vi "2D scan Tclk.vi"(0 "ActiveX Container":refnum<k7>(container), 1 "Det Info":T11={"Brightness A"=40.0, "Contrast A"=26.0, "Detector B name"="ESB @ 1.0 kV", "Brightness B"=40.0, "Contrast B"=40.0, "Detector C name"="PMT @ 6.0", "Detector D name"="Detector D"}, 2 "HW Config":T12={"SEM X coil"="SEM-X", "SEM Y coil"="SEM-Y", "Detectors"="Detectors", "Det min (V)"=-10.0, "Det max (V)"=10.0, "Eanable COM"=TRUE, "COM port"="COM1", "Detector FIB-NI auto switch"="FIB/port0/line0", "Machine Type"=0, "Machine ID"="", "SEM Max FOV (um)"=350.0} {"Machine Type" items=["Feiss", "NVision"]}, 3 "Scan Para":T10={"X resolution"=4096, "Y resolution"=2048, "X center (um)"=0.0, "Y center (um)"=0.0, "X size (V)"=20.0, "X size auto"=TRUE, "X stig"=0.0, "Y stig"=0.0, "X aln"=0.0, "Y aln"=0.0, "Scan rate (Hz)"=10000000, "Oversampling"=10, "Oversampling auto"=TRUE, "Frame line rampdown ratio"=0.1, "Pixel size (nm)"=5.0, "WD"=4.0} {"WD" format="%#_7g"; "Frame line rampdown ratio" min=-1 max=1 step=0.05 format="%.2g"; "Scan rate (Hz)" max=4000000 format="%.2e"}, 4 "Focus Index Options":T2={"Keep aspect ratio"=FALSE, "X Grids"=1, "Y Grids"=1, "Primary X index"=1, "Primary Y index"=1}, 5 "File Info":T8={"File path"=path "E:/Images", "Notes"="", "Save recipe"=FALSE, "Load recipe"=FALSE, "Sample ID"=""}, 6 "Options":T9={"GetInfo"=TRUE, "Set Det A para"=TRUE, "Set WD"=FALSE, "Set Mag"=TRUE, "Set stig"=FALSE, "Set aln"=FALSE, "Display"=TRUE, "Save"=TRUE, "8-bit"=TRUE, "Detector A"=TRUE, "Detector B"=TRUE, "Detector C"=FALSE, "Detector D"=FALSE, "Inverse A"=FALSE, "Inverse B"=FALSE, "Inverse C"=FALSE, "Inverse D"=FALSE, "Inverse PNG"=FALSE, "Freeze"=TRUE, "PNG only"=FALSE, "Upload"=FALSE, "Delete after upload"=FALSE}, 7 "WatchDog Mode":u16(ring)=2 items=["Do Nothing", "Send Idle Only", "Watch FIB & SEM", "Watch FIB Only", "Watch SEM Only"], 9 "Additional Info":cluster{"Restart flag":u8, "Stage move flag":u8}, 10 "Frame":u8=1 min=1 step=1, 11 "Tile index":u8[](array[numeric])=[0, 0], 13 "Milling para":T1={"X resolution"=4096, "Y resolution"=125001, "X offset (um)"=0.0, "Y offset (um)"=0.0, "X center (um)"=0.0, "Y center (um)"=0.0, "X size (um)"=250.0, "Y size (um)"=250.0, "UL-Ang"=90.0, "UR-Ang"=90.0, "Line milling time (s)"=5.0, "Z-step (nm)"=2.0, "Lines auto pause"=1, "Auto pause"=FALSE, "Mill from Bottom"=FALSE, "FIB FOV (um)"=500.0, "Auto Profile"=FALSE, "Mill start from Last"=FALSE, "FIB PID on"=FALSE, "FIB PID reset"=TRUE, "FIB PID measured"=0, "FIB PID target"=0.0, "FIB PID target slope"=0.0, "FIB PID P"=0.001, "FIB PID I"=0.01, "FIB PID D"=0.0, "Emission (uA)"=1.36, "Suppressor (V)"=50.0, "Auto reheat"=FALSE} caption="Milling Parameters" {"Suppressor (V)" step=0.1 format="%.1g"; "Emission (uA)" step=0.1 format="%.2g"; "FIB PID measured" items=["Spec.", "B.D. 1", "B.D. 2", "Mill", "Spec. +"]; "FIB PID target slope" min=-1 max=1 step=0.1; "UR-Ang" format="%.2f"; "UL-Ang" format="%.2f"; "Y offset (um)" step=0.02 format="%.3g"; "X offset (um)" step=1 format="%.3g"; "FIB FOV (um)" format="%.3g"; "Line milling time (s)" format="%.1f"; "Y center (um)" format="%#.3g"; "X center (um)" format="%#.3g"}) -> (12 "Image Focus Index Array":T3, 14 "Info & Status":T7={"AO SampClk.MaxRate"=100000000.0, "AI SampClk.MaxRate"=100000000.0, "AO rate"=10000000.0, "Scan speed"=1, "Detector number"=2, "X min (V)"=-10.0, "X max (V)"=10.0, "X min index"=0, "X max index"=4095, "AO multiline"=128, "Decimating factor"=8, "AvailSampPerChan"=6177088, "AO scan line"=2048, "Total pixels recorded"=8388608, "Total lines scanned"=2048, "Scan time (m)"=0.0, "Scan time (s)"=0.9240575999999999, "Remaining time (m)"=0, "Remaining time (s)"=0, "Specimen I (nA)"=0.0, "Frame"=1, "X tile"=0, "Y tile"=0} {"Frame" min=1 step=1; "Y tile" min=1; "X tile" min=1; "Specimen I (nA)" format="%#.2g"; "AvailSampPerChan" scale=0.0..32000000.0; "Scan time (s)" format="%.3f"; "Total pixels recorded" scale=0.0..250000.0; "Scan speed" scale=1.0..15.0; "AO rate" format="%#_3e"}, 15 "SEM parameters":T5={"Detector A"="Det A", "Detector B"="ESB @ 1.0 kV", "Brightness A"=40.0, "Contrast A"=26.0, "Brightness B"=40.0, "Contrast B"=40.0, "Magnification"=5582.6, "Pixel size"=5.0, "Working distance"=4.0, "EHT"=0.0, "Aperture"=0, "High current mode"=0, "Probe current"=0.0, "Scan rotation"=0.0, "Chamber vac"=0.0, "Gun vac"=0.0, "Beam shift X"=0.0, "Beam shift Y"=0.0, "Stig X"=0.0, "Stig Y"=0.0, "Alignment X"=0.0, "Alignment Y"=0.0, "Stage X"=0.0, "Stage Y"=0.0, "Stage Z"=0.0, "Stage T"=0.0, "Stage R"=0.0, "Stage M"=0.0}, 17 "8-bit over scale":bool[](array[boolean]), 18 "FIB parameters":T6, 19 "Image Focus Index":T4)   [LabVIEW 2018]
uses:
  <vilib>/Utility/error.llb/DialogType.ctl
  <vilib>/DAQmx/write.llb/DAQmx Write (Digital Bool 1Line 1Point).vi
  <vilib>/Analysis/2dsp.llb/Decimate (single shot, DBL).vi
  <vilib>/DAQmx/create/channels.llb/DAQmx Create Channel (DO-Digital Output).vi
  <vilib>/DAQmx/miscellaneous.llb/DAQmx Fill In Error Info.vi
  <instrlib>/niScope/Acquire/niScope Get Scaling Coefficients.vi
  <instrlib>/niScope/Acquire/Fetch/niScope Multi Fetch Binary 16.vi
  <vilib>/measure/madcrms.llb/Basic Averaged DC-RMS for 1 Chan.vi
  <instrlib>/niFgen/niFgen.llb/niFgen Write Waveform.vi
  <vilib>/regexp/Match Regular Expression.xnode
  <vilib>/Analysis/NI_AALPro.lvlib
  <vilib>/measure/NI_MAPro.lvlib
panel:
  out "First pixel Y":i32
  out "First pixel X":i32
  out "Stage move flag":u8
  out "Restart flag":u8
  out "AI multiline":u16
  out "Total pixels":u32
  in  "Force tclk init":bool
  out "DetB-Scaling":sgl
  out "DetA-Scaling":sgl
  out "DetB-Rate":sgl
  out "DetA-Rate":sgl
  out "8-bit coefficents":sgl[][](array[numeric])
  out "DetB-k":sgl
  out "DetB-Io":sgl
  out "DetA-k":sgl
  out "DetA-Io":sgl
  out "8-bit":bool=TRUE
  out "Screen pixel factor":dbl=0.25
  out "Mag":dbl=5582.6
  out "Runsheet header array":string[](array[string])=["Date", "Time", "Notes", "Detector A", "Detector B", "Detector C", "Detector D", "Detectors", "X resolution", "Y resolution", "Rate (Hz)", "Brightness A (%)", "Contrast A (%)", "Brightness B (%)", "Contrast B (%)", "Magnification", "Pixel size (nm)", "Working Distance (mm)", "EHT (kV)", "Aperture #", "High Current Mode", "Probe Current (A)", "Beam Shift X", "Beam Shift Y", "Stigmation X", "Stigmation Y", "Alignment X", "Alignment Y", "FIB spacing (nm)", "A Img Focus Index", "B Img Focus Index", "C Img Focus Index", "D Img Focus Index", "Temp (F)", "FIB Faraday Cup (nA)", "Specimen I (nA)", "Milling Beam Dump (nA)", "Milling Y voltage (V)", "SEM Specimen I (nA)", "Image Delta X (pix)", "Image Delta Y (pix)", "Image Delta Z"]
  out "Set aln":bool
  out "X aln":sgl
  out "Y aln":sgl
  out "FI scaling":u8=1
  in  "SEM Spec. I (nA)":sgl format="%#.2g"
  out "SW date":string
  out "Image bits":u8=16
  out "error out":errorcluster
  out "Delete after upload":bool
  in  "FI Detector":u16(ring) caption="Detector" items=["A", "B", "C", "D"]
  out "keep aspect ratio":bool=TRUE
  out "Primary Y index":u8 caption="Primary Y"
  out "Primary X index":u8 caption="Primary X"
  out "Y Grids":u8=1
  out "X Grids":u8=1
  out "Timestamp":timestamp=timestamp(3479292891.7167473 s since 1904-01-01)
  out "Upload flags path":path
  out "Upload":bool=TRUE
  out "Sample ID":string
  out "Machine ID":string
  out "Eanable COM":bool
  out "PNG only":bool=TRUE
  out "Eval B":i16[][](graph)
  out "Eval A":i16[][](graph)
  out "Freeze":bool=TRUE
  out "Detector FIB-NI auto switch":tag="FIB/port0/line0"
  out "GetInfo":bool=TRUE
  out "Set stig":bool
  out "Y stig":sgl
  out "X stig":sgl
  in  "Total time":dbl=0.9240575999999999
  in  "stop":bool=TRUE
  out "Det max (V)":dbl=10.0
  out "Det min (V)":dbl=-10.0
  in  "AvailSampPerChan":u32(slide)=6177088 scale=0.0..1000000.0
  in  "AO scan line":u32=2048
  in  "AO multiline":u32=128
  in  "Decimating factor":u16=8
  in  "Remaining time (m)":u16
  in  "Remaining time (s)":u8
  in  "Scan time (s)":dbl=0.9240575999999999 format="%.3f"
  in  "Scan time (m)":dbl
  in  "Total lines scanned":i32=2048
  in  "Total pixels recorded":i32(slide)=8388608 scale=-1.0..1048576.0
  in  "X max (V)":dbl=10.0
  in  "X min (V)":dbl=-10.0
  in  "X min index":i32
  in  "X max index":i32=4095
  in  "Scan speed":u8(slide)=1 scale=1.0..15.0
  in  "AO rate":dbl=10000000.0 caption="Scanning rate" format="%#_3e"
  in  "Detector number":u8=2
  in  "AI SampClk.MaxRate":dbl=100000000.0
  in  "AO SampClk.MaxRate":dbl=100000000.0
  out "Det A Img":i16[][](graph)
  out "Det B Img":i16[][](graph)
  out "Notes":string
  out "File path":path=path "E:/Images"
  out "Inverse PNG":bool
  out "Inverse D":bool
  out "Inverse C":bool
  out "Inverse B":bool
  out "Inverse A":bool
  out "Detector D":bool
  out "Detector C":bool
  out "Detector B":bool=TRUE
  out "Detector A":bool=TRUE
  out "Save":bool=TRUE
  out "Display":bool=TRUE
  out "Set Mag":bool=TRUE
  out "Set WD":bool
  out "Set Det A para":bool=TRUE
  out "WD":sgl=4.0
  out "Pixel size (nm)":sgl=5.0
  out "Frame line rampdown ratio":sgl=0.1
  out "Oversampling":u32=10
  out "Scan rate (Hz)":u32=10000000
  out "Y resolution":u32=2048
  out "X resolution":u32=4096
  out "Detector D name":string="Detector D"
  out "Detector C name":string="PMT @ 6.0"
  out "Contrast B":dbl=40.0
  out "Brightness B":dbl=40.0
  out "Detector B name":string="ESB @ 1.0 kV"
  out "Contrast A":dbl=26.0
  out "Brightness A":dbl=40.0
  out "COM port":refnum<visa-resource-name>="COM1"
  out "File name":path=path "E:/Images/Y2014/M04/D02/_14-04-02_091451_0-0.dat"
  # "Hardware Configuration"
  # "Detectors Information"
  # "Scanning Parameters"
  # "Direction"
  # "Start\nfrom"
  # "<"
  # "Hz"
  # "Scanning time"
  # "m"
  # "s"
  # "Remaining time"
  # "m"
  # "s"
  # "Det"
  # "Detector A"
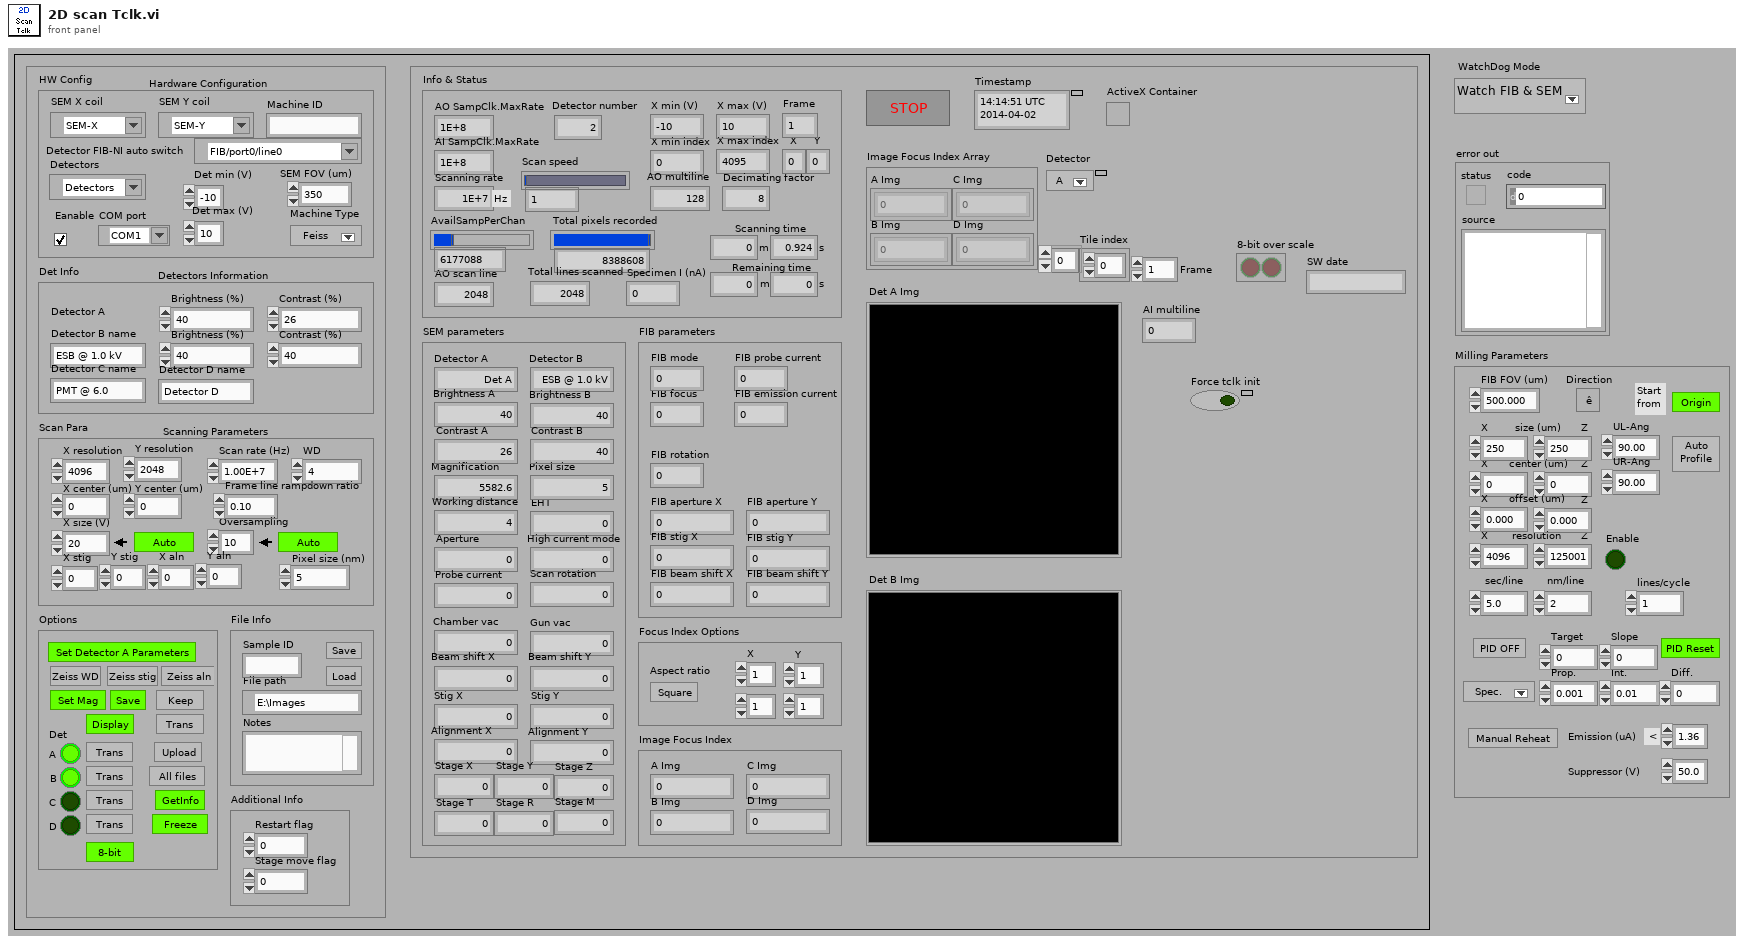
[diagram p1: front panel]
types:
  T1 = cluster{"X resolution":u32, "Y resolution":u32, "X offset (um)":sgl, "Y offset (um)":sgl, "X center (um)":sgl, "Y center (um)":sgl, "X size (um)":sgl, "Y size (um)":sgl, "UL-Ang":sgl, "UR-Ang":sgl, "Line milling time (s)":sgl, "Z-step (nm)":dbl, "Lines auto pause":u16, "Auto pause":bool, "Mill from Bottom":bool, "FIB FOV (um)":sgl, "Auto Profile":bool, "Mill start from Last":bool, "FIB PID on":bool, "FIB PID reset":bool, "FIB PID measured":u8, "FIB PID target":sgl, "FIB PID target slope":sgl, "FIB PID P":sgl, "FIB PID I":sgl, "FIB PID D":sgl, "Emission (uA)":dbl, "Suppressor (V)":sgl, "Auto reheat":bool}
  T2 = cluster{"Keep aspect ratio":bool, "X Grids":u8, "Y Grids":u8, "Primary X index":u8, "Primary Y index":u8}
  T3 = cluster{"A Img Focus Index array":sgl[][], "B Img Focus Index array":sgl[][], "C Img Focus Index array":sgl[][], "D Img Focus Index array":sgl[][]}
  T4 = cluster{"A Img Focus Index":sgl, "B Img Focus Index":sgl, "C Img Focus Index":sgl, "D Img Focus Index":sgl}
  T5 = cluster{"Detector A":string, "Detector B":string, "Brightness A":sgl, "Contrast A":sgl, "Brightness B":sgl, "Contrast B":sgl, "Magnification":sgl, "Pixel size":sgl, "Working distance":sgl, "EHT":sgl, "Aperture":u8, "High current mode":u8, "Probe current":sgl, "Scan rotation":sgl, "Chamber vac":sgl, "Gun vac":sgl, "Beam shift X":sgl, "Beam shift Y":sgl, "Stig X":sgl, "Stig Y":sgl, "Alignment X":sgl, "Alignment Y":sgl, "Stage X":sgl, "Stage Y":sgl, "Stage Z":sgl, "Stage T":sgl, "Stage R":sgl, "Stage M":sgl}
  T6 = cluster{"FIB mode":u8, "FIB focus":sgl, "FIB probe current":sgl, "FIB emission current":sgl, "FIB rotation":sgl, "FIB aperture X":sgl, "FIB aperture Y":sgl, "FIB stig X":sgl, "FIB stig Y":sgl, "FIB beam shift X":sgl, "FIB beam shift Y":sgl}
  T7 = cluster{"AO SampClk.MaxRate":dbl, "AI SampClk.MaxRate":dbl, "AO rate":dbl, "Scan speed":u8, "Detector number":u8, "X min (V)":dbl, "X max (V)":dbl, "X min index":i32, "X max index":i32, "AO multiline":u32, "Decimating factor":u16, "AvailSampPerChan":u32, "AO scan line":u32, "Total pixels recorded":i32, "Total lines scanned":i32, "Scan time (m)":dbl, "Scan time (s)":dbl, "Remaining time (m)":u16, "Remaining time (s)":u8, "Specimen I (nA)":sgl, "Frame":u8, "X tile":u8, "Y tile":u8}
  T8 = cluster{"File path":path, "Notes":string, "Save recipe":bool, "Load recipe":bool, "Sample ID":string}
  T9 = cluster{"GetInfo":bool, "Set Det A para":bool, "Set WD":bool, "Set Mag":bool, "Set stig":bool, "Set aln":bool, "Display":bool, "Save":bool, "8-bit":bool, "Detector A":bool, "Detector B":bool, "Detector C":bool, "Detector D":bool, "Inverse A":bool, "Inverse B":bool, "Inverse C":bool, "Inverse D":bool, "Inverse PNG":bool, "Freeze":bool, "PNG only":bool, "Upload":bool, "Delete after upload":bool}
  T10 = cluster{"X resolution":u32, "Y resolution":u32, "X center (um)":sgl, "Y center (um)":sgl, "X size (V)":dbl, "X size auto":bool, "X stig":sgl, "Y stig":sgl, "X aln":sgl, "Y aln":sgl, "Scan rate (Hz)":u32, "Oversampling":u32, "Oversampling auto":bool, "Frame line rampdown ratio":sgl, "Pixel size (nm)":sgl, "WD":sgl}
  T11 = cluster{"Brightness A":dbl, "Contrast A":dbl, "Detector B name":string, "Brightness B":dbl, "Contrast B":dbl, "Detector C name":string, "Detector D name":string}
  T12 = cluster{"SEM X coil":refnum<k15>, "SEM Y coil":refnum<k15>, "Detectors":refnum<k15>, "Det min (V)":dbl, "Det max (V)":dbl, "Eanable COM":bool, "COM port":refnum<visa-resource-name>, "Detector FIB-NI auto switch":tag, "Machine Type":u8, "Machine ID":string, "SEM Max FOV (um)":sgl}
  T13 = cluster{"AO SampClk.MaxRate":dbl, "AI SampClk.MaxRate":dbl, "AO rate":dbl, "Scan speed":u8, "Detector number":u8, "X min (V)":dbl, "X max (V)":dbl, "X min index":i32, "X max index":i32, "AO multiline":u32, "Decimating factor":u16, "AvailSampPerChan":u32, "AO scan line":u32, "Total pixels recorded":i32, "Total lines scanned":i32, "Scan time (m)":dbl, "Scan time (s)":dbl, "Remaining time (m)":u16, "Remaining time (s)":u8, "SEM Spec. I (nA)":sgl, "Frame":u8, u8, u8}
  T14 = enum16{"SEM", "FIB", "Milling", "SEM + FIB", "Mill + SEM", "SEM Drift Correction", "FIB Drift Correction", "No Beam", "External", "External + SEM"}
  T15 = enum16{"Initialize Reference", "Get Reference", "Close Reference"}
  T16 = enum16{"open", "replace", "create", "open or create", "replace or create", "replace or create with confirmation"}
  T17 = typedef "DialogType.ctl" = u16
  T18 = cluster{"FIB mode":u8, "FIB focus":sgl, "FIB probe current":u8, "FIB emission current":sgl, "FIB rotation":sgl, "FIB aperture X":sgl, "FIB aperture Y":sgl, "FIB stig X":sgl, "FIB stig Y":sgl, "FIB beam shift X":sgl, "FIB beam shift Y":sgl}
  T19 = cluster{"Latest 8-bit coefficients[0]":sgl, "Latest 8-bit coefficients[1]":sgl, "Latest 8-bit coefficients[2]":sgl, "Latest 8-bit coefficients[3]":sgl, "Latest 8-bit coefficients[4]":sgl, "Latest 8-bit coefficients[5]":sgl, "Latest 8-bit coefficients[6]":sgl, "Latest 8-bit coefficients[7]":sgl}
  T20 = cluster{"sessions out":refnum<k20>[], "SEM-X handle out":refnum<k15>, "SEM-Y handle out":refnum<k15>, "SEM-Y waveform handle out":i32, "Detectors handle out":refnum<k15>, "channels":string, "error out":errorcluster, "Others":cluster{"AO SampClk.MaxRate":dbl, "AI SampClk.MaxRate":dbl, "AO rate":dbl, "Scan speed":u8, "Detector number":u8, "X min (V)":dbl, "X max (V)":dbl, "X min index":i32, "X max index":i32, "Y min (V)":dbl, "Y max (V)":dbl, "AO multiline":u32, "Decimating factor":u16, "Total time":dbl, "Scan time (m)":dbl, "Scan time (s)":dbl, "X resolution":u32, "Y resolution":u32, "X resolution with rampdown":i32, "Oversampling":u32, "Y scan pts per line":i32, "Y scan pts per AO multiline":i32, "Small scan":bool, "Y single line pattern":dbl[], "Detectors min record length":u32, "Waveform blocks":u32, "Repeat count":u32, "Waveform size":u32, "AI multiline":u16}}
  T21 = cluster{"offset":dbl, "gain":dbl, "reserved 1":dbl, "reserved 2":dbl}[]
  T22 = cluster{"offset":sgl, "gain":sgl, "reserved 1":sgl, "reserved 2":sgl}[]
  T23 = cluster{"Detector A":bool, "Detector B":bool, "Detector C":bool, "Detector D":bool}
  T24 = cluster{"Detector C name":string, "Detector D name":string}
  T25 = cluster{"X resolution":u32, "Y resolution":u32, "Oversampling":u32, "Scan speed":u8, "AO rate":dbl, "Frame line rampdown ratio":sgl, "X min (V)":dbl, "X max (V)":dbl, "Det min (V)":dbl, "Det max (V)":dbl}
  T26 = cluster{"X resolution":u32, "Y resolution":u32, "X index":u32[], "Y index":u32[], "X length":u32, "Y length":u32}
  T27 = cluster{"A Img Focus Index array":dbl[][], "B Img Focus Index array":dbl[][], "C Img Focus Index array":dbl[][], "D Img Focus Index array":dbl[][]}
  T28 = cluster{"A Img Focus Index":dbl, "B Img Focus Index":dbl, "C Img Focus Index":dbl, "D Img Focus Index":dbl}
  T29 = cluster{"Single":sgl, "Single":sgl, "Single":sgl, "Single":sgl, "Single":sgl, "Single":sgl, "SEM Spec. I (nA)":sgl, "Single":sgl, "D Img Focus Index":dbl, "UInt32":u32}
  T30 = cluster{dbl, "8-bit":bool, "8-bit coefficents":sgl[][], "Restart flag":u8, "Stage move flag":u8, "First pixel X":i32, "First pixel Y":i32, cluster{"Detector A":bool, "Detector B":bool, "Detector C":bool, "Detector D":bool}, cluster{"X resolution":u32, "Y resolution":u32, "Oversampling":u32, "Scan speed":u8, "AO rate":dbl, "Frame line rampdown ratio":sgl, "X min (V)":dbl, "X max (V)":dbl, "Det min (V)":dbl, "Det max (V)":dbl}, "Decimating factor":u16, "Sample ID":string, "Notes":string, cluster{"Detector C name":string, "Detector D name":string}, "SEM parameters":cluster{"Detector A":string, "Detector B":string, "Brightness A":sgl, "Contrast A":sgl, "Brightness B":sgl, "Contrast B":sgl, "Magnification":sgl, "Pixel size":sgl, "Working distance":sgl, "EHT":sgl, "Aperture":u8, "High current mode":u8, "Probe current":sgl, "Scan rotation":sgl, "Chamber vac":sgl, "Gun vac":sgl, "Beam shift X":sgl, "Beam shift Y":sgl, "Stig X":sgl, "Stig Y":sgl, "Alignment X":sgl, "Alignment Y":sgl, "Stage X":sgl, "Stage Y":sgl, "Stage Z":sgl, "Stage T":sgl, "Stage R":sgl, "Stage M":sgl}, "FIB parameters":cluster{"FIB mode":u8, "FIB focus":sgl, "FIB probe current":sgl, "FIB emission current":sgl, "FIB rotation":sgl, "FIB aperture X":sgl, "FIB aperture Y":sgl, "FIB stig X":sgl, "FIB stig Y":sgl, "FIB beam shift X":sgl, "FIB beam shift Y":sgl}, "Milling para":cluster{"X resolution":u32, "Y resolution":u32, "X offset (um)":sgl, "Y offset (um)":sgl, "X center (um)":sgl, "Y center (um)":sgl, "X size (um)":sgl, "Y size (um)":sgl, "UL-Ang":sgl, "UR-Ang":sgl, "Line milling time (s)":sgl, "Z-step (nm)":dbl, "Lines auto pause":u16, "Auto pause":bool, "Mill from Bottom":bool, "FIB FOV (um)":sgl, "Auto Profile":bool, "Mill start from Last":bool, "FIB PID on":bool, "FIB PID reset":bool, "FIB PID measured":u8, "FIB PID target":sgl, "FIB PID target slope":sgl, "FIB PID P":sgl, "FIB PID I":sgl, "FIB PID D":sgl, "Emission (uA)":dbl, "Suppressor (V)":sgl, "Auto reheat":bool}, "Machine ID":string, cluster{"Single":sgl, "Single":sgl, "Single":sgl, "Single":sgl, "Single":sgl, "Single":sgl, "SEM Spec. I (nA)":sgl, "Single":sgl, "D Img Focus Index":dbl, "UInt32":u32}}
  T31 = typedef "imagedata.ctl" = cluster{"image type":i32, "image depth":i32, "image":u8[], "mask":u8[], "colors":u32[], "Rectangle":cluster{"left":i16, "top":i16, "right":i16, "bottom":i16}}
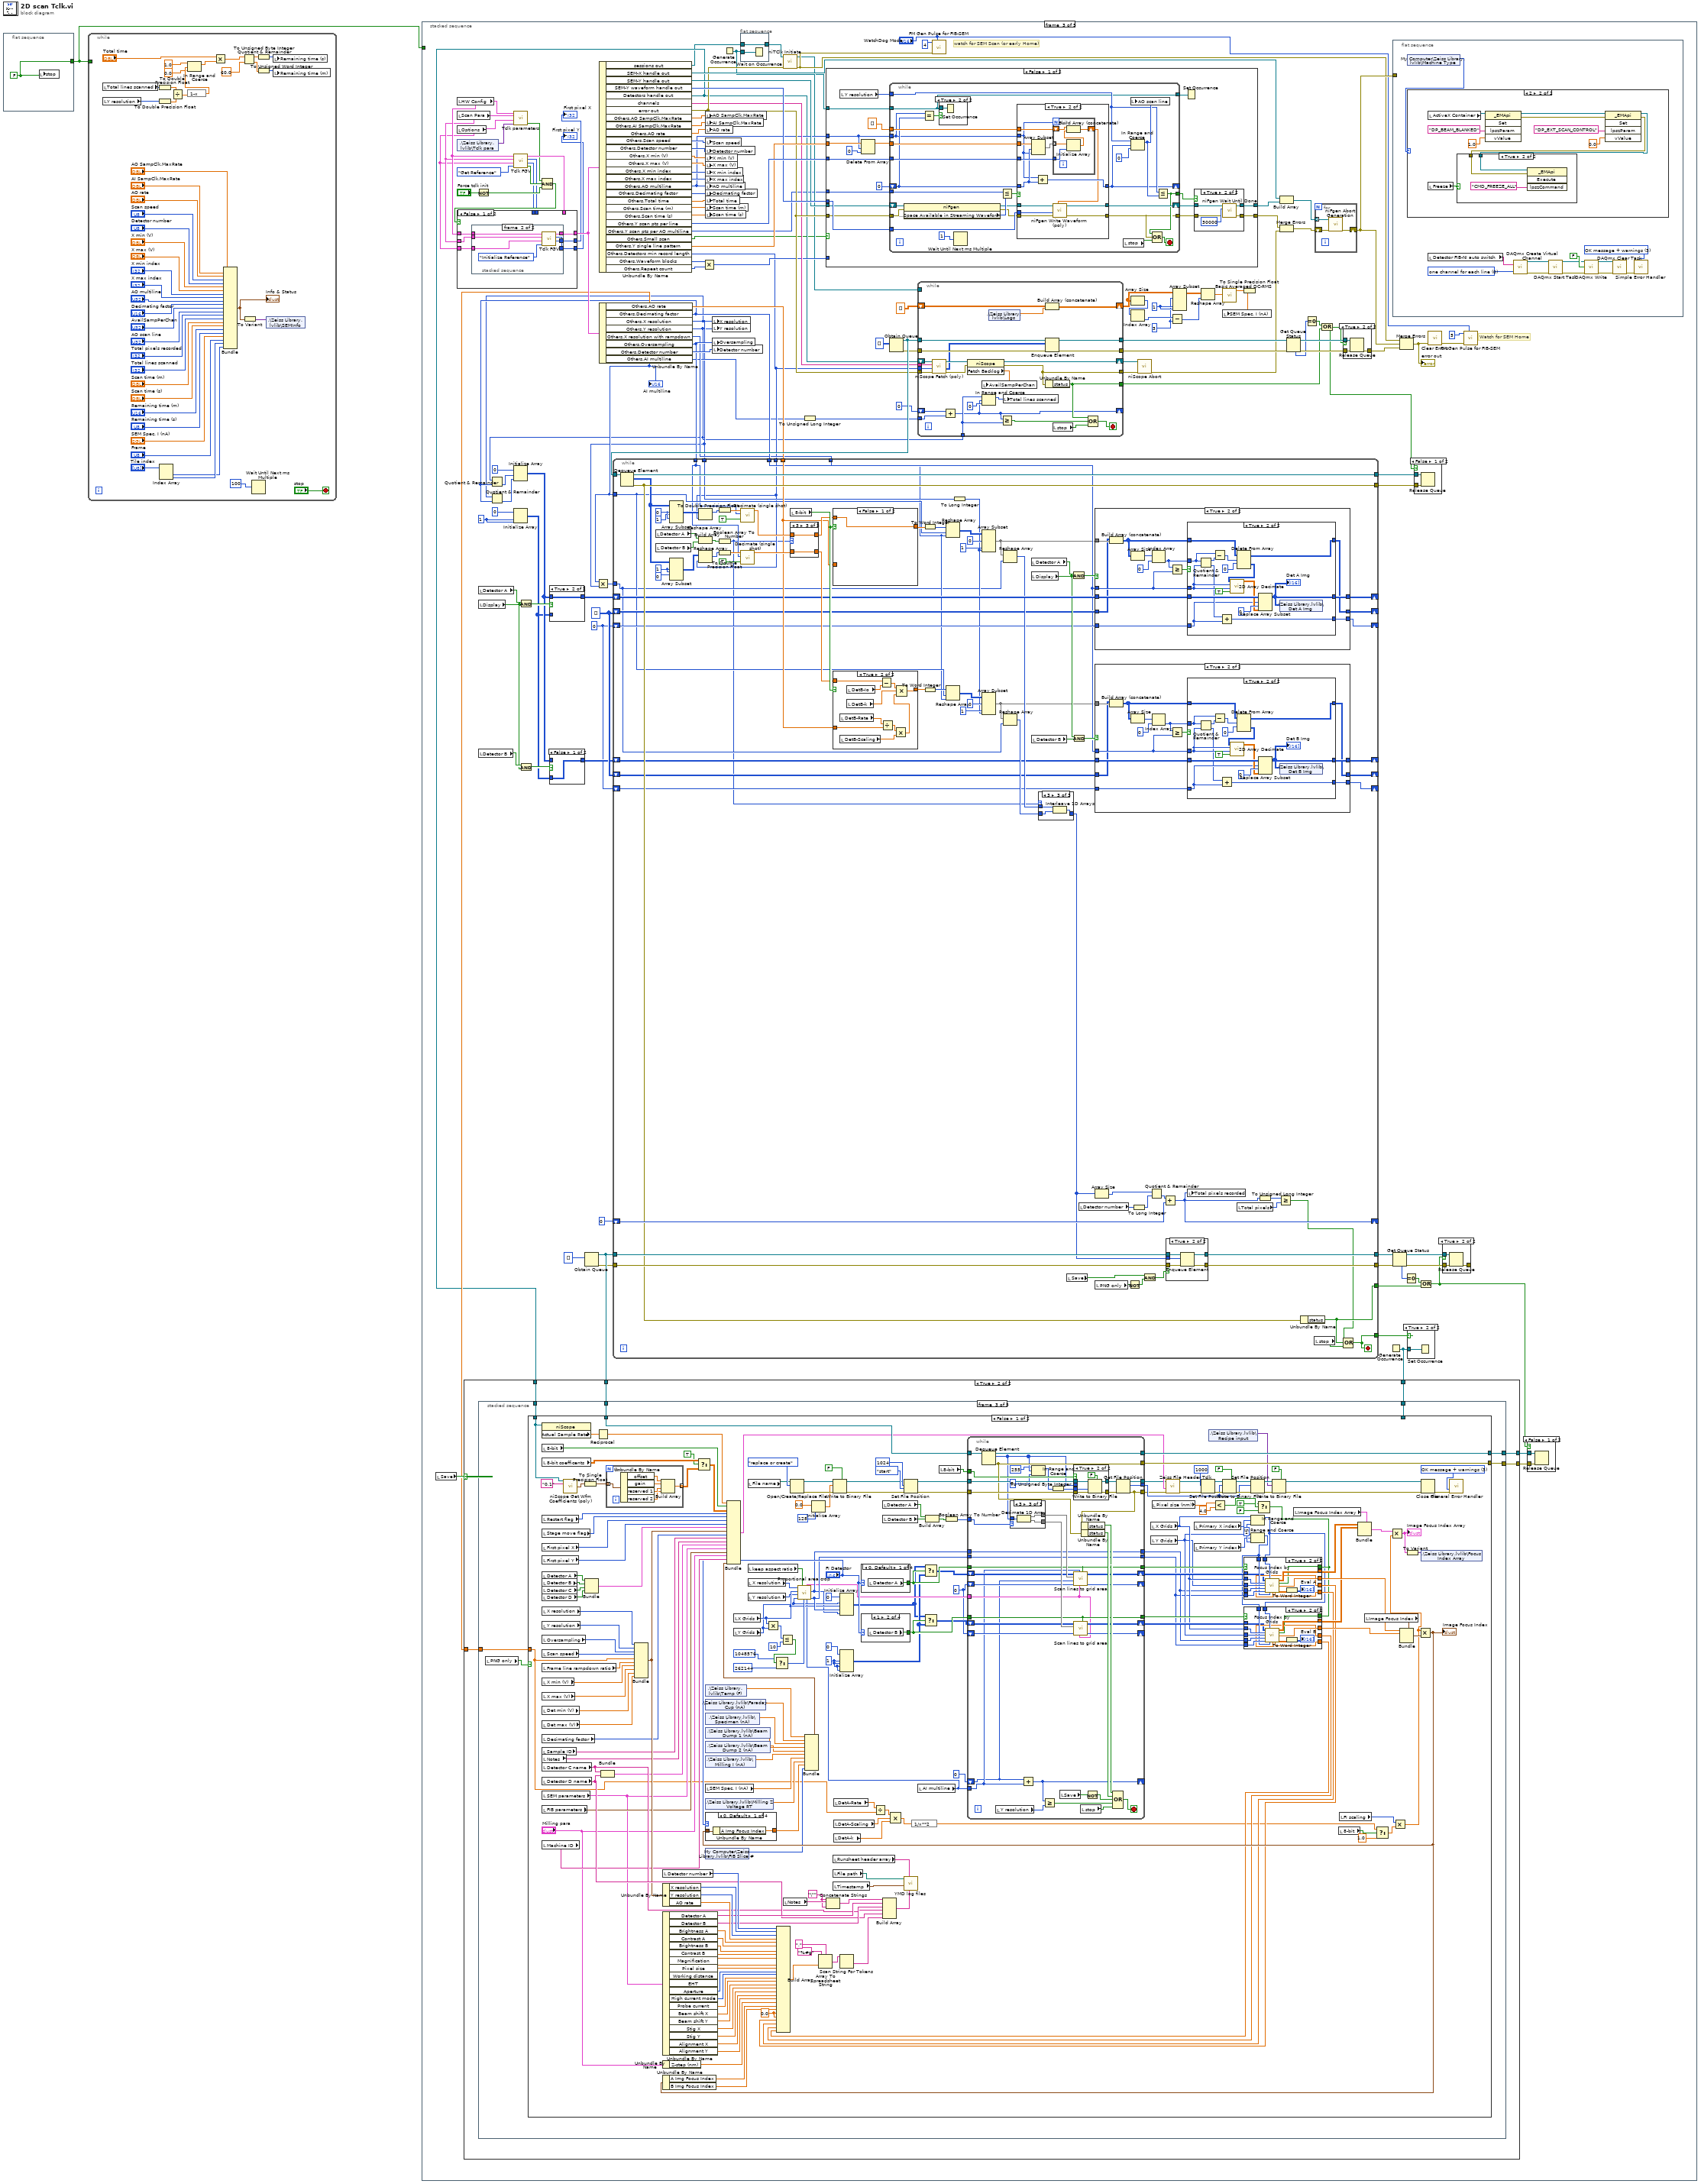
[diagram p0: block diagram]
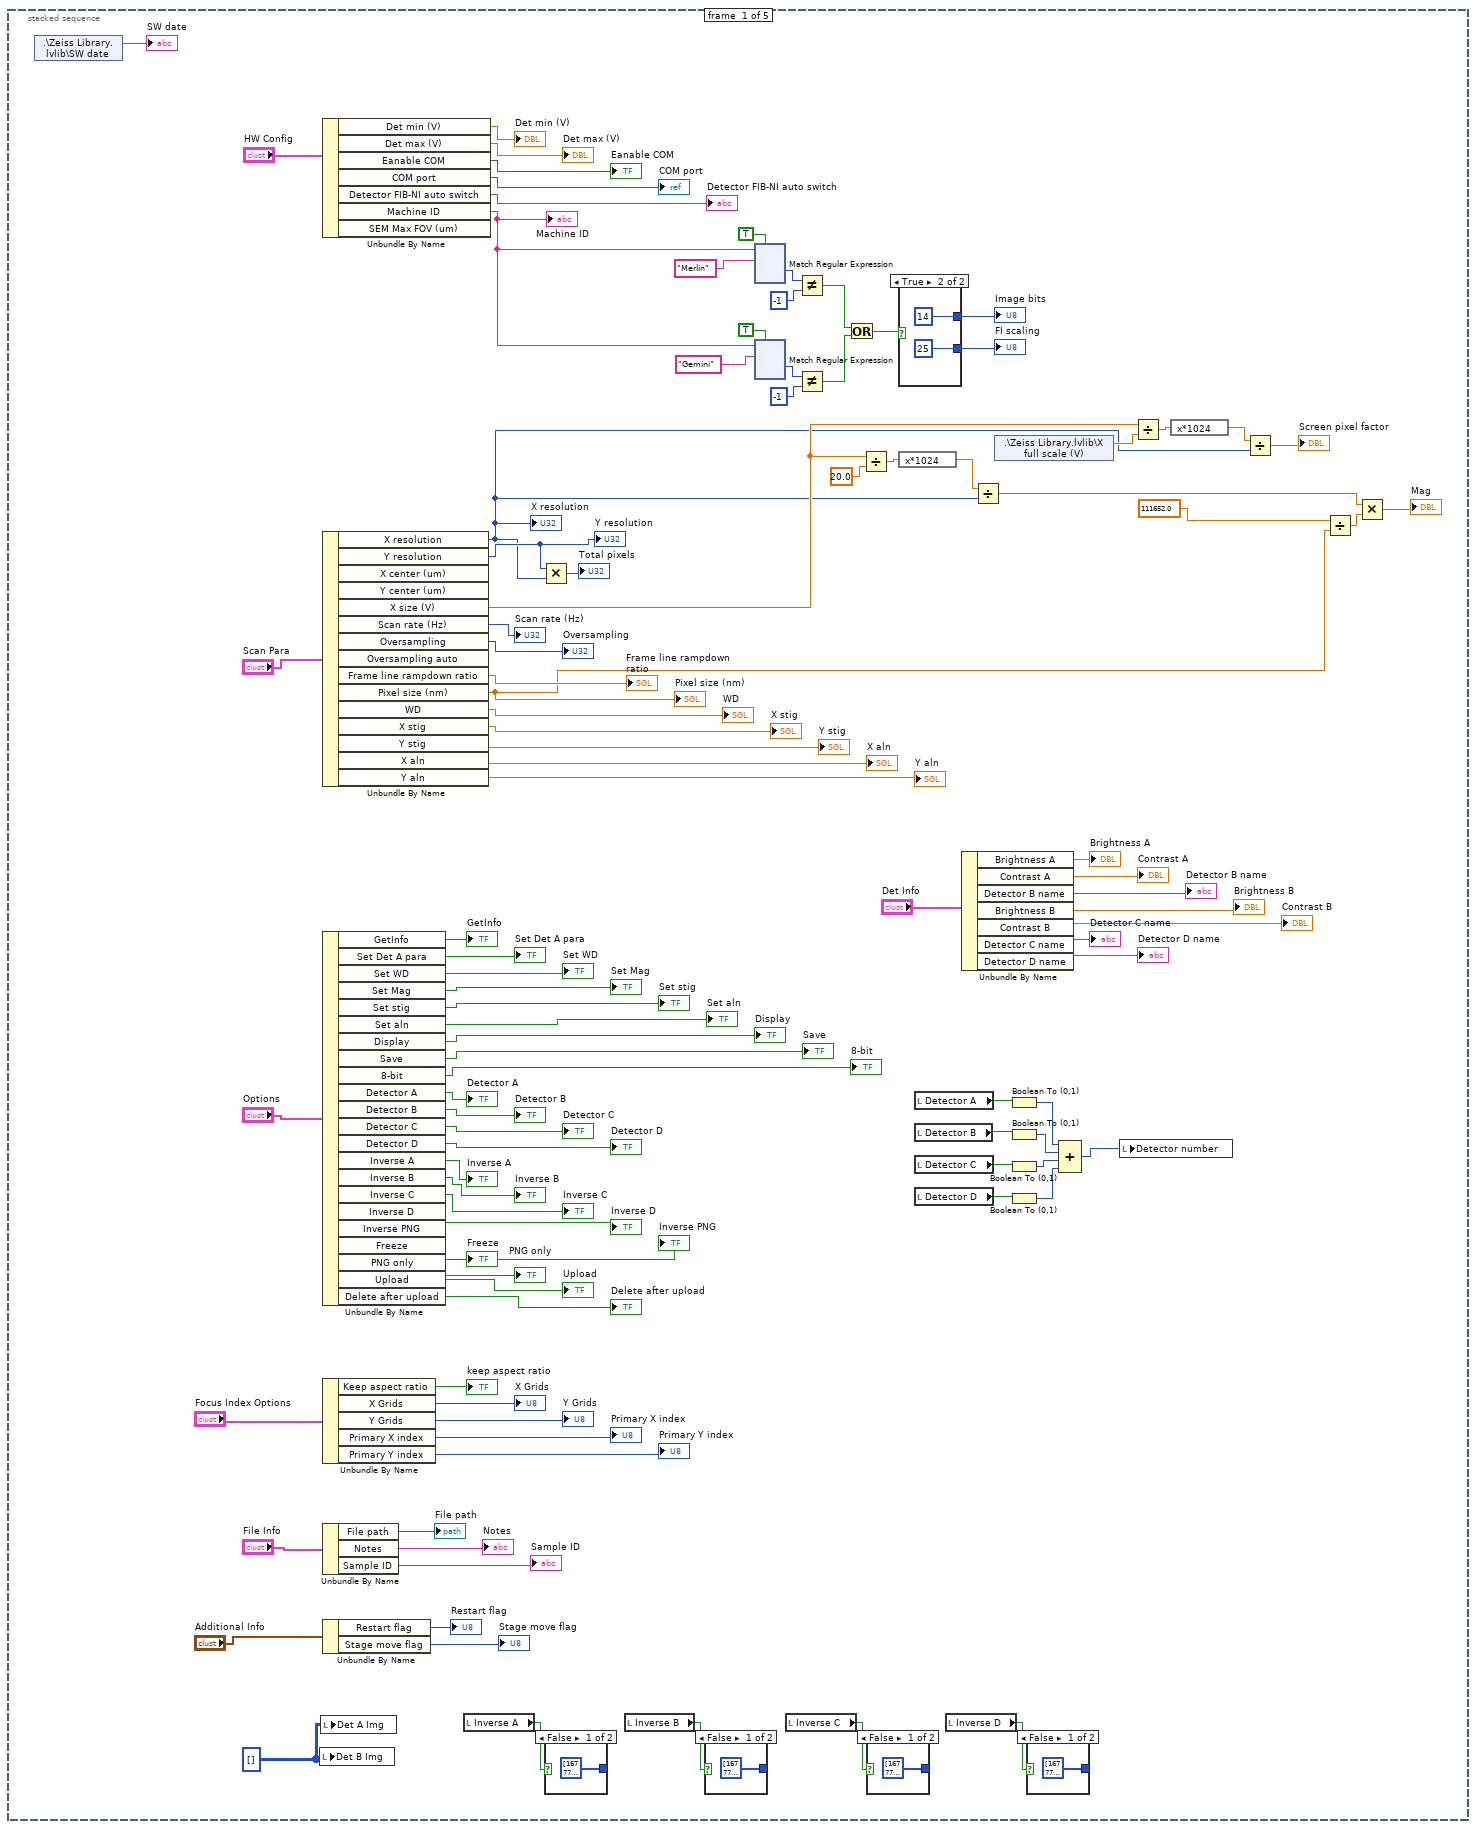
[diagram p2: hidden frame]
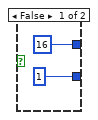
[diagram p3: hidden frame]
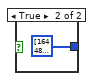
[diagram p4: hidden frame]
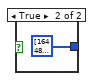
[diagram p5: hidden frame]
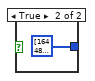
[diagram p6: hidden frame]
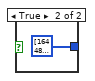
[diagram p7: hidden frame]
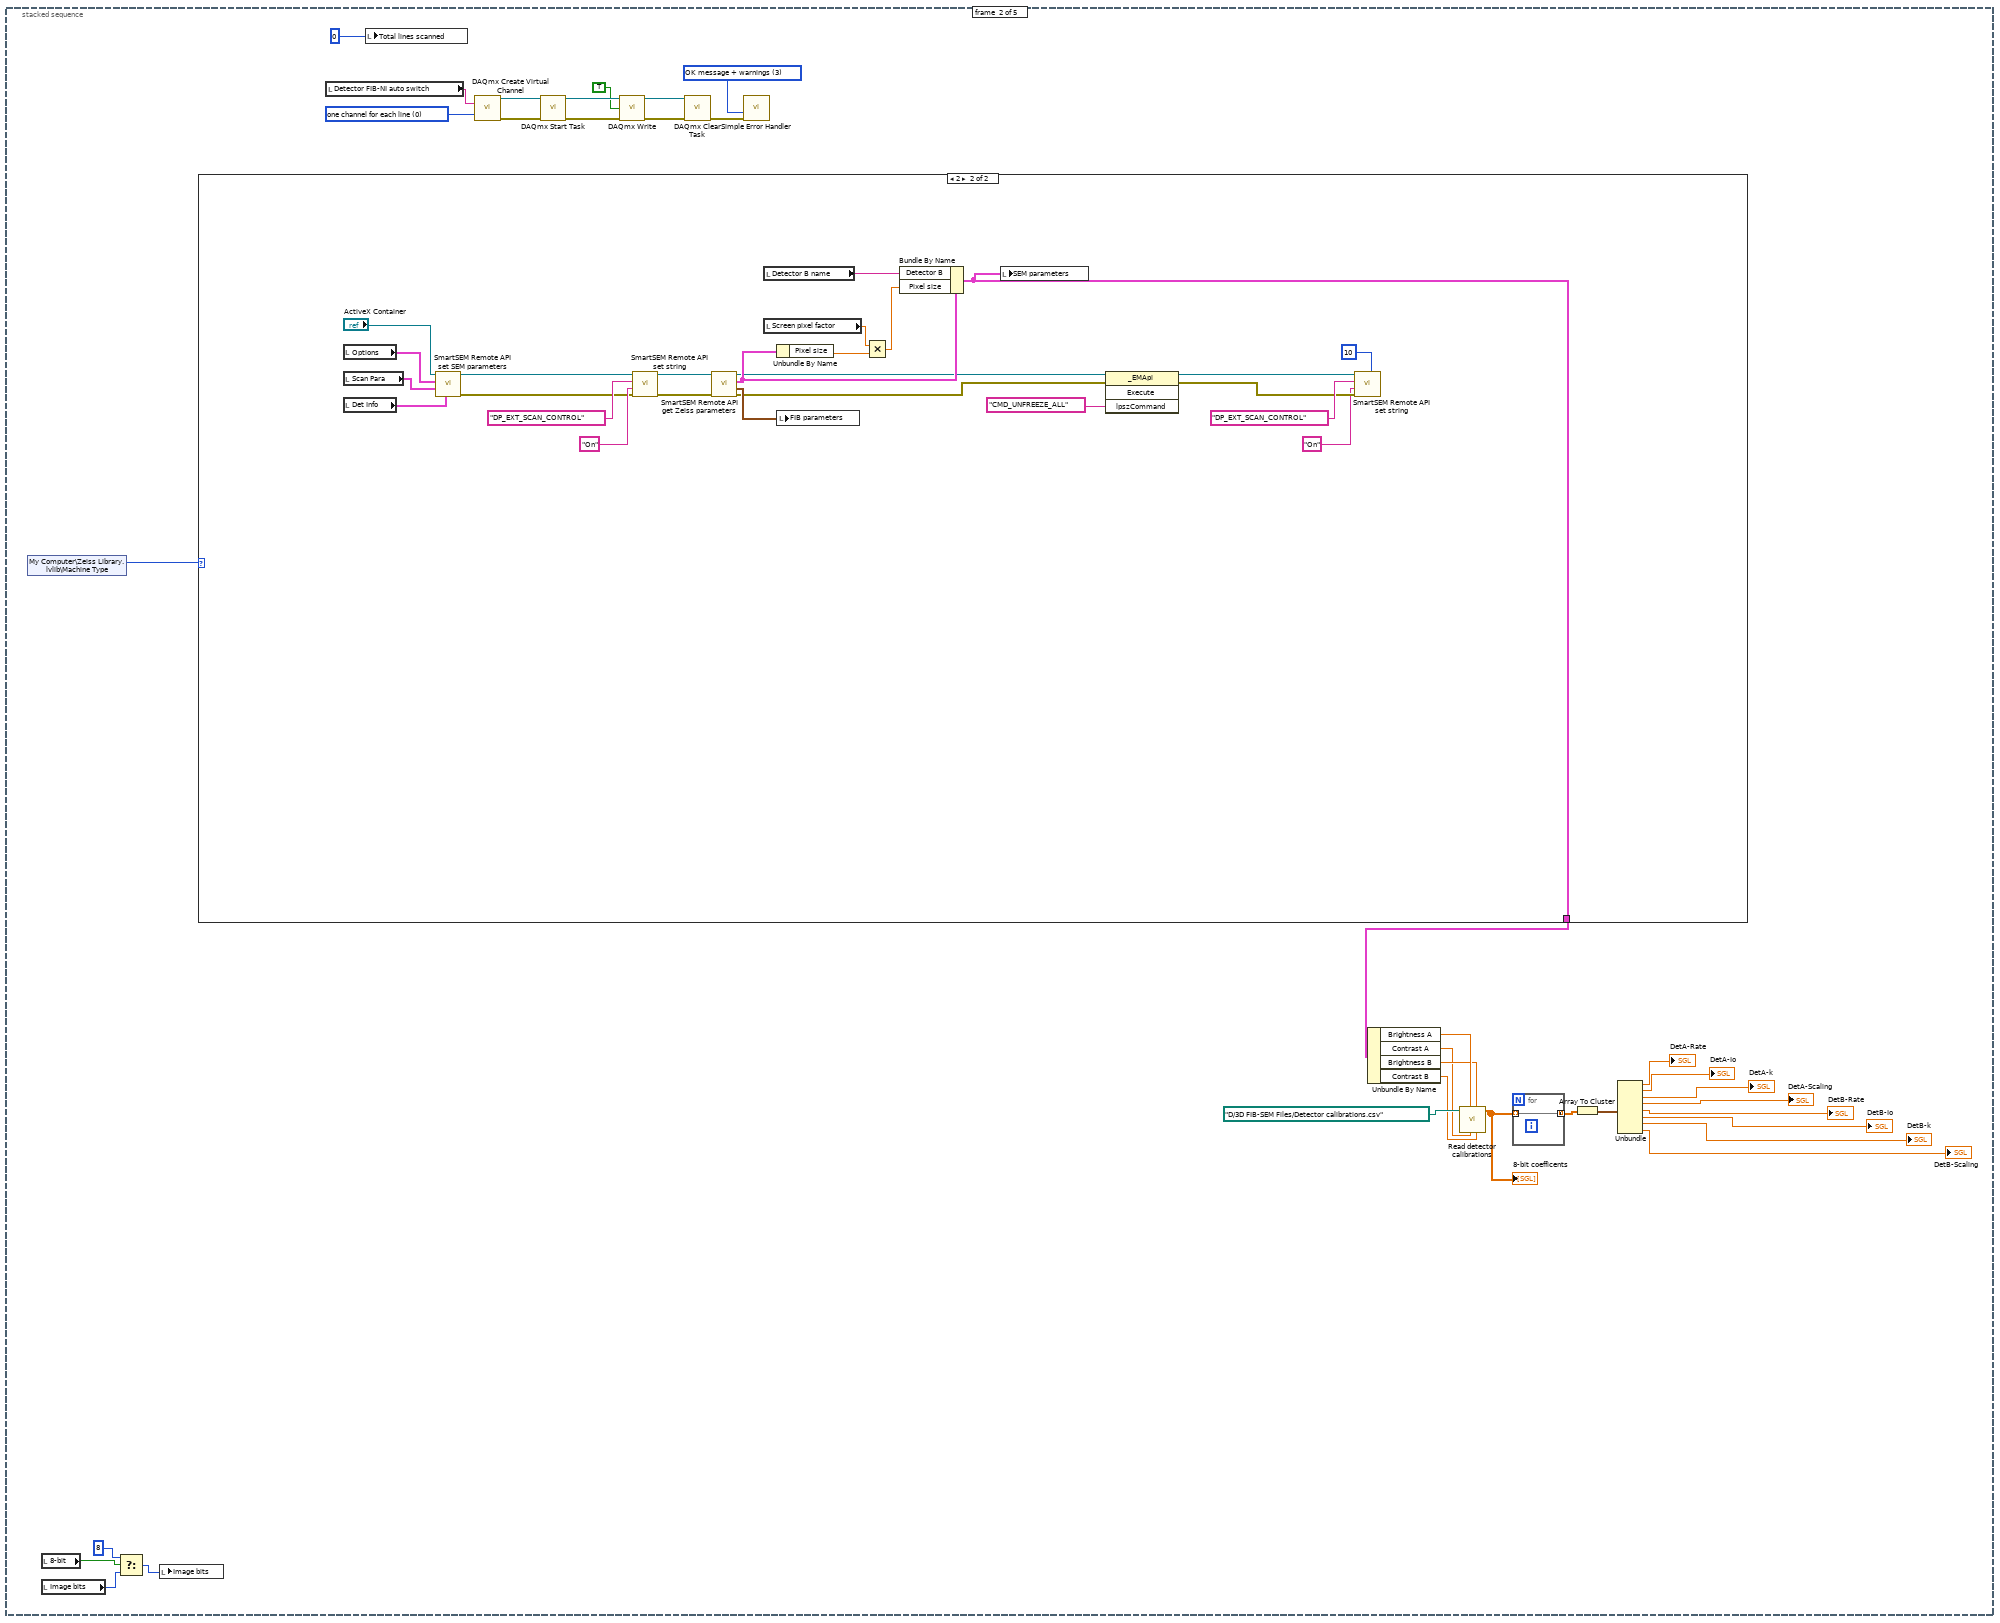
[diagram p8: hidden frame]
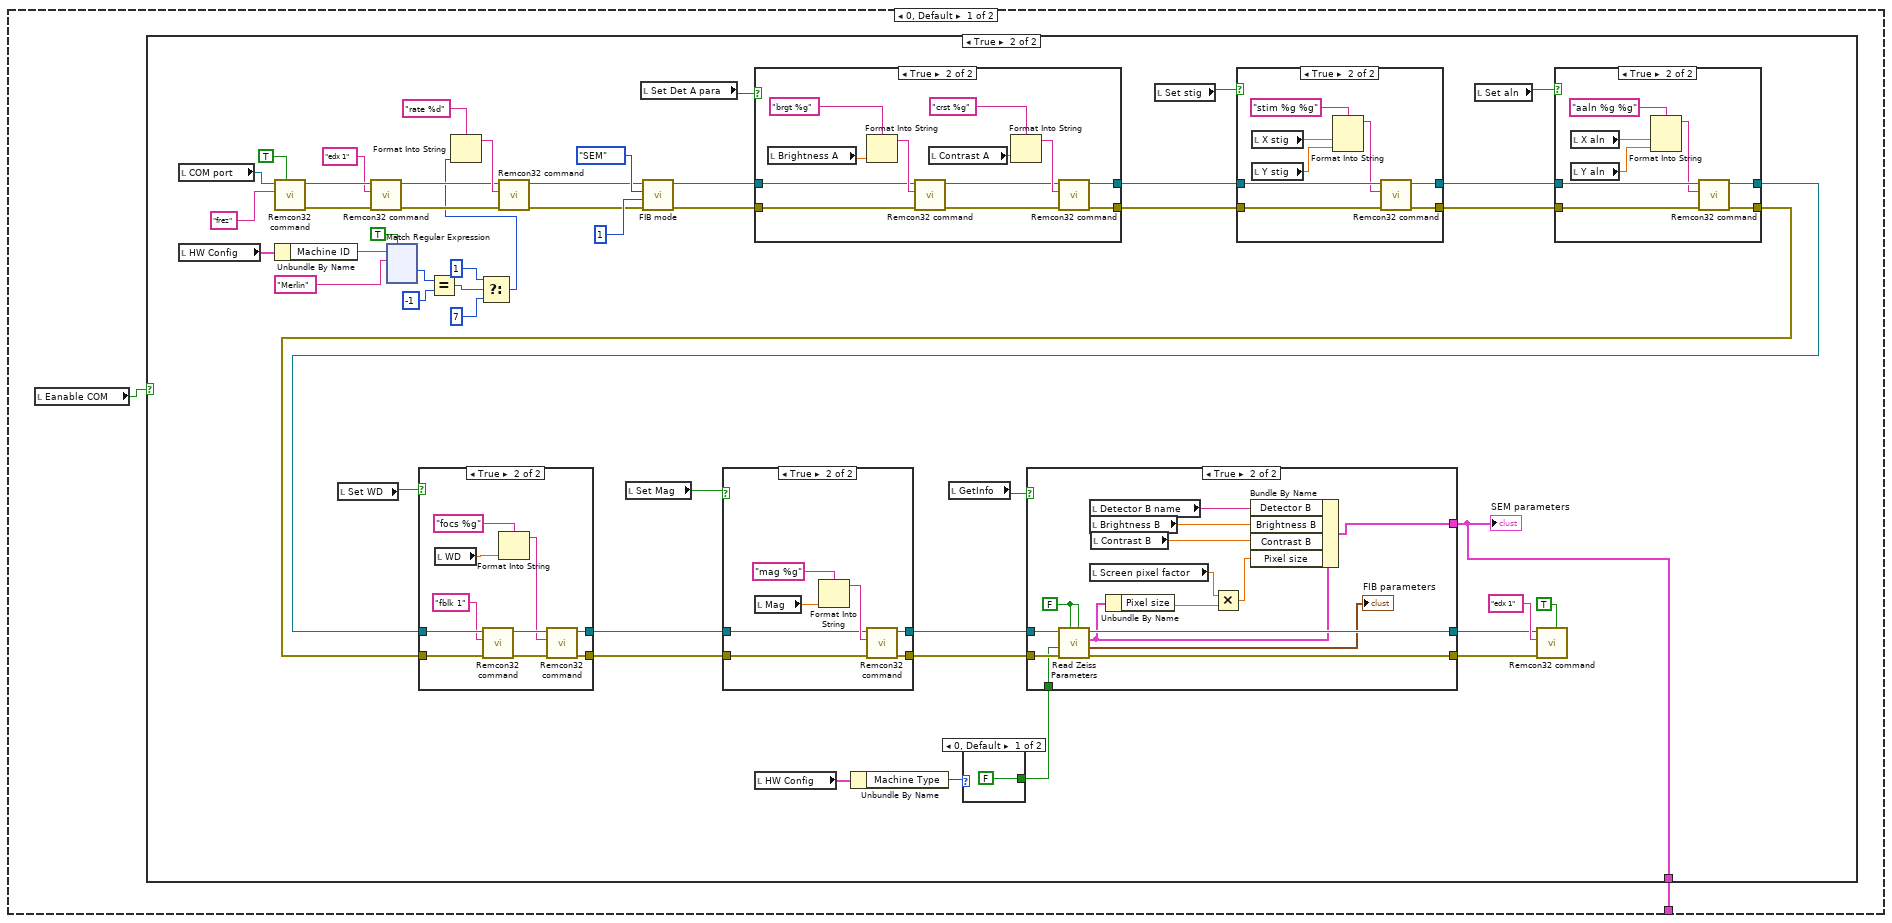
[diagram p9: hidden frame]
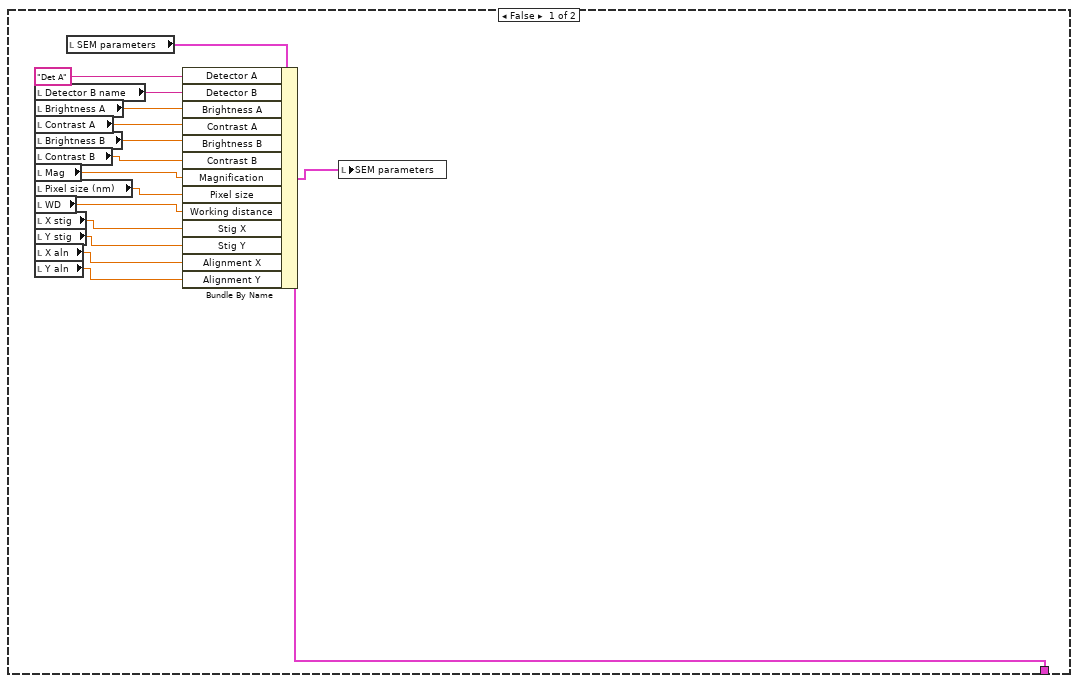
[diagram p10: hidden frame]
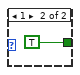
[diagram p12: hidden frame]
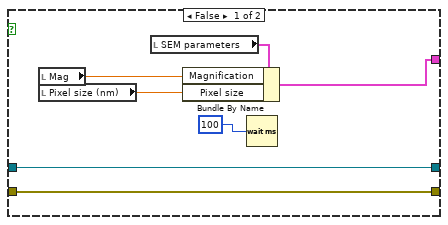
[diagram p13: hidden frame]
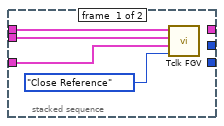
[diagram p19: hidden frame]
diagram:
  n1 = flat-sequence {
    tunnel: [w2] -> w1
    frame #0 {
      w2 = FALSE ("stop")
      n2 = local write "stop"(w2) -> ()
    }
  }
  n3 = while {
    tunnel: w1 -> [_]
    stop <- "stop" stop-if-true
    n4 = local read "Total lines scanned"() -> (w27:i32)
    n5 = local read "Y resolution"() -> (w16:u32)
    n6 = To Double Precision Float(number=w27) -> (double precision float=w20:dbl)
    n7 = To Double Precision Float(number=w16) -> (double precision float=w21:dbl)
    n8 = Index Array(array="Tile index") -> (element #1=w6:u8, element #2=w7:u8)  [unwired: 2 in]
    n9 = Divide(x=w20, y=w21) -> (x/y=w26:dbl)
    n10 = expression code="1-x"(w26) -> (w13:dbl)
    n11 = In Range and Coerce(upper limit=1.0, x=w13, lower limit=0.0) -> (coerced(x)=w10:dbl)  [unwired: 1 out]
    n12 = Multiply(x="Total time", y=w10) -> (x*y=w22:dbl)
    n13 = Bundle("AO SampClk.MaxRate"="AO SampClk.MaxRate", "AI SampClk.MaxRate"="AI SampClk.MaxRate", "AO rate"="AO rate", "Scan speed"="Scan speed", "Detector number"="Detector number", "X min (V)"="X min (V)", "X max (V)"="X max (V)", "X min index"="X min index", "X max index"="X max index", "AO multiline"="AO multiline", "Decimating factor"="Decimating factor", "AvailSampPerChan"="AvailSampPerChan", "AO scan line"="AO scan line", "Total pixels recorded"="Total pixels recorded", "Total lines scanned"="Total lines scanned", "Scan time (m)"="Scan time (m)", "Scan time (s)"="Scan time (s)", "Remaining time (m)"="Remaining time (m)", "Remaining time (s)"="Remaining time (s)", "SEM Spec. I (nA)"="SEM Spec. I (nA)", "Frame"="Frame", w7, w6) -> (w14:T13)  [unwired: 1 out]
    "Info & Status" <- w14
    n14 = Quotient & Remainder(x=w22, y=60.0) -> (x-y*floor(x/y)=w25:dbl, floor(x/y)=w24:dbl)
    n15 = To Variant(anything=w14) -> (Variant=w15:variant)
    n16 = Wait Until Next ms Multiple(millisecond multiple=u32 100) -> ()  [unwired: 1 out]
    n17 = To Unsigned Byte Integer(number=w25) -> (unsigned 8bit integer=w18:u8)
    n18 = To Unsigned Word Integer(number=w24) -> (unsigned 16bit integer=w19:u16)
    n19 = shared-variable ".\\Zeiss Library.lvlib\\SEMInfo"(w15) -> ()  [unwired: 2 out]
    n20 = local write "Remaining time (s)"(w18) -> ()
    n21 = local write "Remaining time (m)"(w19) -> ()
  }
  n22 = stacked-sequence {
    tunnel: w1 -> [_ _ _ _ _]
    frame #0 {
      w137 = i16[][] [] ("SEM")
      n23 = shared-variable ".\\Zeiss Library.lvlib\\SW date"() -> (→"SW date":string)  [unwired: 1 in, 1 out]
      n24 = local write "Det B Img"(w137) -> ()
      n25 = local write "Det A Img"(w137) -> ()
      n26 = Unbundle By Name("HW Config") -> ("Det min (V)"=→"Det min (V)":dbl, "Det max (V)"=→"Det max (V)":dbl, "Eanable COM"=→"Eanable COM":bool, "COM port"=→"COM port":refnum<visa-resource-name>, "Detector FIB-NI auto switch"=→"Detector FIB-NI auto switch":tag, "Machine ID"=w65:string)  [unwired: 1 out]
      "Machine ID" <- w65
      n27 = Unbundle By Name("Scan Para") -> ("X resolution"=w51:u32, "Y resolution"=w52:u32, "X size (V)"=w56:dbl, "Scan rate (Hz)"=→"Scan rate (Hz)":u32, "Oversampling"=→"Oversampling":u32, "Frame line rampdown ratio"=→"Frame line rampdown ratio":sgl, "Pixel size (nm)"=w76:sgl, "WD"=→"WD":sgl, "X stig"=→"X stig":sgl, "Y stig"=→"Y stig":sgl, "X aln"=→"X aln":sgl, "Y aln"=→"Y aln":sgl)  [unwired: 3 out]
      "X resolution" <- w51
      "Y resolution" <- w52
      "Pixel size (nm)" <- w76
      n28 = Unbundle By Name("Options") -> ("GetInfo"=→"GetInfo":bool, "Set Det A para"=→"Set Det A para":bool, "Set WD"=→"Set WD":bool, "Set Mag"=→"Set Mag":bool, "Set stig"=→"Set stig":bool, "Set aln"=→"Set aln":bool, "Display"=→"Display":bool, "Save"=→"Save":bool, "8-bit"=→"8-bit":bool, "Detector A"=→"Detector A":bool, "Detector B"=→"Detector B":bool, "Detector C"=→"Detector C":bool, "Detector D"=→"Detector D":bool, "Inverse A"=→"Inverse A":bool, "Inverse B"=→"Inverse B":bool, "Inverse C"=→"Inverse C":bool, "Inverse D"=→"Inverse D":bool, "Inverse PNG"=→"Inverse PNG":bool, "Freeze"=→"Freeze":bool, "PNG only"=→"PNG only":bool, "Upload"=→"Upload":bool, "Delete after upload"=→"Delete after upload":bool)
      n29 = Unbundle By Name("Focus Index Options") -> ("Keep aspect ratio"=→"keep aspect ratio":bool, "X Grids"=→"X Grids":u8, "Y Grids"=→"Y Grids":u8, "Primary X index"=→"Primary X index":u8, "Primary Y index"=→"Primary Y index":u8)
      n30 = Unbundle By Name("File Info") -> ("File path"=→"File path":path, "Notes"=→"Notes":string, "Sample ID"=→"Sample ID":string)
      n31 = Unbundle By Name("Additional Info") -> ("Restart flag"=→"Restart flag":u8, "Stage move flag"=→"Stage move flag":u8)
      n32 = local read "Inverse A"() -> (w147:bool)
      n33 = Multiply(x=w52, y=w51) -> (x*y=→"Total pixels":u32)
      n34 = case shown="False" w147 {
        tunnel: [u32[] [16777222, 65793, 131586, 197379, 263172, 328965, 394758, 460551, 526344, 592137, 657930, 723723, 789516, 855309, 921102, 986895, 1052688, 1118481, 1184274, 1250067, 1315860, 1381653, 1447446, 1513239, 1579032, 1644825, 1710618, 1776411, 1842204, 1907997, 1973790, 2039583, 2105376, 2171169, 2236962, 2302755, 2368548, 2434341, 2500134, 2565927, 2631720, 2697513, 2763306, 2829099, 2894892, 2960685, 3026478, 3092271, 3158064, 3223857, 3289650, 3355443, 3421236, 3487029, 3552822, 3618615, 3684408, 3750201, 3815994, 3881787, 3947580, 4013373, 4079166, 4144959, 4210752, 4276545, 4342338, 4408131, 4473924, 4539717, 4605510, 4671303, 4737096, 4802889, 4868682, 4934475, 5000268, 5066061, 5131854, 5197647, 5263440, 5329233, 5395026, 5460819, 5526612, 5592405, 5658198, 5723991, 5789784, 5855577, 5921370, 5987163, 6052956, 6118749, 6184542, 6250335, 6316128, 6381921, 6447714, 6513507, 6579300, 6645093, 6710886, 6776679, 6842472, 6908265, 6974058, 7039851, 7105644, 7171437, 7237230, 7303023, 7368816, 7434609, 7500402, 7566195, 7631988, 7697781, 7763574, 7829367, 7895160, 7960953, 8026746, 8092539, 8158332, 8224125, 8289918, 8355711, 8421504, 8487297, 8553090, 8618883, 8684676, 8750469, 8816262, 8882055, 8947848, 9013641, 9079434, 9145227, 9211020, 9276813, 9342606, 9408399, 9474192, 9539985, 9605778, 9671571, 9737364, 9803157, 9868950, 9934743, 10000536, 10066329, 10132122, 10197915, 10263708, 10329501, 10395294, 10461087, 10526880, 10592673, 10658466, 10724259, 10790052, 10855845, 10921638, 10987431, 11053224, 11119017, 11184810, 11250603, 11316396, 11382189, 11447982, 11513775, 11579568, 11645361, 11711154, 11776947, 11842740, 11908533, 11974326, 12040119, 12105912, 12171705, 12237498, 12303291, 12369084, 12434877, 12500670, 12566463, 12632256, 12698049, 12763842, 12829635, 12895428, 12961221, 13027014, 13092807, 13158600, 13224393, 13290186, 13355979, 13421772, 13487565, 13553358, 13619151, 13684944, 13750737, 13816530, 13882323, 13948116, 14013909, 14079702, 14145495, 14211288, 14277081, 14342874, 14408667, 14474460, 14540253, 14606046, 14671839, 14737632, 14803425, 14869218, 14935011, 15000804, 15066597, 15132390, 15198183, 15263976, 15329769, 15395562, 15461355, 15527148, 15592941, 15658734, 15724527, 15790320, 15856113, 15921906, 15987699, 16053492, 16119285, 16185078, 16250871, 16316664, 16382457, 16448250, 16514043, 16579836, 16645629, 16711422, 16448250] ("256 gray scale") u32[] [16448250, 16711422, 16645629, 16579836, 16514043, 16448250, 16382457, 16316664, 16250871, 16185078, 16119285, 16053492, 15987699, 15921906, 15856113, 15790320, 15724527, 15658734, 15592941, 15527148, 15461355, 15395562, 15329769, 15263976, 15198183, 15132390, 15066597, 15000804, 14935011, 14869218, 14803425, 14737632, 14671839, 14606046, 14540253, 14474460, 14408667, 14342874, 14277081, 14211288, 14145495, 14079702, 14013909, 13948116, 13882323, 13816530, 13750737, 13684944, 13619151, 13553358, 13487565, 13421772, 13355979, 13290186, 13224393, 13158600, 13092807, 13027014, 12961221, 12895428, 12829635, 12763842, 12698049, 12632256, 12566463, 12500670, 12434877, 12369084, 12303291, 12237498, 12171705, 12105912, 12040119, 11974326, 11908533, 11842740, 11776947, 11711154, 11645361, 11579568, 11513775, 11447982, 11382189, 11316396, 11250603, 11184810, 11119017, 11053224, 10987431, 10921638, 10855845, 10790052, 10724259, 10658466, 10592673, 10526880, 10461087, 10395294, 10329501, 10263708, 10197915, 10132122, 10066329, 10000536, 9934743, 9868950, 9803157, 9737364, 9671571, 9605778, 9539985, 9474192, 9408399, 9342606, 9276813, 9211020, 9145227, 9079434, 9013641, 8947848, 8882055, 8816262, 8750469, 8684676, 8618883, 8553090, 8487297, 8421504, 8355711, 8289918, 8224125, 8158332, 8092539, 8026746, 7960953, 7895160, 7829367, 7763574, 7697781, 7631988, 7566195, 7500402, 7434609, 7368816, 7303023, 7237230, 7171437, 7105644, 7039851, 6974058, 6908265, 6842472, 6776679, 6710886, 6645093, 6579300, 6513507, 6447714, 6381921, 6316128, 6250335, 6184542, 6118749, 6052956, 5987163, 5921370, 5855577, 5789784, 5723991, 5658198, 5592405, 5526612, 5460819, 5395026, 5329233, 5263440, 5197647, 5131854, 5066061, 5000268, 4934475, 4868682, 4802889, 4737096, 4671303, 4605510, 4539717, 4473924, 4408131, 4342338, 4276545, 4210752, 4144959, 4079166, 4013373, 3947580, 3881787, 3815994, 3750201, 3684408, 3618615, 3552822, 3487029, 3421236, 3355443, 3289650, 3223857, 3158064, 3092271, 3026478, 2960685, 2894892, 2829099, 2763306, 2697513, 2631720, 2565927, 2500134, 2434341, 2368548, 2302755, 2236962, 2171169, 2105376, 2039583, 1973790, 1907997, 1842204, 1776411, 1710618, 1644825, 1579032, 1513239, 1447446, 1381653, 1315860, 1250067, 1184274, 1118481, 1052688, 986895, 921102, 855309, 789516, 723723, 657930, 592137, 526344, 460551, 394758, 328965, 263172, 197379, 131586, 65793, 16777222] ("256 gray scale inverse")] -> _
        frame False {
        }
        frame True {
        }
      }
      n35 = local read "Inverse B"() -> (w148:bool)
      n36 = case shown="False" w148 {
        tunnel: [u32[] [16777222, 65793, 131586, 197379, 263172, 328965, 394758, 460551, 526344, 592137, 657930, 723723, 789516, 855309, 921102, 986895, 1052688, 1118481, 1184274, 1250067, 1315860, 1381653, 1447446, 1513239, 1579032, 1644825, 1710618, 1776411, 1842204, 1907997, 1973790, 2039583, 2105376, 2171169, 2236962, 2302755, 2368548, 2434341, 2500134, 2565927, 2631720, 2697513, 2763306, 2829099, 2894892, 2960685, 3026478, 3092271, 3158064, 3223857, 3289650, 3355443, 3421236, 3487029, 3552822, 3618615, 3684408, 3750201, 3815994, 3881787, 3947580, 4013373, 4079166, 4144959, 4210752, 4276545, 4342338, 4408131, 4473924, 4539717, 4605510, 4671303, 4737096, 4802889, 4868682, 4934475, 5000268, 5066061, 5131854, 5197647, 5263440, 5329233, 5395026, 5460819, 5526612, 5592405, 5658198, 5723991, 5789784, 5855577, 5921370, 5987163, 6052956, 6118749, 6184542, 6250335, 6316128, 6381921, 6447714, 6513507, 6579300, 6645093, 6710886, 6776679, 6842472, 6908265, 6974058, 7039851, 7105644, 7171437, 7237230, 7303023, 7368816, 7434609, 7500402, 7566195, 7631988, 7697781, 7763574, 7829367, 7895160, 7960953, 8026746, 8092539, 8158332, 8224125, 8289918, 8355711, 8421504, 8487297, 8553090, 8618883, 8684676, 8750469, 8816262, 8882055, 8947848, 9013641, 9079434, 9145227, 9211020, 9276813, 9342606, 9408399, 9474192, 9539985, 9605778, 9671571, 9737364, 9803157, 9868950, 9934743, 10000536, 10066329, 10132122, 10197915, 10263708, 10329501, 10395294, 10461087, 10526880, 10592673, 10658466, 10724259, 10790052, 10855845, 10921638, 10987431, 11053224, 11119017, 11184810, 11250603, 11316396, 11382189, 11447982, 11513775, 11579568, 11645361, 11711154, 11776947, 11842740, 11908533, 11974326, 12040119, 12105912, 12171705, 12237498, 12303291, 12369084, 12434877, 12500670, 12566463, 12632256, 12698049, 12763842, 12829635, 12895428, 12961221, 13027014, 13092807, 13158600, 13224393, 13290186, 13355979, 13421772, 13487565, 13553358, 13619151, 13684944, 13750737, 13816530, 13882323, 13948116, 14013909, 14079702, 14145495, 14211288, 14277081, 14342874, 14408667, 14474460, 14540253, 14606046, 14671839, 14737632, 14803425, 14869218, 14935011, 15000804, 15066597, 15132390, 15198183, 15263976, 15329769, 15395562, 15461355, 15527148, 15592941, 15658734, 15724527, 15790320, 15856113, 15921906, 15987699, 16053492, 16119285, 16185078, 16250871, 16316664, 16382457, 16448250, 16514043, 16579836, 16645629, 16711422, 16448250] ("256 gray scale") u32[] [16448250, 16711422, 16645629, 16579836, 16514043, 16448250, 16382457, 16316664, 16250871, 16185078, 16119285, 16053492, 15987699, 15921906, 15856113, 15790320, 15724527, 15658734, 15592941, 15527148, 15461355, 15395562, 15329769, 15263976, 15198183, 15132390, 15066597, 15000804, 14935011, 14869218, 14803425, 14737632, 14671839, 14606046, 14540253, 14474460, 14408667, 14342874, 14277081, 14211288, 14145495, 14079702, 14013909, 13948116, 13882323, 13816530, 13750737, 13684944, 13619151, 13553358, 13487565, 13421772, 13355979, 13290186, 13224393, 13158600, 13092807, 13027014, 12961221, 12895428, 12829635, 12763842, 12698049, 12632256, 12566463, 12500670, 12434877, 12369084, 12303291, 12237498, 12171705, 12105912, 12040119, 11974326, 11908533, 11842740, 11776947, 11711154, 11645361, 11579568, 11513775, 11447982, 11382189, 11316396, 11250603, 11184810, 11119017, 11053224, 10987431, 10921638, 10855845, 10790052, 10724259, 10658466, 10592673, 10526880, 10461087, 10395294, 10329501, 10263708, 10197915, 10132122, 10066329, 10000536, 9934743, 9868950, 9803157, 9737364, 9671571, 9605778, 9539985, 9474192, 9408399, 9342606, 9276813, 9211020, 9145227, 9079434, 9013641, 8947848, 8882055, 8816262, 8750469, 8684676, 8618883, 8553090, 8487297, 8421504, 8355711, 8289918, 8224125, 8158332, 8092539, 8026746, 7960953, 7895160, 7829367, 7763574, 7697781, 7631988, 7566195, 7500402, 7434609, 7368816, 7303023, 7237230, 7171437, 7105644, 7039851, 6974058, 6908265, 6842472, 6776679, 6710886, 6645093, 6579300, 6513507, 6447714, 6381921, 6316128, 6250335, 6184542, 6118749, 6052956, 5987163, 5921370, 5855577, 5789784, 5723991, 5658198, 5592405, 5526612, 5460819, 5395026, 5329233, 5263440, 5197647, 5131854, 5066061, 5000268, 4934475, 4868682, 4802889, 4737096, 4671303, 4605510, 4539717, 4473924, 4408131, 4342338, 4276545, 4210752, 4144959, 4079166, 4013373, 3947580, 3881787, 3815994, 3750201, 3684408, 3618615, 3552822, 3487029, 3421236, 3355443, 3289650, 3223857, 3158064, 3092271, 3026478, 2960685, 2894892, 2829099, 2763306, 2697513, 2631720, 2565927, 2500134, 2434341, 2368548, 2302755, 2236962, 2171169, 2105376, 2039583, 1973790, 1907997, 1842204, 1776411, 1710618, 1644825, 1579032, 1513239, 1447446, 1381653, 1315860, 1250067, 1184274, 1118481, 1052688, 986895, 921102, 855309, 789516, 723723, 657930, 592137, 526344, 460551, 394758, 328965, 263172, 197379, 131586, 65793, 16777222] ("256 gray scale inverse")] -> _
        frame False {
        }
        frame True {
        }
      }
      n37 = xnode "Match Regular Expression"("input string"=w65, "regular expression"="Merlin", "ignore case? (F)"=TRUE) -> ("offset past match"=w85:i32)  [unwired: 3 in, 4 out]
      n38 = xnode "Match Regular Expression"("input string"=w65, "regular expression"="Gemini", "ignore case? (F)"=TRUE) -> ("offset past match"=w71:i32)  [unwired: 3 in, 4 out]
      n39 = local read "Inverse C"() -> (w149:bool)
      n40 = Not Equal?(x=w85, y=-1) -> (x != y?=w66:bool)
      n41 = Not Equal?(x=w71, y=-1) -> (x != y?=w68:bool)
      n42 = Or(x=w66, y=w68) -> (x .or. y?=w67:bool)
      n43 = Divide(x=w56, y=20.0) -> (x/y=w79:dbl)
      n44 = case shown="False" w149 {
        tunnel: [u32[] [16777222, 65793, 131586, 197379, 263172, 328965, 394758, 460551, 526344, 592137, 657930, 723723, 789516, 855309, 921102, 986895, 1052688, 1118481, 1184274, 1250067, 1315860, 1381653, 1447446, 1513239, 1579032, 1644825, 1710618, 1776411, 1842204, 1907997, 1973790, 2039583, 2105376, 2171169, 2236962, 2302755, 2368548, 2434341, 2500134, 2565927, 2631720, 2697513, 2763306, 2829099, 2894892, 2960685, 3026478, 3092271, 3158064, 3223857, 3289650, 3355443, 3421236, 3487029, 3552822, 3618615, 3684408, 3750201, 3815994, 3881787, 3947580, 4013373, 4079166, 4144959, 4210752, 4276545, 4342338, 4408131, 4473924, 4539717, 4605510, 4671303, 4737096, 4802889, 4868682, 4934475, 5000268, 5066061, 5131854, 5197647, 5263440, 5329233, 5395026, 5460819, 5526612, 5592405, 5658198, 5723991, 5789784, 5855577, 5921370, 5987163, 6052956, 6118749, 6184542, 6250335, 6316128, 6381921, 6447714, 6513507, 6579300, 6645093, 6710886, 6776679, 6842472, 6908265, 6974058, 7039851, 7105644, 7171437, 7237230, 7303023, 7368816, 7434609, 7500402, 7566195, 7631988, 7697781, 7763574, 7829367, 7895160, 7960953, 8026746, 8092539, 8158332, 8224125, 8289918, 8355711, 8421504, 8487297, 8553090, 8618883, 8684676, 8750469, 8816262, 8882055, 8947848, 9013641, 9079434, 9145227, 9211020, 9276813, 9342606, 9408399, 9474192, 9539985, 9605778, 9671571, 9737364, 9803157, 9868950, 9934743, 10000536, 10066329, 10132122, 10197915, 10263708, 10329501, 10395294, 10461087, 10526880, 10592673, 10658466, 10724259, 10790052, 10855845, 10921638, 10987431, 11053224, 11119017, 11184810, 11250603, 11316396, 11382189, 11447982, 11513775, 11579568, 11645361, 11711154, 11776947, 11842740, 11908533, 11974326, 12040119, 12105912, 12171705, 12237498, 12303291, 12369084, 12434877, 12500670, 12566463, 12632256, 12698049, 12763842, 12829635, 12895428, 12961221, 13027014, 13092807, 13158600, 13224393, 13290186, 13355979, 13421772, 13487565, 13553358, 13619151, 13684944, 13750737, 13816530, 13882323, 13948116, 14013909, 14079702, 14145495, 14211288, 14277081, 14342874, 14408667, 14474460, 14540253, 14606046, 14671839, 14737632, 14803425, 14869218, 14935011, 15000804, 15066597, 15132390, 15198183, 15263976, 15329769, 15395562, 15461355, 15527148, 15592941, 15658734, 15724527, 15790320, 15856113, 15921906, 15987699, 16053492, 16119285, 16185078, 16250871, 16316664, 16382457, 16448250, 16514043, 16579836, 16645629, 16711422, 16448250] ("256 gray scale") u32[] [16448250, 16711422, 16645629, 16579836, 16514043, 16448250, 16382457, 16316664, 16250871, 16185078, 16119285, 16053492, 15987699, 15921906, 15856113, 15790320, 15724527, 15658734, 15592941, 15527148, 15461355, 15395562, 15329769, 15263976, 15198183, 15132390, 15066597, 15000804, 14935011, 14869218, 14803425, 14737632, 14671839, 14606046, 14540253, 14474460, 14408667, 14342874, 14277081, 14211288, 14145495, 14079702, 14013909, 13948116, 13882323, 13816530, 13750737, 13684944, 13619151, 13553358, 13487565, 13421772, 13355979, 13290186, 13224393, 13158600, 13092807, 13027014, 12961221, 12895428, 12829635, 12763842, 12698049, 12632256, 12566463, 12500670, 12434877, 12369084, 12303291, 12237498, 12171705, 12105912, 12040119, 11974326, 11908533, 11842740, 11776947, 11711154, 11645361, 11579568, 11513775, 11447982, 11382189, 11316396, 11250603, 11184810, 11119017, 11053224, 10987431, 10921638, 10855845, 10790052, 10724259, 10658466, 10592673, 10526880, 10461087, 10395294, 10329501, 10263708, 10197915, 10132122, 10066329, 10000536, 9934743, 9868950, 9803157, 9737364, 9671571, 9605778, 9539985, 9474192, 9408399, 9342606, 9276813, 9211020, 9145227, 9079434, 9013641, 8947848, 8882055, 8816262, 8750469, 8684676, 8618883, 8553090, 8487297, 8421504, 8355711, 8289918, 8224125, 8158332, 8092539, 8026746, 7960953, 7895160, 7829367, 7763574, 7697781, 7631988, 7566195, 7500402, 7434609, 7368816, 7303023, 7237230, 7171437, 7105644, 7039851, 6974058, 6908265, 6842472, 6776679, 6710886, 6645093, 6579300, 6513507, 6447714, 6381921, 6316128, 6250335, 6184542, 6118749, 6052956, 5987163, 5921370, 5855577, 5789784, 5723991, 5658198, 5592405, 5526612, 5460819, 5395026, 5329233, 5263440, 5197647, 5131854, 5066061, 5000268, 4934475, 4868682, 4802889, 4737096, 4671303, 4605510, 4539717, 4473924, 4408131, 4342338, 4276545, 4210752, 4144959, 4079166, 4013373, 3947580, 3881787, 3815994, 3750201, 3684408, 3618615, 3552822, 3487029, 3421236, 3355443, 3289650, 3223857, 3158064, 3092271, 3026478, 2960685, 2894892, 2829099, 2763306, 2697513, 2631720, 2565927, 2500134, 2434341, 2368548, 2302755, 2236962, 2171169, 2105376, 2039583, 1973790, 1907997, 1842204, 1776411, 1710618, 1644825, 1579032, 1513239, 1447446, 1381653, 1315860, 1250067, 1184274, 1118481, 1052688, 986895, 921102, 855309, 789516, 723723, 657930, 592137, 526344, 460551, 394758, 328965, 263172, 197379, 131586, 65793, 16777222] ("256 gray scale inverse")] -> _
        frame False {
        }
        frame True {
        }
      }
      n45 = case shown="True" w67 {
        tunnel: [u8 16 ("t") u8 14 ("t")] -> w83
        tunnel: [u8 1 ("t") u8 25 ("t")] -> w82
        frame False {
        }
        frame True {
        }
      }
      "Image bits" <- w83
      "FI scaling" <- w82
      n46 = expression code="x*1024"(w79) -> (w74:dbl)
      n47 = local read "Detector A"() -> (w141:bool)
      n48 = local read "Detector B"() -> (w140:bool)
      n49 = local read "Detector C"() -> (w142:bool)
      n50 = local read "Detector D"() -> (w143:bool)
      n51 = local read "Inverse D"() -> (w150:bool)
      n52 = Unbundle By Name("Det Info") -> ("Brightness A"=→"Brightness A":dbl, "Contrast A"=→"Contrast A":dbl, "Detector B name"=→"Detector B name":string, "Brightness B"=→"Brightness B":dbl, "Contrast B"=→"Contrast B":dbl, "Detector C name"=→"Detector C name":string, "Detector D name"=→"Detector D name":string)
      n53 = Divide(x=w74, y=w51) -> (x/y=w73:dbl)
      n54 = shared-variable ".\\Zeiss Library.lvlib\\X full scale (V)"() -> (w55:sgl)  [unwired: 1 in, 1 out]
      n55 = Boolean To (0,1)(Boolean=w141) -> (0, 1=w138:i16)
      n56 = Boolean To (0,1)(Boolean=w140) -> (0, 1=w139:i16)
      n57 = Boolean To (0,1)(Boolean=w142) -> (0, 1=w144:i16)
      n58 = Boolean To (0,1)(Boolean=w143) -> (0, 1=w145:i16)
      n59 = case shown="False" w150 {
        tunnel: [u32[] [16777222, 65793, 131586, 197379, 263172, 328965, 394758, 460551, 526344, 592137, 657930, 723723, 789516, 855309, 921102, 986895, 1052688, 1118481, 1184274, 1250067, 1315860, 1381653, 1447446, 1513239, 1579032, 1644825, 1710618, 1776411, 1842204, 1907997, 1973790, 2039583, 2105376, 2171169, 2236962, 2302755, 2368548, 2434341, 2500134, 2565927, 2631720, 2697513, 2763306, 2829099, 2894892, 2960685, 3026478, 3092271, 3158064, 3223857, 3289650, 3355443, 3421236, 3487029, 3552822, 3618615, 3684408, 3750201, 3815994, 3881787, 3947580, 4013373, 4079166, 4144959, 4210752, 4276545, 4342338, 4408131, 4473924, 4539717, 4605510, 4671303, 4737096, 4802889, 4868682, 4934475, 5000268, 5066061, 5131854, 5197647, 5263440, 5329233, 5395026, 5460819, 5526612, 5592405, 5658198, 5723991, 5789784, 5855577, 5921370, 5987163, 6052956, 6118749, 6184542, 6250335, 6316128, 6381921, 6447714, 6513507, 6579300, 6645093, 6710886, 6776679, 6842472, 6908265, 6974058, 7039851, 7105644, 7171437, 7237230, 7303023, 7368816, 7434609, 7500402, 7566195, 7631988, 7697781, 7763574, 7829367, 7895160, 7960953, 8026746, 8092539, 8158332, 8224125, 8289918, 8355711, 8421504, 8487297, 8553090, 8618883, 8684676, 8750469, 8816262, 8882055, 8947848, 9013641, 9079434, 9145227, 9211020, 9276813, 9342606, 9408399, 9474192, 9539985, 9605778, 9671571, 9737364, 9803157, 9868950, 9934743, 10000536, 10066329, 10132122, 10197915, 10263708, 10329501, 10395294, 10461087, 10526880, 10592673, 10658466, 10724259, 10790052, 10855845, 10921638, 10987431, 11053224, 11119017, 11184810, 11250603, 11316396, 11382189, 11447982, 11513775, 11579568, 11645361, 11711154, 11776947, 11842740, 11908533, 11974326, 12040119, 12105912, 12171705, 12237498, 12303291, 12369084, 12434877, 12500670, 12566463, 12632256, 12698049, 12763842, 12829635, 12895428, 12961221, 13027014, 13092807, 13158600, 13224393, 13290186, 13355979, 13421772, 13487565, 13553358, 13619151, 13684944, 13750737, 13816530, 13882323, 13948116, 14013909, 14079702, 14145495, 14211288, 14277081, 14342874, 14408667, 14474460, 14540253, 14606046, 14671839, 14737632, 14803425, 14869218, 14935011, 15000804, 15066597, 15132390, 15198183, 15263976, 15329769, 15395562, 15461355, 15527148, 15592941, 15658734, 15724527, 15790320, 15856113, 15921906, 15987699, 16053492, 16119285, 16185078, 16250871, 16316664, 16382457, 16448250, 16514043, 16579836, 16645629, 16711422, 16448250] ("256 gray scale") u32[] [16448250, 16711422, 16645629, 16579836, 16514043, 16448250, 16382457, 16316664, 16250871, 16185078, 16119285, 16053492, 15987699, 15921906, 15856113, 15790320, 15724527, 15658734, 15592941, 15527148, 15461355, 15395562, 15329769, 15263976, 15198183, 15132390, 15066597, 15000804, 14935011, 14869218, 14803425, 14737632, 14671839, 14606046, 14540253, 14474460, 14408667, 14342874, 14277081, 14211288, 14145495, 14079702, 14013909, 13948116, 13882323, 13816530, 13750737, 13684944, 13619151, 13553358, 13487565, 13421772, 13355979, 13290186, 13224393, 13158600, 13092807, 13027014, 12961221, 12895428, 12829635, 12763842, 12698049, 12632256, 12566463, 12500670, 12434877, 12369084, 12303291, 12237498, 12171705, 12105912, 12040119, 11974326, 11908533, 11842740, 11776947, 11711154, 11645361, 11579568, 11513775, 11447982, 11382189, 11316396, 11250603, 11184810, 11119017, 11053224, 10987431, 10921638, 10855845, 10790052, 10724259, 10658466, 10592673, 10526880, 10461087, 10395294, 10329501, 10263708, 10197915, 10132122, 10066329, 10000536, 9934743, 9868950, 9803157, 9737364, 9671571, 9605778, 9539985, 9474192, 9408399, 9342606, 9276813, 9211020, 9145227, 9079434, 9013641, 8947848, 8882055, 8816262, 8750469, 8684676, 8618883, 8553090, 8487297, 8421504, 8355711, 8289918, 8224125, 8158332, 8092539, 8026746, 7960953, 7895160, 7829367, 7763574, 7697781, 7631988, 7566195, 7500402, 7434609, 7368816, 7303023, 7237230, 7171437, 7105644, 7039851, 6974058, 6908265, 6842472, 6776679, 6710886, 6645093, 6579300, 6513507, 6447714, 6381921, 6316128, 6250335, 6184542, 6118749, 6052956, 5987163, 5921370, 5855577, 5789784, 5723991, 5658198, 5592405, 5526612, 5460819, 5395026, 5329233, 5263440, 5197647, 5131854, 5066061, 5000268, 4934475, 4868682, 4802889, 4737096, 4671303, 4605510, 4539717, 4473924, 4408131, 4342338, 4276545, 4210752, 4144959, 4079166, 4013373, 3947580, 3881787, 3815994, 3750201, 3684408, 3618615, 3552822, 3487029, 3421236, 3355443, 3289650, 3223857, 3158064, 3092271, 3026478, 2960685, 2894892, 2829099, 2763306, 2697513, 2631720, 2565927, 2500134, 2434341, 2368548, 2302755, 2236962, 2171169, 2105376, 2039583, 1973790, 1907997, 1842204, 1776411, 1710618, 1644825, 1579032, 1513239, 1447446, 1381653, 1315860, 1250067, 1184274, 1118481, 1052688, 986895, 921102, 855309, 789516, 723723, 657930, 592137, 526344, 460551, 394758, 328965, 263172, 197379, 131586, 65793, 16777222] ("256 gray scale inverse")] -> _
        frame False {
        }
        frame True {
        }
      }
      n60 = Compound Arithmetic op=ADD(w138, w139, w144, w145) -> (w146:i16)
      n61 = local write "Detector number"(w146) -> ()
      n62 = Divide(x=w56, y=w55) -> (x/y=w57:dbl)
      n63 = expression code="x*1024"(w57) -> (w54:dbl)
      n64 = Divide(x=w54, y=w51) -> (x/y=→"Screen pixel factor":dbl)
      n65 = Divide(x=111652.0, y=w76) -> (x/y=w77:dbl)
      n66 = Multiply(x=w73, y=w77) -> (x*y=→"Mag":dbl)
    }
    frame #1 {
      w411 = T17 3 items=["no dialog", "OK message", "continue or stop message", "OK message + warnings", "continue/stop + warnings"] ("type of dialog (OK msg:1)")
      w415 = 0 items=["one channel for each line", "one channel for all lines"] ("line grouping")
      n67 = shared-variable "My Computer\\Zeiss Library.lvlib\\Machine Type"() -> (w385:u8)  [unwired: 1 in, 1 out]
      n68 = local read "8-bit"() -> (w388:bool)
      n69 = local read "Image bits"() -> (w389:u8)
      n70 = Select(t=u8 8, s=w388, f=w389) -> (s? t:f=w386:u8)
      n71 = local write "Image bits"(w386) -> ()
      n72 = case shown="2" w385 {
        tunnel: [w419 w688] -> w403
        frame 0, Default {
          n73 = local read "Eanable COM"() -> (w420:bool)
          n74 = case shown="True" w420 {
            tunnel: [w421 w452] -> w419
            frame False {
              n75 = local read "Detector B name"() -> (w434:string)
              n76 = local read "Brightness A"() -> (w432:dbl)
              n77 = local read "Contrast A"() -> (w431:dbl)
              n78 = local read "Brightness B"() -> (w430:dbl)
              n79 = local read "Contrast B"() -> (w429:dbl)
              n80 = local read "Mag"() -> (w426:dbl)
              n81 = local read "Pixel size (nm)"() -> (w428:sgl)
              n82 = local read "WD"() -> (w427:sgl)
              n83 = local read "X stig"() -> (w425:sgl)
              n84 = local read "Y stig"() -> (w424:sgl)
              n85 = local read "X aln"() -> (w423:sgl)
              n86 = local read "Y aln"() -> (w422:sgl)
              n87 = local read "SEM parameters"() -> (w435:T5)
              n88 = Bundle By Name(cluster=w435, "Detector A"="Det A", "Detector B"=w434, "Brightness A"=w432, "Contrast A"=w431, "Brightness B"=w430, "Contrast B"=w429, "Magnification"=w426, "Pixel size"=w428, "Working distance"=w427, "Stig X"=w425, "Stig Y"=w424, "Alignment X"=w423, "Alignment Y"=w422) -> (w421:T5)
              n89 = local write "SEM parameters"(w421) -> ()
            }
            frame True {
              n90 = local read "COM port"() -> (w479:refnum<visa-resource-name>)
              n91 = local read "HW Config"() -> (w445:T12)
              n92 = call "Remcon32 command.vi"("Initialization"=TRUE, "SEM command"="frez" ("write buffer"), "COM port in"=w479) -> ("error out"=w459:errorcluster, "COM port out"=w460:refnum<visa-resource-name>)  [unwired: 2 in, 5 out]
              n93 = Unbundle By Name(w445) -> ("Machine ID"=w441:string)
              n94 = local read "Set WD"() -> (w469:bool)
              n95 = call "Remcon32 command.vi"("error in"=w459, "SEM command"="edx 1" ("write buffer"), "COM port in"=w460) -> ("error out"=w447:errorcluster, "COM port out"=w449:refnum<visa-resource-name>)  [unwired: 2 in, 5 out]
              n96 = xnode "Match Regular Expression"("input string"=w441, "regular expression"="Merlin", "ignore case? (F)"=TRUE) -> ("offset past match"=w443:i32)  [unwired: 3 in, 4 out]
              n97 = Equal?(x=w443, y=-1) -> (x = y?=w439:bool)
              n98 = Select(t=u8 1, s=w439, f=u8 7 ("t")) -> (s? t:f=w436:u8)
              n99 = Format Into String(format string="rate %d", w436) -> (resulting string=w451:string)  [unwired: 2 in, 1 out]
              n100 = call "Remcon32 command.vi"("error in"=w447, "SEM command"=w451, "COM port in"=w449) -> ("error out"=w446:errorcluster, "COM port out"=w448:refnum<visa-resource-name>)  [unwired: 2 in, 5 out]
              n101 = local read "Set Mag"() -> (w468:bool)
              n102 = local read "Set Det A para"() -> (w470:bool)
              n103 = call "FIB mode.vi"("error in"=w446, "Iterations"=u32 1, "FIB mode"=T14."SEM", "COM port in"=w448) -> ("error out"=w471:errorcluster, "COM port out"=w472:refnum<visa-resource-name>)  [unwired: 2 in, 4 out]
              n104 = case shown="True" w470 {
                tunnel: w472 -> [w642 w646]
                tunnel: w471 -> [w641 w645]
                tunnel: [w642 w654] -> w466
                tunnel: [w641 w653] -> w465
                frame False {
                }
                frame True {
                  n105 = local read "Brightness A"() -> (w643:dbl)
                  n106 = Format Into String(format string="brgt %g", w643) -> (resulting string=w649:string)  [unwired: 2 in, 1 out]
                  n107 = call "Remcon32 command.vi"("error in"=w645, "SEM command"=w649, "COM port in"=w646) -> ("error out"=w647:errorcluster, "COM port out"=w648:refnum<visa-resource-name>)  [unwired: 2 in, 5 out]
                  n108 = local read "Contrast A"() -> (w644:dbl)
                  n109 = Format Into String(format string="crst %g", w644) -> (resulting string=w651:string)  [unwired: 2 in, 1 out]
                  n110 = call "Remcon32 command.vi"("error in"=w647, "SEM command"=w651, "COM port in"=w648) -> ("error out"=w653:errorcluster, "COM port out"=w654:refnum<visa-resource-name>)  [unwired: 2 in, 5 out]
                }
              }
              n111 = local read "HW Config"() -> (w463:T12)
              n112 = Unbundle By Name(w463) -> ("Machine Type"=w462:u8)
              n113 = local read "GetInfo"() -> (w464:bool)
              n114 = case shown="0, Default" w462 {
                tunnel: [FALSE ("Initialization") TRUE ("Initialization")] -> w461
                frame 0, Default {
                }
                frame 1 {
                }
              }
              n115 = local read "Set stig"() -> (w467:bool)
              n116 = case shown="True" w467 {
                tunnel: [w632 w640] -> w455
                tunnel: [w631 w639] -> w456
                tunnel: w466 -> [w632 w638]
                tunnel: w465 -> [w631 w637]
                frame False {
                }
                frame True {
                  n117 = local read "X stig"() -> (w634:sgl)
                  n118 = local read "Y stig"() -> (w636:sgl)
                  n119 = Format Into String(format string="stim %g %g", w634, w636) -> (resulting string=w633:string)  [unwired: 2 in, 1 out]
                  n120 = call "Remcon32 command.vi"("error in"=w637, "SEM command"=w633, "COM port in"=w638) -> ("error out"=w639:errorcluster, "COM port out"=w640:refnum<visa-resource-name>)  [unwired: 2 in, 5 out]
                }
              }
              n121 = local read "Set aln"() -> (w457:bool)
              n122 = case shown="True" w457 {
                tunnel: [w598 w606] -> w454
                tunnel: [w597 w605] -> w453
                tunnel: w455 -> [w598 w604]
                tunnel: w456 -> [w597 w603]
                frame False {
                }
                frame True {
                  n123 = local read "X aln"() -> (w600:sgl)
                  n124 = local read "Y aln"() -> (w602:sgl)
                  n125 = Format Into String(format string="aaln %g %g", w600, w602) -> (resulting string=w599:string)  [unwired: 2 in, 1 out]
                  n126 = call "Remcon32 command.vi"("error in"=w603, "SEM command"=w599, "COM port in"=w604) -> ("error out"=w605:errorcluster, "COM port out"=w606:refnum<visa-resource-name>)  [unwired: 2 in, 5 out]
                }
              }
              n127 = case shown="True" w469 {
                tunnel: w454 -> [w665 w675]
                tunnel: w453 -> [w664 w674]
                tunnel: [w665 w672] -> w476
                tunnel: [w664 w670] -> w474
                frame False {
                }
                frame True {
                  n128 = local read "WD"() -> (w668:sgl)
                  n129 = call "Remcon32 command.vi"("error in"=w674, "SEM command"="fblk 1", "COM port in"=w675) -> ("error out"=w671:errorcluster, "COM port out"=w673:refnum<visa-resource-name>)  [unwired: 2 in, 5 out]
                  n130 = Format Into String(format string="focs %g", w668) -> (resulting string=w666:string)  [unwired: 2 in, 1 out]
                  n131 = call "Remcon32 command.vi"("error in"=w671, "SEM command"=w666, "COM port in"=w673) -> ("error out"=w670:errorcluster, "COM port out"=w672:refnum<visa-resource-name>)  [unwired: 2 in, 5 out]
                }
              }
              n132 = case shown="True" w468 {
                tunnel: w476 -> [w656 w659]
                tunnel: [w656 w661] -> w475
                tunnel: w474 -> [w655 w658]
                tunnel: [w655 w660] -> w473
                frame False {
                }
                frame True {
                  n133 = local read "Mag"() -> (w657:dbl)
                  n134 = Format Into String(format string="mag %g", w657) -> (resulting string=w662:string)  [unwired: 2 in, 1 out]
                  n135 = call "Remcon32 command.vi"("error in"=w658, "SEM command"=w662, "COM port in"=w659) -> ("error out"=w660:errorcluster, "COM port out"=w661:refnum<visa-resource-name>)  [unwired: 2 in, 5 out]
                }
              }
              n136 = case shown="True" w464 {
                tunnel: [w615 w630] -> w481
                tunnel: [w614 w629] -> w480
                tunnel: w475 -> [w615 w628]
                tunnel: w473 -> [w614 w627]
                tunnel: w461 -> [_ w619]
                tunnel: [w609 w616] -> w452
                frame False {
                  n137 = local read "Mag"() -> (w610:dbl)
                  n138 = local read "Pixel size (nm)"() -> (w611:sgl)
                  n139 = local read "SEM parameters"() -> (w613:T5)
                  n140 = Bundle By Name(cluster=w613, "Magnification"=w610, "Pixel size"=w611) -> (w609:T5)
                  n141 = Wait (ms)(milliseconds to wait=u32 100) -> ()  [unwired: 1 out]
                }
                frame True {
                  w620 = FALSE ("Initialization")
                  n142 = call "Read Zeiss Parameters.vi"("Close session"=w620, "Initialization"=w620, "error in (no error)"=w627, "FIB"=w619, "COM port in"=w628) -> ("error out"=w629:errorcluster, "FIB parameters"=→"FIB parameters":T18, "SEM parameters"=w622:T5, "COM port out"=w630:refnum<visa-resource-name>)  [unwired: 3 out]
                  n143 = local read "Detector B name"() -> (w624:string)
                  n144 = local read "Brightness B"() -> (w625:dbl)
                  n145 = local read "Screen pixel factor"() -> (w618:dbl)
                  n146 = local read "Contrast B"() -> (w626:dbl)
                  n147 = Unbundle By Name(w622) -> ("Pixel size"=w621:sgl)
                  n148 = Multiply(x=w618, y=w621) -> (x*y=w617:dbl)
                  n149 = Bundle By Name(cluster=w622, "Detector B"=w624, "Brightness B"=w625, "Contrast B"=w626, "Pixel size"=w617) -> (w616:T5)
                }
              }
              "SEM parameters" <- w452
              n150 = call "Remcon32 command.vi"("Close session"=TRUE, "error in"=w480, "SEM command"="edx 1" ("write buffer"), "COM port in"=w481) -> ()  [unwired: 1 in, 7 out]
            }
          }
        }
        frame 2 {
          n151 = local read "Options"() -> (w699:T9)
          n152 = local read "Scan Para"() -> (w700:T10)
          n153 = local read "Det Info"() -> (w698:T11)
          n154 = call "SmartSEM Remote API set SEM parameters.vi"("Det Info"=w698, "Scan Para"=w700, "SEM Options"=w699, "ActiveX Container"="ActiveX Container") -> ("error out"=w679:errorcluster, "reference out"=w680:refnum<k7>)  [unwired: 6 in]
          n155 = call "SmartSEM Remote API set string.vi"("error in"=w679, "vValue"="On", "lpszParam"="DP_EXT_SCAN_CONTROL" ("lpszCommand"), "ActiveX Container"=w680) -> ("error out"=w677:errorcluster, "reference out"=w678:refnum<k7>)  [unwired: 6 in]
          n156 = call "SmartSEM Remote API get Zeiss parameters.vi"("error in"=w677, "ActiveX Container"=w678) -> ("error out"=w690:errorcluster, "FIB parameters"=w697:T6, "SEM parameters"=w692:T5, "reference out"=w689:refnum<k7>)  [unwired: 6 in]
          n157 = local read "Detector B name"() -> (w696:string)
          n158 = local read "Screen pixel factor"() -> (w694:dbl)
          n159 = Unbundle By Name(w692) -> ("Pixel size"=w695:sgl)
          n160 = local write "FIB parameters"(w697) -> ()
          n161 = Multiply(x=w694, y=w695) -> (x*y=w693:dbl)
          n162 = Bundle By Name(cluster=w692, "Detector B"=w696, "Pixel size"=w693) -> (w688:T5)
          n163 = local write "SEM parameters"(w688) -> ()
          n164 = invoke class="_EMApi" method="Execute"(reference=w689, error in=w690, "lpszCommand"="CMD_UNFREEZE_ALL") -> (reference out=w687:refnum<k7>, error out=w685:errorcluster)  [unwired: 1 in, 2 out]
          n165 = call "SmartSEM Remote API set string.vi"("Wait (ms)"=u32 10 ("wait (ms)"), "error in"=w685, "vValue"="On", "lpszParam"="DP_EXT_SCAN_CONTROL" ("lpszCommand"), "ActiveX Container"=w687) -> ()  [unwired: 5 in, 2 out]
        }
      }
      n166 = local read "Detector FIB-NI auto switch"() -> (w407:tag)
      n167 = local write "Total lines scanned"(0 ("Read line")) -> ()
      n168 = call-poly <vilib>:"DAQmx Create Virtual Channel.vi"("lines"=w407, "line grouping"=w415) -> ("task out"=w417:refnum<k21>, "error out"=w416:errorcluster)  [unwired: 3 in, 9 out]
      n169 = call <vilib>:"DAQmx Start Task.vi"("task/channels in"=w417, "error in"=w416) -> ("task out"=w414:refnum<k21>, "error out"=w413:errorcluster)  [unwired: 12 out]
      n170 = call-poly <vilib>:"DAQmx Write.vi"("task/channels in"=w414, "data"=TRUE, "error in"=w413) -> ("task out"=w409:refnum<k21>, "error out"=w408:errorcluster)  [unwired: 1 in, 10 out]
      n171 = call <vilib>:"DAQmx Clear Task.vi"("task in"=w409, "error in"=w408) -> ("error out"=w410:errorcluster)  [unwired: 13 out]
      n172 = call <vilib>:"Simple Error Handler.vi"("type of dialog (OK msg:1)"=w411, "error in (no error)"=w410) -> ()  [unwired: 8 out]
      n173 = Unbundle By Name(w403) -> ("Brightness A"=w402:sgl, "Contrast A"=w400:sgl, "Brightness B"=w401:sgl, "Contrast B"=w399:sgl)
      n174 = call "Read detector calibrations.vi"("Contrast B"=w399, "Brightness B"=w401, "Contrast A"=w400, "Brightness A"=w402, "Path"=path "D:/3D FIB-SEM Files/Detector calibrations.csv" ("file path (dialog if empty)")) -> ("Latest 8-bit coefficients"=w390:sgl[][])  [unwired: 6 in]
      "8-bit coefficents" <- w390
      n175 = for {
        tunnel: w390 -> [w701] mode=indexing
        tunnel: [w701] -> w406 mode=concatenating
      }
      n176 = Array To Cluster(array=w406) -> (cluster=w405:T19)
      n177 = Unbundle(w405) -> ("Latest 8-bit coefficients[0]"=→"DetA-Rate":sgl, "Latest 8-bit coefficients[1]"=→"DetA-Io":sgl, "Latest 8-bit coefficients[2]"=→"DetA-k":sgl, "Latest 8-bit coefficients[3]"=→"DetA-Scaling":sgl, "Latest 8-bit coefficients[4]"=→"DetB-Rate":sgl, "Latest 8-bit coefficients[5]"=→"DetB-Io":sgl, "Latest 8-bit coefficients[6]"=→"DetB-k":sgl, "Latest 8-bit coefficients[7]"=→"DetB-Scaling":sgl)
    }
    frame #2 {
      w718 = i16[][] []
      w708 = 0
      w742 = 3 ("index")
      w745 = 1 ("index")
      w805 = 1 ("dimension size")
      # "Watch for SEM Home"
      # "watch for SEM Scan (or early Home)"
      n178 = local read "Save"() -> (w808:bool)
      n179 = local read "HW Config"() -> (w760:T12)
      n180 = local read "Scan Para"() -> (w759:T10)
      n181 = local read "Options"() -> (w758:T9)
      n182 = shared-variable ".\\Zeiss Library.lvlib\\Tclk para"() -> (w762:variant)  [unwired: 1 in, 1 out]
      n183 = Not(x="Force tclk init") -> (.not. x?=w752:bool)
      n184 = local read "Detector A"() -> (w807:bool)
      n185 = local read "Display"() -> (w712:bool)
      n186 = local read "Detector B"() -> (w803:bool)
      n187 = call "Tclk parameters.vi"("variant"=w762, "Options"=w758, "Scan Para"=w759, "HW Config"=w760) -> ("Same tclk para?"=w753:bool)  [unwired: 6 in, 1 out]
      n188 = call "Tclk FGV.vi"("Action"=T15."Get Reference", "Options"=w758, "Scan Para"=w759, "HW Config"=w760) -> ("Tclk handle valid"=w754:bool, "First pixel Y"=w704:i32, "First pixel X"=w705:i32, "Initialized handles"=w757:T20)  [unwired: 4 in]
      n189 = Initialize Array(i16 0 ("element"), w805, w805) -> (w713:i16[][])
      n190 = And(x=w807, y=w712) -> (x .and. y?=w804:bool)
      n191 = And(x=w803, y=w712) -> (x .and. y?=w714:bool)
      n192 = Compound Arithmetic op=AND(w753, w754, w752) -> (w756:bool)
      n193 = case shown="False" w756 {
        tunnel: w760 -> [w842 _]
        tunnel: w759 -> [w841 _]
        tunnel: w758 -> [w840 _]
        tunnel: [w839 w856] -> w766
        tunnel: w757 -> [_ w856]
        tunnel: w705 -> [_ w855]
        tunnel: [w838 w855] -> w703
        tunnel: w704 -> [_ w854]
        tunnel: [w837 w854] -> w702
        frame False {
          n194 = stacked-sequence {
            tunnel: w842 -> [w846 w853]
            tunnel: w841 -> [w845 w852]
            tunnel: w840 -> [w844 w851]
            tunnel: [_ w849] -> w839
            tunnel: [_ w848] -> w838
            tunnel: [_ w847] -> w837
            frame #0 {
              n195 = call "Tclk FGV.vi"("Action"=T15."Close Reference", "Options"=w844, "Scan Para"=w845, "HW Config"=w846) -> ()  [unwired: 4 in, 4 out]
            }
            frame #1 {
              n196 = call "Tclk FGV.vi"("Action"=T15."Initialize Reference", "Options"=w851, "Scan Para"=w852, "HW Config"=w853) -> ("First pixel Y"=w847:i32, "First pixel X"=w848:i32, "Initialized handles"=w849:T20)  [unwired: 4 in, 1 out]
            }
          }
        }
        frame True {
        }
      }
      "First pixel X" <- w703
      "First pixel Y" <- w702
      n197 = Obtain Queue(element data type=i16[] [] ("2D array")) -> (queue out=w825:refnum<queue>, error out=w824:errorcluster)  [unwired: 3 in, 2 out]
      n198 = Unbundle By Name(w766) -> ("sessions out"=w728:refnum<k20>[], "SEM-X handle out"=w790:refnum<k15>, "SEM-Y handle out"=w786:refnum<k15>, "SEM-Y waveform handle out"=w787:i32, "Detectors handle out"=w733:refnum<k15>, "channels"=w784:string, "error out"=w785:errorcluster, "Others.AO SampClk.MaxRate"=w783:dbl, "Others.AI SampClk.MaxRate"=w782:dbl, "Others.AO rate"=w781:dbl, "Others.Scan speed"=w780:u8, "Others.Detector number"=w779:u8, "Others.X min (V)"=w778:dbl, "Others.X max (V)"=w777:dbl, "Others.X min index"=w776:i32, "Others.X max index"=w775:i32, "Others.AO multiline"=w774:u32, "Others.Decimating factor"=w767:u16, "Others.Total time"=w768:dbl, "Others.Scan time (m)"=w773:dbl, "Others.Scan time (s)"=w772:dbl, "Others.Y scan pts per line"=w789:i32, "Others.Y scan pts per AO multiline"=w710:i32, "Others.Small scan"=w709:bool, "Others.Y single line pattern"=w788:dbl[], "Others.Detectors min record length"=w721:u32, "Others.Waveform blocks"=w771:u32, "Others.Repeat count"=w770:u32)
      n199 = Unbundle By Name(w766) -> ("Others.AO rate"=w765:dbl, "Others.Decimating factor"=w764:u16, "Others.X resolution"=w719:u32, "Others.Y resolution"=w711:u32, "Others.X resolution with rampdown"=w722:i32, "Others.Oversampling"=w723:u32, "Others.Detector number"=w763:u8, "Others.AI multiline"=w720:u16)
      "AI multiline" <- w720
      n200 = Quotient & Remainder(x=w711, y=w764) -> (floor(x/y)=w822:u32)  [unwired: 1 out]
      n201 = Quotient & Remainder(x=w719, y=w764) -> (floor(x/y)=w821:u32)  [unwired: 1 out]
      n202 = Initialize Array(i16 0 ("element"), w822, w821) -> (w716:i16[][])
      n203 = case shown="True" w804 {
        tunnel: w716 -> [_ w984]
        tunnel: [w983 w984] -> w717
        tunnel: w713 -> [w983 _]
        frame False {
        }
        frame True {
        }
      }
      n204 = case shown="False" w714 {
        tunnel: w716 -> [_ w834]
        tunnel: [w833 w834] -> w715
        tunnel: w713 -> [w833 _]
        frame False {
        }
        frame True {
        }
      }
      n205 = Multiply(x=w720, y=w719) -> (x*y=w724:u32)
      n206 = Multiply(x=w771, y=w770) -> (x*y=w769:u32)
      n207 = local write "AO SampClk.MaxRate"(w783) -> ()
      n208 = local write "AI SampClk.MaxRate"(w782) -> ()
      n209 = local write "AO rate"(w781) -> ()
      n210 = local write "Scan speed"(w780) -> ()
      n211 = local write "Detector number"(w779) -> ()
      n212 = local write "X min (V)"(w778) -> ()
      n213 = local write "X max (V)"(w777) -> ()
      n214 = local write "X min index"(w776) -> ()
      n215 = local write "X max index"(w775) -> ()
      n216 = local write "AO multiline"(w774) -> ()
      n217 = local write "Decimating factor"(w767) -> ()
      n218 = local write "Total time"(w768) -> ()
      n219 = local write "Scan time (m)"(w773) -> ()
      n220 = local write "Scan time (s)"(w772) -> ()
      n221 = local write "X resolution"(w719) -> ()
      n222 = local write "Y resolution"(w711) -> ()
      n223 = local write "Oversampling"(w723) -> ()
      n224 = local write "Detector number"(w763) -> ()
      n225 = Generate Occurrence() -> (w729:refnum<k4>)
      n226 = flat-sequence {
        tunnel: w729 -> [w836]
        tunnel: [w835] -> w727
        tunnel: w728 -> [w835]
        frame #0 {
          n227 = Wait on Occurrence(2:w836) -> ()  [unwired: 2 in, 1 out]
        }
      }
      n228 = call <instrlib>:"niTClk Initiate.vi"("error in (no error)"=w785, "sessions"=w727) -> ("error out"=w739:errorcluster, "sessions out"=w734:refnum<k20>[])  [unwired: 8 in]
      n229 = To Unsigned Long Integer(number=w720) -> (unsigned 32bit integer=w730:u32)
      n230 = case shown="False" w709 {
        tunnel: w786 -> [w866 w933]
        tunnel: w787 -> [w875 _]
        tunnel: w789 -> [w867 _]
        tunnel: w785 -> [w874 w932]
        tunnel: w774 -> [w861 _]
        tunnel: [w872 w933] -> w795
        tunnel: [w869 w932] -> w793
        tunnel: w788 -> [w862 _]
        tunnel: w710 -> [w865 _]
        tunnel: w769 -> [_ _]
        tunnel: w729 -> [w858 w930]
        frame False {
          n231 = local read "Y resolution"() -> (w871:u32)
          n232 = Delete From Array(array=w862, length=w861, index=0) -> (array with subset deleted=w860:dbl[])  [unwired: 1 out]
          n233 = while {
            tunnel: w861 -> [w884]
            tunnel: w860 -> [w896]
            tunnel: w867 -> [w897]
            shift-right: [w888] -> _
            shift-left: u32 0 -> [w885]
            tunnel: w875 -> [w906]
            tunnel: w874 -> [w904]
            tunnel: [w893] -> w868
            tunnel: [w901] -> w870
            tunnel: w865 -> [w892]
            tunnel: w871 -> [w898]
            shift-right: [w905] -> w873
            shift-left: w866 -> [w890]
            tunnel: dbl[] [] -> [w889]
            tunnel: w858 -> [w887]
            tunnel: [w887] -> w857
            stop <- w907 stop-if-true
            n234 = property class="niFgen"(reference=w890, error in=w904) -> (reference out=w895:refnum<k15>, error out=w891:errorcluster, "Arbitrary Waveform:Data Transfer:Streaming:Space Available in Streaming Waveform"=w902:i32)
            n235 = Equal?(x=w884, y=w885) -> (x = y?=w886:bool)
            n236 = case shown="True" w886 {
              tunnel: w887 -> [_ w908]
              frame False {
              }
              frame True {
                n237 = Set Occurrence(w908) -> ()
              }
            }
            n238 = Wait Until Next ms Multiple(millisecond multiple=u32 1) -> ()  [unwired: 1 out]
            n239 = Less Or Equal?(x=w892, y=w902) -> (x <= y?=w894:bool)
            n240 = case shown="True" w894 {
              tunnel: [w911 w924] -> w905
              tunnel: w895 -> [w911 w923]
              tunnel: [w910 w922] -> w888
              tunnel: w885 -> [w910 w913]
              tunnel: w906 -> [_ w921]
              tunnel: [w909 w920] -> w893
              tunnel: w884 -> [_ w912]
              tunnel: w897 -> [_ w917]
              tunnel: w896 -> [_ w919]
              tunnel: w891 -> [w909 w916]
              tunnel: w889 -> [_ w914]
              frame False {
              }
              frame True {
                n241 = Array Subset(array=w919, index=w913, length=w912) -> (w918:dbl[])
                n242 = Add(x=w912, y=w913) -> (x+y=w922:u32)
                n243 = for {
                  N: w912 -> [_]
                  tunnel: w918 -> [w929] mode=indexing
                  tunnel: w917 -> [w928]
                  shift-right: [w926] -> w915
                  shift-left: w914 -> [w927]
                  n244 = Initialize Array(w929, w928) -> (w925:dbl[])
                  n245 = Build Array (concatenate)(w927, w925) -> (w926:dbl[])
                }
                n246 = call-poly <instrlib>:"niFgen Write Waveform (poly).vi"("Waveform Data"=w915, "error in (no error)"=w916, "Waveform Handle"=w921, "Instrument Handle"=w923) -> ("error out"=w920:errorcluster, "Instrument Handle Out"=w924:refnum<k15>)  [unwired: 5 in, 1 out]
              }
            }
            n247 = local read "stop"() -> (w903:bool)
            n248 = In Range and Coerce(upper limit=w898, x=w888, lower limit=u32 0) -> (coerced(x)=w899:u32)  [unwired: 1 out]
            n249 = local write "AO scan line"(w899) -> ()
            n250 = Less Or Equal?(x=w898, y=w899) -> (x <= y?=w901:bool)
            n251 = Compound Arithmetic op=OR(w901, w893, w903) -> (w907:bool)
          }
          n252 = Set Occurrence(w857) -> ()
          n253 = case shown="True" w870 {
            tunnel: w873 -> [w877 w882]
            tunnel: [w877 w881] -> w872
            tunnel: [w876 w879] -> w869
            tunnel: w868 -> [w876 w878]
            frame False {
            }
            frame True {
              n254 = call <instrlib>:"niFgen Wait Until Done.vi"("error in (no error)"=w878, "MaxTime (msec)"=30000, "Instrument Handle"=w882) -> ("error out"=w879:errorcluster, "Instrument Handle Out"=w881:refnum<k15>)  [unwired: 7 in]
            }
          }
        }
        frame True {
          n255 = Set Occurrence(w930) -> ()
          n256 = local read "Y resolution"() -> (w931:u32)
          n257 = local write "AO scan line"(w931) -> ()
        }
      }
      n258 = Obtain Queue(element data type=i16[][] [] ("wfm")) -> (queue out=w820:refnum<queue>, error out=w725:errorcluster)  [unwired: 3 in, 2 out]
      n259 = while {
        tunnel: w825 -> [w1076]
        tunnel: w824 -> [w1075]
        tunnel: [w1074] -> w813
        tunnel: [w1073] -> w812
        shift-right: [w1072] -> _
        shift-left: 0 -> [w1068]
        tunnel: [w1064] -> w818
        tunnel: [w1071] -> w706
        tunnel: w820 -> [w1070]
        tunnel: [w1069] -> w819
        tunnel: w720 -> [w998]
        tunnel: [w1066] -> w802
        tunnel: w765 -> [w1044]
        tunnel: w764 -> [w1008]
        tunnel: w724 -> [w992]
        tunnel: w723 -> [w995]
        tunnel: w722 -> [w997]
        tunnel: w719 -> [w1037]
        tunnel: w721 -> [w994]
        shift-right: [w1035] -> _
        shift-left: w717 -> [w1036]
        shift-right: [w1012] -> _
        shift-left: w708 -> [w1010]
        shift-right: [w1006] -> _
        shift-left: w718 -> [w1011]
        shift-right: [w1014] -> _
        shift-left: w718 -> [w1013]
        shift-right: [w1005] -> _
        shift-left: w715 -> [w1007]
        shift-right: [w1002] -> _
        shift-left: w708 -> [w1001]
        stop <- w1066 stop-if-true
        w1059 = 1 ("index")
        w1063 = 0 ("index")
        n260 = Dequeue Element(queue=w1070) -> (queue out=w1069:refnum<queue>, element=w1061:i16[][], error out=w1064:errorcluster)  [unwired: 1 in, 2 out]
        n261 = local read "Detector A"() -> (w1056:bool)
        n262 = local read "Detector B"() -> (w1057:bool)
        n263 = Array Subset(array=w1061, index (row)=w1063, length (row)=1 ("length"), index (col)=w1063) -> (w999:i16[][])  [unwired: 1 in]
        n264 = Array Subset(array=w1061, index (row)=w1059, length (row)=w1059, index (col)=0 ("length")) -> (w993:i16[][])  [unwired: 1 in]
        n265 = Reshape Array(w999, w994) -> (w1054:i16[])
        n266 = Build Array(w1056, w1057) -> (w1058:bool[])
        n267 = Reshape Array(w993, w994) -> (w1050:i16[])
        n268 = To Double Precision Float(number=w1054) -> (double precision float=w1000:dbl[])
        n269 = Boolean Array To Number(Boolean array=w1058) -> (number=w991:u32)
        n270 = To Double Precision Float(number=w1050) -> (double precision float=w1051:dbl[])
        n271 = call-poly <vilib>:"Decimate (single shot).vi"("averaging"=TRUE, "decimating factor"=w995, "X"=w1000) -> ("Decimated Array"=w1053:dbl[])  [unwired: 8 out]
        n272 = call-poly <vilib>:"Decimate (single shot).vi"("averaging"=TRUE, "decimating factor"=w995, "X"=w1051) -> ("Decimated Array"=w1049:dbl[])  [unwired: 8 out]
        n273 = local read "8-bit"() -> (w1047:bool)
        n274 = case shown="3" w991 {
          tunnel: w1053 -> [w1182 w1184 w1186]
          tunnel: w1049 -> [_ _ w1185]
          tunnel: [w1182 dbl[] [] ("output array") w1186] -> w1046
          tunnel: [dbl[] [] ("output array") w1184 w1185] -> w1045
          frame 1, Default {
          }
          frame 2 {
          }
          frame 3 {
          }
        }
        n275 = case shown="False" w1047 {
          tunnel: [w1170 w1177] -> w1048
          tunnel: w1046 -> [w1170 w1179]
          tunnel: w1044 -> [_ w1172]
          frame False {
          }
          frame True {
            n276 = local read "DetA-Rate"() -> (w1175:sgl)
            n277 = local read "DetA-Scaling"() -> (w1173:sgl)
            n278 = local read "DetA-Io"() -> (w1180:sgl)
            n279 = local read "DetA-k"() -> (w1176:sgl)
            n280 = Subtract(x=w1179, y=w1180) -> (x-y=w1178:dbl[])
            n281 = Divide(x=w1175, y=w1172) -> (x/y=w1174:dbl)
            n282 = Multiply(x=w1174, y=w1173) -> (x*y=w1171:dbl)
            n283 = Compound Arithmetic op=MULTIPLY(w1178, w1176, w1171) -> (w1177:dbl[])
          }
        }
        n284 = case shown="True" w1047 {
          tunnel: [w1159 w1166] -> w1043
          tunnel: w1045 -> [w1159 w1168]
          tunnel: w1044 -> [_ w1161]
          frame False {
          }
          frame True {
            n285 = local read "DetB-Rate"() -> (w1164:sgl)
            n286 = local read "DetB-Scaling"() -> (w1163:sgl)
            n287 = local read "DetB-Io"() -> (w1169:sgl)
            n288 = local read "DetB-k"() -> (w1165:sgl)
            n289 = Subtract(x=w1168, y=w1169) -> (x-y=w1167:dbl[])
            n290 = Divide(x=w1164, y=w1161) -> (x/y=w1162:dbl)
            n291 = Multiply(x=w1162, y=w1163) -> (x*y=w1160:dbl)
            n292 = Compound Arithmetic op=MULTIPLY(w1167, w1165, w1160) -> (w1166:dbl[])
          }
        }
        n293 = To Word Integer(number=w1048) -> (16bit integer=w1042:i16[])
        n294 = To Word Integer(number=w1043) -> (16bit integer=w1041:i16[])
        n295 = Reshape Array(w1042, w998, w997) -> (w1040:i16[][])
        n296 = Reshape Array(w1041, w998, w997) -> (w1030:i16[][])
        n297 = To Long Integer(number=w1037) -> (32bit integer=w996:i32)
        n298 = Array Subset(array=w1040, index (row)=0 ("index"), index (col)=1 ("index"), length (col)=w996) -> (w1004:i16[][])  [unwired: 1 in]
        n299 = Array Subset(array=w1030, index (row)=0 ("index"), index (col)=1 ("index"), length (col)=w996) -> (w1003:i16[][])  [unwired: 1 in]
        n300 = Reshape Array(w1004, w992) -> (w1027:i16[])
        n301 = Reshape Array(w1003, w992) -> (w1026:i16[])
        n302 = local read "Detector A"() -> (w1034:bool)
        n303 = local read "Display"() -> (w1028:bool)
        n304 = local read "Detector B"() -> (w1029:bool)
        n305 = case shown="3" w991 {
          tunnel: w1027 -> [w1119 _ w1123]
          tunnel: w1026 -> [_ w1120 w1122]
          tunnel: [w1119 w1120 w1121] -> w1015
          frame 1, Default {
          }
          frame 2 {
          }
          frame 3 {
            n306 = Interleave 1D Arrays(w1123, w1122) -> (w1121:i16[])
          }
        }
        n307 = local read "Save"() -> (w1018:bool)
        n308 = And(x=w1034, y=w1028) -> (x .and. y?=w1033:bool)
        n309 = And(x=w1028, y=w1029) -> (x .and. y?=w1009:bool)
        n310 = local read "Detector number"() -> (w1023:u8)
        n311 = case shown="True" w1033 {
          tunnel: w1004 -> [_ w1129]
          tunnel: w1036 -> [w1126 w1139]
          tunnel: w1008 -> [_ w1133]
          tunnel: [w1126 w1138] -> w1035
          tunnel: [w1125 w1137] -> w1014
          tunnel: w1013 -> [w1125 w1128]
          tunnel: w1010 -> [w1124 w1131]
          tunnel: [w1124 w1130] -> w1012
          frame False {
          }
          frame True {
            n312 = Build Array (concatenate)(w1128, w1129) -> (w1127:i16[][])
            n313 = Array Size(array=w1127) -> (size(s)=w1136:i32[])
            n314 = Index Array(array=w1136, index=0) -> (element=w1132:i32)
            n315 = Greater Or Equal?(x=w1132, y=w1133) -> (x >= y?=w1134:bool)
            n316 = case shown="True" w1134 {
              tunnel: w1139 -> [w1142 w1158]
              tunnel: w1133 -> [_ w1154]
              tunnel: [w1142 w1155] -> w1138
              tunnel: [w1140 w1143] -> w1137
              tunnel: w1132 -> [_ w1151]
              tunnel: w1131 -> [w1141 w1146]
              tunnel: [w1141 w1149] -> w1130
              tunnel: w1127 -> [w1140 w1144]
              frame False {
              }
              frame True {
                n317 = Quotient & Remainder(x=w1151, y=w1154) -> (x-y*floor(x/y)=w1152:i32, floor(x/y)=w1147:i32)
                n318 = Subtract(x=w1151, y=w1152) -> (x-y=w1148:i32)
                n319 = Add(x=w1147, y=w1146) -> (x+y=w1149:i32)
                n320 = Delete From Array(array=w1144, length=w1148, index (row)=0) -> (deleted portion=w1150:i16[][], array with subset deleted=w1143:i16[][])  [unwired: 1 in]
                n321 = call "2D Array Decimate.vi"("averaging"=TRUE, "y decimating factor"=w1154, "x decimating factor"=w1154, "Input 2D Array"=w1150) -> ("output array"=w1156:dbl[][])  [unwired: 7 out]
                n322 = Replace Array Subset(array=w1158, new element=w1156, index (row)=w1146, index (col)=0 ("disabled index (col)")) -> (w1155:i16[][])
                "Det A Img" <- w1155
                n323 = shared-variable ".\\Zeiss Library.lvlib\\Det A Img"(w1155) -> ()  [unwired: 1 in, 1 out]
              }
            }
          }
        }
        n324 = case shown="True" w1009 {
          tunnel: w1003 -> [_ w1085]
          tunnel: w1007 -> [w1079 w1092]
          tunnel: w1008 -> [_ w1087]
          tunnel: [w1079 w1091] -> w1005
          tunnel: [w1078 w1090] -> w1006
          tunnel: w1011 -> [w1078 w1084]
          tunnel: w1001 -> [w1077 w1086]
          tunnel: [w1077 w1080] -> w1002
          frame False {
          }
          frame True {
            n325 = Build Array (concatenate)(w1084, w1085) -> (w1083:i16[][])
            n326 = Array Size(array=w1083) -> (size(s)=w1082:i32[])
            n327 = Index Array(array=w1082, index=0) -> (element=w1081:i32)
            n328 = Greater Or Equal?(x=w1081, y=w1087) -> (x >= y?=w1088:bool)
            n329 = case shown="True" w1088 {
              tunnel: w1092 -> [w1095 w1111]
              tunnel: w1087 -> [_ w1108]
              tunnel: [w1095 w1103] -> w1091
              tunnel: [w1094 w1099] -> w1090
              tunnel: w1086 -> [w1093 w1098]
              tunnel: w1083 -> [w1094 w1101]
              tunnel: w1081 -> [_ w1100]
              tunnel: [w1093 w1096] -> w1080
              frame False {
              }
              frame True {
                n330 = Quotient & Remainder(x=w1100, y=w1108) -> (x-y*floor(x/y)=w1106:i32, floor(x/y)=w1097:i32)
                n331 = Subtract(x=w1100, y=w1106) -> (x-y=w1104:i32)
                n332 = Add(x=w1097, y=w1098) -> (x+y=w1096:i32)
                n333 = Delete From Array(array=w1101, length=w1104, index (row)=0) -> (deleted portion=w1105:i16[][], array with subset deleted=w1099:i16[][])  [unwired: 1 in]
                n334 = call "2D Array Decimate.vi"("averaging"=TRUE, "y decimating factor"=w1108, "x decimating factor"=w1108, "Input 2D Array"=w1105) -> ("output array"=w1109:dbl[][])  [unwired: 7 out]
                n335 = Replace Array Subset(array=w1111, new element=w1109, index (row)=w1098, index (col)=0 ("disabled index (col)")) -> (w1103:i16[][])
                "Det B Img" <- w1103
                n336 = shared-variable ".\\Zeiss Library.lvlib\\Det B Img"(w1103) -> ()  [unwired: 1 in, 1 out]
              }
            }
          }
        }
        n337 = Array Size(array=w1015) -> (size(s)=w1024:i32)
        n338 = local read "PNG only"() -> (w1020:bool)
        n339 = Not(x=w1020) -> (.not. x?=w1019:bool)
        n340 = To Long Integer(number=w1023) -> (32bit integer=w1022:i32)
        n341 = And(x=w1018, y=w1019) -> (x .and. y?=w1017:bool)
        n342 = Quotient & Remainder(x=w1024, y=w1022) -> (floor(x/y)=w1025:i32)  [unwired: 1 out]
        n343 = Add(x=w1025, y=w1068) -> (x+y=w1072:i32)
        n344 = case shown="True" w1017 {
          tunnel: w1076 -> [w1113 w1118]
          tunnel: w1075 -> [w1112 w1117]
          tunnel: [w1113 w1116] -> w1074
          tunnel: [w1112 w1115] -> w1073
          tunnel: w1015 -> [_ w1114]
          frame False {
          }
          frame True {
            n345 = Enqueue Element(queue=w1118, element=w1114, error in (no error)=w1117) -> (queue out=w1116:refnum<queue>, error out=w1115:errorcluster)  [unwired: 2 out]
          }
        }
        n346 = local write "Total pixels recorded"(w1072) -> ()
        n347 = local read "Total pixels"() -> (w1016:u32)
        n348 = To Unsigned Long Integer(number=w1072) -> (unsigned 32bit integer=w1021:u32)
        n349 = Greater Or Equal?(x=w1021, y=w1016) -> (x >= y?=w1065:bool)
        n350 = Unbundle By Name(w1064) -> ("status"=w1071:bool)
        n351 = local read "stop"() -> (w1067:bool)
        n352 = Compound Arithmetic op=OR(w1065, w1071, w1067) -> (w1066:bool)
      }
      n353 = while {
        tunnel: w820 -> [w1898]
        tunnel: w725 -> [w1897]
        tunnel: [w1896] -> w832
        tunnel: [w1895] -> w830
        tunnel: w711 -> [w1881]
        tunnel: w785 -> [w1893]
        tunnel: w721 -> [w1892]
        tunnel: [w1890] -> w794
        tunnel: w784 -> [w1891]
        tunnel: [w1885] -> w799
        tunnel: w734 -> [_]
        shift-right: [w1876] -> w750
        shift-left: sgl[][] [] -> [w1877]
        shift-right: [w1887] -> w798
        shift-left: w733 -> [w1879]
        shift-right: [w1873] -> _
        shift-left: u32 0 -> [w1875]
        tunnel: w730 -> [w1874]
        stop <- w1894 stop-if-true
        n354 = call-poly <instrlib>:"niScope Fetch (poly).vi"("error in"=w1893, "numSamples"=w1892, "channels"=w1891, "instrument handle"=w1879) -> ("error out"=w1889:errorcluster, "wfm"=w1872:i16[][], "instrument handle out"=w1888:refnum<k15>)  [unwired: 4 in, 1 out]
        n355 = Add(x=w1875, y=w1874) -> (x+y=w1873:u32)
        n356 = property class="niScope"(reference=w1888, error in=w1889) -> (reference out=w1887:refnum<k15>, error out=w1890:errorcluster, "Fetch Backlog"=w1886:dbl)
        n357 = local write "AvailSampPerChan"(w1886) -> ()
        n358 = In Range and Coerce(upper limit=w1881, x=w1873, lower limit=u32 0) -> (coerced(x)=w1884:u32)  [unwired: 1 out]
        n359 = shared-variable ".\\Zeiss Library.lvlib\\Logs"() -> (w1878:sgl[])  [unwired: 1 in, 1 out]
        n360 = Greater Or Equal?(x=w1873, y=w1881) -> (x >= y?=w1882:bool)
        n361 = local write "Total lines scanned"(w1884) -> ()
        n362 = Build Array (concatenate)(w1877, w1878) -> (w1876:sgl[][])
        n363 = Enqueue Element(queue=w1898, element=w1872, error in (no error)=w1897) -> (queue out=w1896:refnum<queue>, error out=w1895:errorcluster)  [unwired: 2 out]
        n364 = Unbundle By Name(w1890) -> ("status"=w1885:bool)
        n365 = local read "stop"() -> (w1883:bool)
        n366 = Compound Arithmetic op=OR(w1885, w1882, w1883) -> (w1894:bool)
      }
      n367 = call "FM Gen Pulse for FIB-SEM.vi"("WatchDog Mode"="WatchDog Mode", "error in"=w739, "State Value"=i16 4) -> ()  [unwired: 6 in, 3 out]
      n368 = Array Size(array=w750) -> (size(s)=w751:i32[])
      n369 = Index Array(array=w751) -> (element=w744:i32)  [unwired: 1 in]
      n370 = call <instrlib>:"niScope Abort.vi"("instrument handle"=w798, "error in"=w794) -> ("error out"=w737:errorcluster)  [unwired: 12 in, 1 out]
      n371 = Subtract(x=w744, y=w742) -> (x-y=w743:i32)
      n372 = Array Subset(array=w750, index (row)=w742, index (col)=w745, length (col)=w745) -> (w749:sgl[][])  [unwired: 1 in]
      n373 = Reshape Array(w749, w743) -> (w748:sgl[])
      n374 = call-poly <vilib>:"Basic Averaged DC-RMS.vi"("signal in"=w748) -> ("DC value"=w746:dbl)  [unwired: 7 in, 3 out]
      n375 = To Single Precision Float(number=w746) -> (single precision float=w747:sgl)
      n376 = local write "SEM Spec. I (nA)"(w747) -> ()
      n377 = Build Array(w790, w795) -> (w797:refnum<k15>[])
      n378 = Merge Errors(w793, w737) -> (w792:errorcluster)
      n379 = Get Queue Status(queue=w832, error in (no error)=w830) -> (queue out=w831:refnum<queue>, error out=w829:errorcluster, # elements in queue=w828:i32)  [unwired: 6 out]
      n380 = Equal To 0?(x=w828) -> (x = 0?=w827:bool)
      n381 = for {
        tunnel: w797 -> [w936] mode=indexing
        shift-right: [w934] -> w791
        shift-left: w792 -> [w935]
        n382 = call <instrlib>:"niFgen Abort Generation.vi"("error in (no error)"=w935, "Instrument Handle"=w936) -> ("error out"=w934:errorcluster)  [unwired: 8 in, 1 out]
      }
      n383 = Compound Arithmetic op=OR(w827, w799) -> (w826:bool)
      n384 = case shown="True" w826 {
        tunnel: w831 -> [_ w1871]
        tunnel: w829 -> [w1868 w1870]
        tunnel: [w1868 w1869] -> w796
        frame False {
        }
        frame True {
          n385 = Release Queue(queue=w1871, error in (no error)=w1870) -> (error out=w1869:errorcluster)  [unwired: 3 out]
        }
      }
      n386 = Generate Occurrence() -> (w801:refnum<k4>)
      n387 = case shown="True" w808 {
        tunnel: w825 -> [_ w1192]
        tunnel: [_ w1191] -> w811
        tunnel: [_ w1190] -> w810
        tunnel: w801 -> [_ w1189]
        tunnel: w733 -> [_ w1188]
        tunnel: w765 -> [_ w1187]
        frame False {
        }
        frame True {
          n388 = stacked-sequence {
            tunnel: w1192 -> [_ _ w1342 _ _]
            tunnel: [_ _ w1341 _ _] -> w1191
            tunnel: [_ _ w1340 _ _] -> w1190
            tunnel: w1189 -> [_ _ w1338 _ _]
            tunnel: w1188 -> [_ _ w1337 _ _]
            tunnel: w1187 -> [_ _ w1336 w1663 _]
            frame #0 {
              w1194 = "-" ("string")
              w1203 = "_" ("string")
              n389 = local read "Machine ID"() -> (w1208:string)
              n390 = local read "Tile index"() -> (w1196:u8[])
              n391 = local read "Frame"() -> (w1193:u8)
              n392 = Format Into String(w1193) -> (resulting string=w1195:string)  [unwired: 3 in, 1 out]
              n393 = Index Array(array=w1196) -> (element #1=w1198:u8, element #2=w1197:u8)  [unwired: 2 in]
              n394 = Compound Arithmetic op=ADD(w1197, w1198, w1193) -> (w1199:u8)
              n395 = Equal To 0?(x=w1199) -> (x = 0?=w1200:bool)
              n396 = case shown="False" w1200 {
                tunnel: [w1220 w1221] -> w1206
                frame False {
                  n397 = local read "Timestamp"() -> (w1220:timestamp)
                }
                frame True {
                  n398 = Get Date/Time In Seconds() -> (seconds since 1Jan1904=w1221:timestamp)
                }
              }
              "Timestamp" <- w1206
              n399 = local read "File path"() -> (w1211:path)
              n400 = xnode "Match Regular Expression"("input string"=w1208, "regular expression"="/") -> ("after match"=w1209:string)  [unwired: 4 in, 4 out]
              n401 = Format Date/Time String(time format string (%c)="%y-%m-%d_%H%M%S", seconds (now)=w1206) -> (date/time string=w1214:string)  [unwired: 1 out]
              n402 = Format Into String(w1198) -> (resulting string=w1202:string)  [unwired: 3 in, 1 out]
              n403 = Format Into String(w1197) -> (resulting string=w1201:string)  [unwired: 3 in, 1 out]
              n404 = Format Date/Time String(time format string (%c)="Y%Y\\M%m\\D%d", seconds (now)=w1206) -> (date/time string=w1207:string)  [unwired: 1 out]
              n405 = Build Path(base path=w1211, name or relative path=w1207) -> (appended path=w1212:path)
              n406 = Concatenate Strings(w1209, w1203, w1214, w1203, w1195, w1194, w1202, w1194, w1201, ".dat" ("string")) -> (w1205:string)
              n407 = File/Directory Info(path=w1212) -> (path out=w1219:path, error out=w1217:errorcluster)  [unwired: 1 in, 5 out]
              n408 = Build Path(base path=w1212, name or relative path=w1205) -> (appended path=→"File name":path)
              n409 = Unbundle By Name(w1217) -> ("status"=w1218:bool)
              n410 = case shown="True" w1218 {
                tunnel: w1219 -> [_ w1333]
                frame False {
                }
                frame True {
                  n411 = Create Folder(path (use dialog)=w1333) -> ()  [unwired: 1 in, 4 out]
                }
              }
            }
            frame #1 {
              n412 = local read "PNG only"() -> (w1334:bool)
              n413 = case shown="False" w1334 {
                frame False {
                  "Runsheet header array" <- string[] ["Date", "Time", "Notes", "Detector A", "Detector B", "Detector C", "Detector D", "Detectors", "X resolution", "Y resolution", "Rate (Hz)", "Brightness A (%)", "Contrast A (%)", "Brightness B (%)", "Contrast B (%)", "Magnification", "Pixel size (nm)", "Working Distance (mm)", "EHT (kV)", "Aperture #", "High Current Mode", "Probe Current (A)", "Beam Shift X", "Beam Shift Y", "Stigmation X", "Stigmation Y", "Alignment X", "Alignment Y", "FIB spacing (nm)", "A Img Focus Index", "B Img Focus Index", "A Img FRC resolution (nm)", "B Img FRC resolution (nm)", "A Img Primary Grid Mean", "A Img Primary Grid Std", "B Img Primary Grid Mean", "B Img Primary Grid Std", "Temp (F)", "FIB Faraday Cup (nA)", "Specimen I (nA)", "Milling Beam Dump 1 (nA)", "Milling Beam Dump 2 (nA)", "Milling I (nA)", "SEM Specimen I (nA)", "Milling Z voltage (V)", "Image Delta X (nm)", "Image Delta Y (nm)", "Image Delta Z"]
                }
                frame True {
                }
              }
            }
            frame #2 {
              n414 = local read "PNG only"() -> (w1339:bool)
              n415 = case shown="False" w1339 {
                tunnel: w1342 -> [w1502 _]
                tunnel: [w1501 _] -> w1341
                tunnel: [w1500 _] -> w1340
                tunnel: w1338 -> [_ w1662]
                tunnel: w1337 -> [w1440 _]
                tunnel: w1336 -> [w1392 _]
                frame False {
                  w1343 = 0.0 ("element")
                  w1357 = u32 0 ("Y line out")
                  w1375 = 1 ("dimension size")
                  w1470 = u8 1 ("lower limit")
                  w1514 = "\"" ("string")
                  w1535 = T17 3 items=["no dialog", "OK message", "continue or stop message", "OK message + warnings", "continue/stop + warnings"] ("type of dialog (OK msg:1)")
                  n416 = property class="niScope"(reference=w1440) -> ("Actual Sample Rate"=w1444:dbl)  [unwired: 1 in, 2 out]
                  n417 = local read "8-bit"() -> (w1409:bool)
                  n418 = local read "8-bit coefficents"() -> (w1398:sgl[][])
                  n419 = local read "Restart flag"() -> (w1348:u8)
                  n420 = local read "Stage move flag"() -> (w1347:u8)
                  n421 = local read "First pixel X"() -> (w1346:i32)
                  n422 = local read "First pixel Y"() -> (w1345:i32)
                  n423 = local read "Detector A"() -> (w1526:bool)
                  n424 = local read "Detector B"() -> (w1525:bool)
                  n425 = local read "Detector C"() -> (w1507:bool)
                  n426 = local read "Detector D"() -> (w1506:bool)
                  n427 = local read "X resolution"() -> (w1521:u32)
                  n428 = local read "Y resolution"() -> (w1532:u32)
                  n429 = local read "Oversampling"() -> (w1533:u32)
                  n430 = local read "Scan speed"() -> (w1527:u8)
                  n431 = local read "Frame line rampdown ratio"() -> (w1534:sgl)
                  n432 = local read "X min (V)"() -> (w1474:dbl)
                  n433 = local read "X max (V)"() -> (w1508:dbl)
                  n434 = local read "Det min (V)"() -> (w1476:dbl)
                  n435 = local read "Det max (V)"() -> (w1475:dbl)
                  n436 = local read "Decimating factor"() -> (w1419:u16)
                  n437 = local read "Sample ID"() -> (w1349:string)
                  n438 = local read "Notes"() -> (w1449:string)
                  n439 = local read "Detector C name"() -> (w1503:string)
                  n440 = local read "Detector D name"() -> (w1504:string)
                  n441 = local read "SEM parameters"() -> (w1445:T5)
                  n442 = local read "FIB parameters"() -> (w1447:T6)
                  n443 = local read "Machine ID"() -> (w1446:string)
                  n444 = call-poly <instrlib>:"niScope Get Wfm Coefficients (poly).vi"("instrument handle"=w1440, "channels"="0,1") -> ("coefficient info"=w1442:T21)  [unwired: 11 in, 2 out]
                  n445 = To Single Precision Float(number=w1442) -> (single precision float=w1441:T22)
                  n446 = Bundle("Detector A"=w1526, "Detector B"=w1525, "Detector C"=w1507, "Detector D"=w1506) -> (w1451:T23)  [unwired: 1 out]
                  n447 = Reciprocal(x=w1444) -> (1/x=w1439:dbl)
                  n448 = Bundle("Detector C name"=w1503, "Detector D name"=w1504) -> (w1448:T24)  [unwired: 1 out]
                  n449 = for {
                    tunnel: w1441 -> [w1557] mode=indexing
                    tunnel: [w1556] -> w1411 mode=indexing
                    n450 = Unbundle By Name(w1557) -> ("offset"=w1561:sgl, "gain"=w1560:sgl, "reserved 1"=w1559:sgl, "reserved 2"=w1558:sgl)
                    n451 = Build Array(w1561, w1560, w1559, w1558) -> (w1556:sgl[])
                  }
                  n452 = Bundle("X resolution"=w1521, "Y resolution"=w1532, "Oversampling"=w1533, "Scan speed"=w1527, "AO rate"=w1392, "Frame line rampdown ratio"=w1534, "X min (V)"=w1474, "X max (V)"=w1508, "Det min (V)"=w1476, "Det max (V)"=w1475) -> (w1450:T25)  [unwired: 1 out]
                  n453 = local read "Detector number"() -> (w1517:u8)
                  n454 = Unbundle By Name(w1450) -> ("X resolution"=w1518:u32, "Y resolution"=w1519:u32, "AO rate"=w1520:dbl)
                  n455 = Unbundle By Name(w1445) -> ("Detector A"=w1512:string, "Detector B"=w1511:string, "Brightness A"=w1499:sgl, "Contrast A"=w1498:sgl, "Brightness B"=w1509:sgl, "Contrast B"=w1510:sgl, "Magnification"=w1497:sgl, "Pixel size"=w1496:sgl, "Working distance"=w1495:sgl, "EHT"=w1494:sgl, "Aperture"=w1493:u8, "High current mode"=w1492:u8, "Probe current"=w1491:sgl, "Beam shift X"=w1486:sgl, "Beam shift Y"=w1485:sgl, "Stig X"=w1490:sgl, "Stig Y"=w1489:sgl, "Alignment X"=w1488:sgl, "Alignment Y"=w1487:sgl)
                  n456 = Unbundle By Name("Milling para") -> ("Z-step (nm)"=w1378:dbl)
                  n457 = Select(t=w1398, s=TRUE, f=w1411) -> (s? t:f=w1410:sgl[][])
                  n458 = shared-variable ".\\Zeiss Library.lvlib\\Temp (F)"() -> (w1428:sgl)  [unwired: 1 in, 1 out]
                  n459 = shared-variable ".\\Zeiss Library.lvlib\\Faraday Cup (nA)"() -> (w1427:sgl)  [unwired: 1 in, 1 out]
                  n460 = shared-variable ".\\Zeiss Library.lvlib\\Specimen (nA)"() -> (w1426:sgl)  [unwired: 1 in, 1 out]
                  n461 = shared-variable ".\\Zeiss Library.lvlib\\Beam Dump 1 (nA)"() -> (w1425:sgl)  [unwired: 1 in, 1 out]
                  n462 = shared-variable ".\\Zeiss Library.lvlib\\Beam Dump 2 (nA)"() -> (w1389:sgl)  [unwired: 1 in, 1 out]
                  n463 = shared-variable ".\\Zeiss Library.lvlib\\Milling I (nA)"() -> (w1388:sgl)  [unwired: 1 in, 1 out]
                  n464 = local read "SEM Spec. I (nA)"() -> (w1424:sgl)
                  n465 = shared-variable "My Computer\\Zeiss Library.lvlib\\FIB Slice #"() -> (w1421:u32)  [unwired: 1 in, 1 out]
                  n466 = shared-variable ".\\Zeiss Library.lvlib\\Milling Z Voltage RT"() -> (w1423:sgl)  [unwired: 1 in, 1 out]
                  n467 = local read "X Grids"() -> (w1372:u8)
                  n468 = local read "Y Grids"() -> (w1371:u8)
                  n469 = local read "File name"() -> (w1477:path)
                  n470 = local read "keep aspect ratio"() -> (w1382:bool)
                  n471 = local read "X resolution"() -> (w1369:u32)
                  n472 = local read "Y resolution"() -> (w1368:u32)
                  n473 = Multiply(x=w1372, y=w1371) -> (x*y=w1467:u8)
                  n474 = Less Or Equal?(x=w1467, y=u8 10) -> (x <= y?=w1466:bool)
                  n475 = Select(t=u32 1048576 ("Cropped to area pixels"), s=w1466, f=u32 262144 ("Cropped to area pixels")) -> (s? t:f=w1463:u32)
                  n476 = local read "Notes"() -> (w1516:string)
                  n477 = Open/Create/Replace File(file path (use dialog)=w1477, operation (0:open)=T16."replace or create") -> (refnum out=w1541:refnum<file>, error out=w1540:errorcluster)  [unwired: 1 in, 4 out]
                  n478 = Initialize Array(0.0 ("element"), 128 ("dimension size")) -> (w1537:dbl[])
                  n479 = Concatenate Strings(w1514, w1516, w1514) -> (w1515:string)
                  n480 = Write to Binary File(file (use dialog)=w1541, data=w1537, error in=w1540, 5:FALSE ("prepend array or string size? (T)")) -> (refnum out=w1437:refnum<file>, error out=w1436:errorcluster)  [unwired: 3 out]
                  n481 = local read "Runsheet header array"() -> (w1415:string[])
                  n482 = local read "File path"() -> (w1418:path)
                  n483 = local read "Timestamp"() -> (w1417:timestamp)
                  n484 = local read "DetA-Rate"() -> (w1394:sgl)
                  n485 = local read "DetA-Scaling"() -> (w1396:sgl)
                  n486 = local read "DetA-k"() -> (w1393:sgl)
                  n487 = Initialize Array(i16 0 ("element"), w1375, w1375, w1375, w1375) -> (w1364:i16[][][][])
                  n488 = case shown="0, Default" "FI Detector" {
                    tunnel: [w1566 FALSE ("Detector A") FALSE ("Detector A") FALSE ("Detector A")] -> w1367
                    frame 0, Default {
                      n489 = local read "Detector A"() -> (w1566:bool)
                    }
                    frame 1 {
                    }
                    frame 2 {
                    }
                    frame 3 {
                    }
                  }
                  n490 = case shown="1" "FI Detector" {
                    tunnel: [FALSE ("Detector A") w1563 FALSE ("Detector A") FALSE ("Detector A")] -> w1461
                    frame 0, Default {
                    }
                    frame 1 {
                      n491 = local read "Detector B"() -> (w1563:bool)
                    }
                    frame 2 {
                    }
                    frame 3 {
                    }
                  }
                  n492 = Divide(x=w1394, y=w1392) -> (x/y=w1395:dbl)
                  n493 = local read "Detector A"() -> (w1482:bool)
                  n494 = local read "Detector B"() -> (w1483:bool)
                  n495 = Compound Arithmetic op=MULTIPLY(w1395, w1396, w1393) -> (w1391:dbl)
                  n496 = Set File Position(offset (in bytes) (0)=i64 1024, refnum=w1437, from (0:start)=enum16{"start", "end", "current"}."start", error in=w1436) -> (refnum out=w1544:refnum<file>, error out=w1543:errorcluster)
                  n497 = expression code="1/x**2"(w1391) -> (w1390:dbl)
                  n498 = local read "AI multiline"() -> (w1344:u16)
                  n499 = call "Proportional area crop.vi"("multiline"=w1344, "Cropped to area pixels"=w1463, "keep aspect ratio"=w1382, "Y grids"=w1371, "Y resolution"=w1368, "X grids"=w1372, "X resolution"=w1369) -> ("Y length"=w1373:u32, "X length"=w1366:u32, "Grid settings"=w1365:T26)  [unwired: 2 out]
                  n500 = Initialize Array(i16 0 ("element"), w1371, w1372, w1373, w1366) -> (w1363:i16[][][][])
                  n501 = Select(t=w1363, s=w1367, f=w1364) -> (s? t:f=w1361:i16[][][][])
                  n502 = Select(t=w1363, s=w1461, f=w1364) -> (s? t:f=w1358:i16[][][][])
                  n503 = Build Array(w1482, w1483) -> (w1484:bool[])
                  n504 = local read "8-bit"() -> (w1412:bool)
                  n505 = Boolean Array To Number(Boolean array=w1484) -> (number=w1481:u32)
                  n506 = while {
                    tunnel: w1544 -> [w1644]
                    tunnel: [w1642] -> w1435
                    tunnel: w1543 -> [w1641]
                    tunnel: [w1637] -> w1434
                    tunnel: w1502 -> [w1634]
                    tunnel: [w1633] -> w1453
                    tunnel: [w1630] -> w1501
                    tunnel: [w1629] -> w1500
                    tunnel: w1481 -> [w1605]
                    shift-right: [w1626] -> w1370
                    shift-left: w1361 -> [w1614]
                    shift-right: [w1610] -> w1362
                    shift-left: w1358 -> [w1611]
                    tunnel: w1366 -> [w1624]
                    tunnel: w1373 -> [w1615]
                    tunnel: w1461 -> [w1609]
                    tunnel: [w1624] -> w1353
                    tunnel: [w1615] -> w1352
                    tunnel: [w1606] -> w1360
                    tunnel: [w1609] -> w1356
                    tunnel: w1412 -> [w1622]
                    shift-right: [w1616] -> _
                    shift-left: u16 0 -> [w1602]
                    tunnel: w1344 -> [w1603]
                    tunnel: w1367 -> [w1606]
                    shift-right: [w1612] -> _
                    shift-left: w1357 -> [w1613]
                    tunnel: w1365 -> [w1604]
                    shift-right: [w1607] -> _
                    shift-left: w1357 -> [w1608]
                    stop <- w1638 stop-if-true
                    n507 = Dequeue Element(queue=w1634) -> (queue out=w1630:refnum<queue>, element=w1621:i16[], error out=w1629:errorcluster)  [unwired: 1 in, 2 out]
                    n508 = local read "Y resolution"() -> (w1617:u32)
                    n509 = case shown="3" w1605 {
                      tunnel: w1621 -> [w1657 w1658 w1661]
                      tunnel: [w1657 _ w1660] -> w1627
                      tunnel: [_ w1658 w1659] -> w1625
                      frame 1, Default {
                      }
                      frame 2 {
                      }
                      frame 3 {
                        n510 = Decimate 1D Array(w1661) -> (w1660:i16[], w1659:i16[])
                      }
                    }
                    n511 = Add(x=w1602, y=w1603) -> (x+y=w1616:u16)
                    n512 = In Range and Coerce(upper limit=u8 255 ("offset (in bytes) (0)"), x=w1621, lower limit=u8 0 ("offset (in bytes) (0)")) -> (coerced(x)=w1620:i16[])  [unwired: 1 out]
                    n513 = Greater Or Equal?(x=w1616, y=w1617) -> (x >= y?=w1631:bool)
                    n514 = To Unsigned Byte Integer(number=w1620) -> (unsigned 8bit integer=w1623:u8[])
                    n515 = local read "Save"() -> (w1636:bool)
                    n516 = case shown="True" w1622 {
                      tunnel: w1644 -> [w1649 w1655]
                      tunnel: [w1648 w1654] -> w1643
                      tunnel: w1641 -> [w1647 w1653]
                      tunnel: [w1646 w1652] -> w1640
                      tunnel: w1623 -> [_ w1651]
                      tunnel: w1621 -> [w1645 _]
                      frame False {
                        n517 = Write to Binary File(file (use dialog)=w1649, data=w1645, error in=w1647, 5:FALSE ("prepend array or string size? (T)")) -> (refnum out=w1648:refnum<file>, error out=w1646:errorcluster)  [unwired: 3 out]
                      }
                      frame True {
                        n518 = Write to Binary File(file (use dialog)=w1655, data=w1651, error in=w1653, 5:FALSE ("prepend array or string size? (T)")) -> (refnum out=w1654:refnum<file>, error out=w1652:errorcluster)  [unwired: 3 out]
                      }
                    }
                    n519 = call "Scan lines to grid area.vi"("Enable"=w1606, "Grid settings"=w1604, "Multilines"=w1603, "Y line in"=w1613, "Y scan line"=w1602, "Multi-line scan"=w1627, "Input array"=w1614) -> ("Y line out"=w1612:u32, "Ouput array"=w1626:i16[][][][])  [unwired: 3 in]
                    n520 = call "Scan lines to grid area.vi"("Enable"=w1609, "Grid settings"=w1604, "Y line in"=w1608, "Multi-line scan"=w1625, "Input array"=w1611) -> ("Y line out"=w1607:u32, "Ouput array"=w1610:i16[][][][])  [unwired: 5 in]
                    n521 = local read "stop"() -> (w1628:bool)
                    n522 = Unbundle By Name(w1629) -> ("status"=w1632:bool)
                    n523 = Not(x=w1636) -> (.not. x?=w1635:bool)
                    n524 = Get File Position(4:w1640, 7:w1643) -> (0:w1637:errorcluster, 2:w1633:i64, 3:w1642:refnum<file>)
                    n525 = Unbundle By Name(w1637) -> ("status"=w1639:bool)
                    n526 = Compound Arithmetic op=OR(w1639, w1632, w1635, w1631, w1628) -> (w1638:bool)
                  }
                  n527 = local read "X Grids"() -> (w1355:u8)
                  n528 = local read "Y Grids"() -> (w1354:u8)
                  n529 = local read "Pixel size (nm)"() -> (w1387:sgl)
                  n530 = local read "Primary X index"() -> (w1381:u8)
                  n531 = local read "Primary Y index"() -> (w1380:u8)
                  n532 = shared-variable ".\\Zeiss Library.lvlib\\Recipe input"() -> (w1452:variant)  [unwired: 1 in, 1 out]
                  n533 = Less?(x=w1387, y=sgl 4.0) -> (x < y?=w1385:bool)
                  n534 = In Range and Coerce(upper limit=w1355, x=w1381, lower limit=w1470) -> (coerced(x)=w1350:u8)  [unwired: 1 out]
                  n535 = In Range and Coerce(upper limit=w1354, x=w1380, lower limit=w1470) -> (coerced(x)=w1351:u8)  [unwired: 1 out]
                  n536 = Select(t=TRUE ("prepend array or string size? (T)"), s=w1385, f=FALSE ("prepend array or string size? (T)")) -> (s? t:f=w1359:bool)
                  n537 = case shown="True" w1360 {
                    tunnel: w1353 -> [_ w1601]
                    tunnel: w1352 -> [_ w1600]
                    tunnel: w1355 -> [_ w1599]
                    tunnel: w1354 -> [_ w1598]
                    tunnel: [w1586 w1595] -> w1473
                    tunnel: w1350 -> [_ w1594]
                    tunnel: w1351 -> [_ w1593]
                    tunnel: [sgl[][] [] ("Focus index array") w1592] -> w1471
                    tunnel: [w1586 w1591] -> w1403
                    tunnel: [w1586 w1590] -> w1402
                    tunnel: w1359 -> [_ w1589]
                    tunnel: w1370 -> [_ w1588]
                    frame False {
                      w1586 = sgl 0.0 ("Focus index")
                    }
                    frame True {
                      n538 = call "Focus Index by Grids.vi"("Input array"=w1588, "Primary X index"=w1594, "X grids"=w1599, "Pre-bin 2"=w1589, "Y grids"=w1598, "X length"=w1601, "Y length"=w1600, "Primary Y index"=w1593) -> ("Focus index array"=w1592:sgl[][], "Primary FI"=w1595:sgl, "Primary eval area mean"=w1591:sgl, "Primary eval area std"=w1590:sgl, "Primary eval area"=w1597:dbl[][])  [unwired: 3 in]
                      n539 = To Word Integer(number=w1597) -> (16bit integer=→"Eval A":i16[][])
                    }
                  }
                  n540 = case shown="True" w1356 {
                    tunnel: w1353 -> [_ w1585]
                    tunnel: w1352 -> [_ w1584]
                    tunnel: w1355 -> [_ w1583]
                    tunnel: w1354 -> [_ w1582]
                    tunnel: [w1570 w1580] -> w1469
                    tunnel: w1350 -> [_ w1579]
                    tunnel: w1351 -> [_ w1578]
                    tunnel: [sgl[][] [] ("Focus index array") w1577] -> w1468
                    tunnel: [w1570 w1575] -> w1401
                    tunnel: [w1570 w1574] -> w1400
                    tunnel: w1359 -> [_ w1573]
                    tunnel: w1362 -> [_ w1572]
                    frame False {
                      w1570 = sgl 0.0 ("Focus index")
                    }
                    frame True {
                      n541 = call "Focus Index by Grids.vi"("Input array"=w1572, "Primary X index"=w1579, "X grids"=w1583, "Pre-bin 2"=w1573, "Y grids"=w1582, "X length"=w1585, "Y length"=w1584, "Primary Y index"=w1578) -> ("Focus index array"=w1577:sgl[][], "Primary FI"=w1580:sgl, "Primary eval area mean"=w1575:sgl, "Primary eval area std"=w1574:sgl, "Primary eval area"=w1581:dbl[][])  [unwired: 3 in]
                      n542 = To Word Integer(number=w1581) -> (16bit integer=→"Eval B":i16[][])
                    }
                  }
                  n543 = local read "Image Focus Index Array"() -> (w1472:T3)
                  n544 = local read "8-bit"() -> (w1408:bool)
                  n545 = local read "FI scaling"() -> (w1406:u8)
                  n546 = Bundle(cluster=w1472, "A Img Focus Index array"=w1471, "B Img Focus Index array"=w1468) -> (w1460:T3)  [unwired: 2 in]
                  n547 = local read "Image Focus Index"() -> (w1480:T4)
                  n548 = Select(t=w1390, s=w1408, f=1.0) -> (s? t:f=w1407:dbl)
                  n549 = Multiply(x=w1406, y=w1407) -> (x*y=w1405:dbl)
                  n550 = Multiply(x=w1460, y=w1405) -> (x*y=w1414:T27)
                  "Image Focus Index Array" <- w1414
                  n551 = Bundle(cluster=w1480, "A Img Focus Index"=w1473, "B Img Focus Index"=w1469) -> (w1459:T4)  [unwired: 2 in]
                  n552 = To Variant(anything=w1414) -> (Variant=w1413:variant)
                  n553 = Multiply(x=w1405, y=w1459) -> (x*y=w1429:T28)
                  "Image Focus Index" <- w1429
                  n554 = Unbundle By Name(w1429) -> ("A Img Focus Index"=w1479:dbl, "B Img Focus Index"=w1478:dbl)
                  n555 = case shown="0, Default" "FI Detector" {
                    tunnel: w1429 -> [w1549 w1551 w1553 w1555]
                    tunnel: [w1548 w1550 w1552 w1554] -> w1422
                    frame 0, Default {
                      n556 = Unbundle By Name(w1549) -> ("A Img Focus Index"=w1548:dbl)
                    }
                    frame 1 {
                      n557 = Unbundle By Name(w1551) -> ("B Img Focus Index"=w1550:dbl)
                    }
                    frame 2 {
                      n558 = Unbundle By Name(w1553) -> ("C Img Focus Index"=w1552:dbl)
                    }
                    frame 3 {
                      n559 = Unbundle By Name(w1555) -> ("D Img Focus Index"=w1554:dbl)
                    }
                  }
                  n560 = Build Array(w1517, w1518, w1519, w1520, w1499, w1498, w1509, w1510, w1497, w1496, w1495, w1494, w1493, w1492, w1491, w1486, w1485, w1490, w1489, w1488, w1487, w1378, w1479, w1478, w1343, w1343, w1403, w1402, w1401, w1400) -> (w1522:dbl[])
                  n561 = Bundle("Single"=w1428, "Single"=w1427, "Single"=w1426, "Single"=w1425, "Single"=w1389, "Single"=w1388, "SEM Spec. I (nA)"=w1424, "Single"=w1423, "D Img Focus Index"=w1422, "UInt32"=w1421) -> (w1420:T29)  [unwired: 1 out]
                  n562 = Bundle(w1439, "8-bit"=w1409, "8-bit coefficents"=w1410, "Restart flag"=w1348, "Stage move flag"=w1347, "First pixel X"=w1346, "First pixel Y"=w1345, w1451, w1450, "Decimating factor"=w1419, "Sample ID"=w1349, "Notes"=w1449, w1448, "SEM parameters"=w1445, "FIB parameters"=w1447, "Milling para"="Milling para", "Machine ID"=w1446, w1420) -> (w1438:T30)  [unwired: 1 in]
                  n563 = Array To Spreadsheet String(delimiter (Tab)=",", array=w1522, 3:"%#g" ("format string")) -> (spreadsheet string=w1513:string)
                  n564 = Scan String For Tokens(9:w1513) -> (1:w1505:string)  [unwired: 1 in, 7 out]
                  n565 = Build Array(w1515, w1512, w1511, w1503, w1504, w1505) -> (w1416:string[])
                  n566 = call "YMD log files.vi"("Input text array"=w1416, "Input header array"=w1415, "current time"=w1417, "Log file path"=w1418) -> ()  [unwired: 8 in]
                  n567 = call "Zeiss File Header Tclk.vi"("error in"=w1434, "Inputs"=w1438, "refnum"=w1435) -> ("error out"=w1430:errorcluster, "dup refnum"=w1431:refnum<file>)  [unwired: 6 in, 1 out]
                  n568 = Set File Position(offset (in bytes) (0)=i64 1000, refnum=w1431, error in=w1430) -> (refnum out=w1531:refnum<file>, error out=w1530:errorcluster)  [unwired: 1 in]
                  n569 = Write to Binary File(file (use dialog)=w1531, data=w1453, error in=w1530, 5:FALSE ("prepend array or string size? (T)")) -> (refnum out=w1455:refnum<file>, error out=w1454:errorcluster)  [unwired: 3 out]
                  n570 = Set File Position(offset (in bytes) (0)=w1453, refnum=w1455, error in=w1454) -> (refnum out=w1456:refnum<file>, error out=w1457:errorcluster)  [unwired: 1 in]
                  n571 = Write to Binary File(file (use dialog)=w1456, data=w1452, error in=w1457, 5:FALSE ("prepend array or string size? (T)")) -> (refnum out=w1433:refnum<file>, error out=w1432:errorcluster)  [unwired: 3 out]
                  n572 = Close File(refnum=w1433, error in=w1432) -> (error out=w1536:errorcluster)  [unwired: 1 out]
                  n573 = shared-variable ".\\Zeiss Library.lvlib\\Focus Index Array"(w1413) -> ()  [unwired: 1 in, 1 out]
                  n574 = call <vilib>:"General Error Handler.vi"("type of dialog (OK msg:1)"=w1535, "error in (no error)"=w1536) -> ()  [unwired: 1 in, 13 out]
                }
                frame True {
                  n575 = Wait on Occurrence(2:w1662) -> ()  [unwired: 2 in, 1 out]
                }
              }
            }
            frame #3 {
              n576 = local read "Display"() -> (w1664:bool)
              n577 = case shown="True" w1664 {
                tunnel: w1663 -> [_ w1683]
                frame False {
                }
                frame True {
                  w1740 = "%s, B&C = %#u\\% & %#u\\%, Max/Mean/Min = %#g / %#g / %#g, Focus Index = %^_3e" ("format string")
                  n578 = local read "Detector A"() -> (w1734:bool)
                  n579 = local read "Detector B"() -> (w1733:bool)
                  n580 = local read "Det B Img"() -> (w1711:i16[][])
                  n581 = local read "Detector A"() -> (w1708:bool)
                  n582 = local read "Detector C"() -> (w1707:bool)
                  n583 = local read "Detector D"() -> (w1704:bool)
                  n584 = local read "Det A Img"() -> (w1710:i16[][])
                  n585 = local read "Detector B"() -> (w1705:bool)
                  n586 = case shown="True" w1734 {
                    tunnel: [u8[][] [] w1825] -> w1712
                    tunnel: [_ w1828] -> w1679
                    tunnel: [_ w1827] -> w1678
                    tunnel: [_ w1826] -> w1677
                    tunnel: [_ w1830] -> w1719
                    frame False {
                    }
                    frame True {
                      n587 = local read "Det A Img"() -> (w1829:i16[][])
                      n588 = local read "Image Focus Index"() -> (w1831:T4)
                      n589 = call "16bit Image Normalization.vi"("Input image"=w1829) -> ("min"=w1826:i16, "mean"=w1827:i16, "max"=w1828:i16, "Normalized image"=w1825:u8[][])  [unwired: 6 in, 1 out]
                      n590 = Unbundle By Name(w1831) -> ("A Img Focus Index"=w1830:sgl)
                    }
                  }
                  n591 = case shown="True" w1733 {
                    tunnel: [u8[][] [] w1821] -> w1727
                    tunnel: [_ w1820] -> w1676
                    tunnel: [_ w1819] -> w1675
                    tunnel: [_ w1818] -> w1674
                    tunnel: [_ w1822] -> w1720
                    frame False {
                    }
                    frame True {
                      n592 = local read "Det B Img"() -> (w1817:i16[][])
                      n593 = local read "Image Focus Index"() -> (w1823:T4)
                      n594 = call "16bit Image Normalization.vi"("Input image"=w1817) -> ("min"=w1818:i16, "mean"=w1819:i16, "max"=w1820:i16, "Normalized image"=w1821:u8[][])  [unwired: 6 in, 1 out]
                      n595 = Unbundle By Name(w1823) -> ("B Img Focus Index"=w1822:sgl)
                    }
                  }
                  n596 = Build Array(w1734, w1733) -> (w1732:bool[])
                  n597 = Build Array(w1708, w1705, w1707, w1704) -> (w1706:bool[])
                  n598 = Boolean Array To Number(Boolean array=w1732) -> (number=w1743:u32)
                  n599 = Boolean Array To Number(Boolean array=w1706) -> (number=w1709:u32)
                  n600 = case shown="3" w1709 {
                    tunnel: w1710 -> [w1788 _ w1790]
                    tunnel: w1711 -> [_ w1789 _]
                    tunnel: [w1788 w1789 w1790] -> w1703
                    frame 1, Default {
                    }
                    frame 2 {
                    }
                    frame 3 {
                    }
                  }
                  n601 = local read "Image bits"() -> (w1701:u8)
                  n602 = local read "Inverse PNG"() -> (w1700:bool)
                  n603 = case shown="True" w1700 {
                    tunnel: [u32[] [16777222, 65793, 131586, 197379, 263172, 328965, 394758, 460551, 526344, 592137, 657930, 723723, 789516, 855309, 921102, 986895, 1052688, 1118481, 1184274, 1250067, 1315860, 1381653, 1447446, 1513239, 1579032, 1644825, 1710618, 1776411, 1842204, 1907997, 1973790, 2039583, 2105376, 2171169, 2236962, 2302755, 2368548, 2434341, 2500134, 2565927, 2631720, 2697513, 2763306, 2829099, 2894892, 2960685, 3026478, 3092271, 3158064, 3223857, 3289650, 3355443, 3421236, 3487029, 3552822, 3618615, 3684408, 3750201, 3815994, 3881787, 3947580, 4013373, 4079166, 4144959, 4210752, 4276545, 4342338, 4408131, 4473924, 4539717, 4605510, 4671303, 4737096, 4802889, 4868682, 4934475, 5000268, 5066061, 5131854, 5197647, 5263440, 5329233, 5395026, 5460819, 5526612, 5592405, 5658198, 5723991, 5789784, 5855577, 5921370, 5987163, 6052956, 6118749, 6184542, 6250335, 6316128, 6381921, 6447714, 6513507, 6579300, 6645093, 6710886, 6776679, 6842472, 6908265, 6974058, 7039851, 7105644, 7171437, 7237230, 7303023, 7368816, 7434609, 7500402, 7566195, 7631988, 7697781, 7763574, 7829367, 7895160, 7960953, 8026746, 8092539, 8158332, 8224125, 8289918, 8355711, 8421504, 8487297, 8553090, 8618883, 8684676, 8750469, 8816262, 8882055, 8947848, 9013641, 9079434, 9145227, 9211020, 9276813, 9342606, 9408399, 9474192, 9539985, 9605778, 9671571, 9737364, 9803157, 9868950, 9934743, 10000536, 10066329, 10132122, 10197915, 10263708, 10329501, 10395294, 10461087, 10526880, 10592673, 10658466, 10724259, 10790052, 10855845, 10921638, 10987431, 11053224, 11119017, 11184810, 11250603, 11316396, 11382189, 11447982, 11513775, 11579568, 11645361, 11711154, 11776947, 11842740, 11908533, 11974326, 12040119, 12105912, 12171705, 12237498, 12303291, 12369084, 12434877, 12500670, 12566463, 12632256, 12698049, 12763842, 12829635, 12895428, 12961221, 13027014, 13092807, 13158600, 13224393, 13290186, 13355979, 13421772, 13487565, 13553358, 13619151, 13684944, 13750737, 13816530, 13882323, 13948116, 14013909, 14079702, 14145495, 14211288, 14277081, 14342874, 14408667, 14474460, 14540253, 14606046, 14671839, 14737632, 14803425, 14869218, 14935011, 15000804, 15066597, 15132390, 15198183, 15263976, 15329769, 15395562, 15461355, 15527148, 15592941, 15658734, 15724527, 15790320, 15856113, 15921906, 15987699, 16053492, 16119285, 16185078, 16250871, 16316664, 16382457, 16448250, 16514043, 16579836, 16645629, 16711422, 16448250] ("256 gray scale") u32[] [16448250, 16711422, 16645629, 16579836, 16514043, 16448250, 16382457, 16316664, 16250871, 16185078, 16119285, 16053492, 15987699, 15921906, 15856113, 15790320, 15724527, 15658734, 15592941, 15527148, 15461355, 15395562, 15329769, 15263976, 15198183, 15132390, 15066597, 15000804, 14935011, 14869218, 14803425, 14737632, 14671839, 14606046, 14540253, 14474460, 14408667, 14342874, 14277081, 14211288, 14145495, 14079702, 14013909, 13948116, 13882323, 13816530, 13750737, 13684944, 13619151, 13553358, 13487565, 13421772, 13355979, 13290186, 13224393, 13158600, 13092807, 13027014, 12961221, 12895428, 12829635, 12763842, 12698049, 12632256, 12566463, 12500670, 12434877, 12369084, 12303291, 12237498, 12171705, 12105912, 12040119, 11974326, 11908533, 11842740, 11776947, 11711154, 11645361, 11579568, 11513775, 11447982, 11382189, 11316396, 11250603, 11184810, 11119017, 11053224, 10987431, 10921638, 10855845, 10790052, 10724259, 10658466, 10592673, 10526880, 10461087, 10395294, 10329501, 10263708, 10197915, 10132122, 10066329, 10000536, 9934743, 9868950, 9803157, 9737364, 9671571, 9605778, 9539985, 9474192, 9408399, 9342606, 9276813, 9211020, 9145227, 9079434, 9013641, 8947848, 8882055, 8816262, 8750469, 8684676, 8618883, 8553090, 8487297, 8421504, 8355711, 8289918, 8224125, 8158332, 8092539, 8026746, 7960953, 7895160, 7829367, 7763574, 7697781, 7631988, 7566195, 7500402, 7434609, 7368816, 7303023, 7237230, 7171437, 7105644, 7039851, 6974058, 6908265, 6842472, 6776679, 6710886, 6645093, 6579300, 6513507, 6447714, 6381921, 6316128, 6250335, 6184542, 6118749, 6052956, 5987163, 5921370, 5855577, 5789784, 5723991, 5658198, 5592405, 5526612, 5460819, 5395026, 5329233, 5263440, 5197647, 5131854, 5066061, 5000268, 4934475, 4868682, 4802889, 4737096, 4671303, 4605510, 4539717, 4473924, 4408131, 4342338, 4276545, 4210752, 4144959, 4079166, 4013373, 3947580, 3881787, 3815994, 3750201, 3684408, 3618615, 3552822, 3487029, 3421236, 3355443, 3289650, 3223857, 3158064, 3092271, 3026478, 2960685, 2894892, 2829099, 2763306, 2697513, 2631720, 2565927, 2500134, 2434341, 2368548, 2302755, 2236962, 2171169, 2105376, 2039583, 1973790, 1907997, 1842204, 1776411, 1710618, 1644825, 1579032, 1513239, 1447446, 1381653, 1315860, 1250067, 1184274, 1118481, 1052688, 986895, 921102, 855309, 789516, 723723, 657930, 592137, 526344, 460551, 394758, 328965, 263172, 197379, 131586, 65793, 16777222] ("256 gray scale inverse")] -> w1699
                    frame False {
                    }
                    frame True {
                    }
                  }
                  n604 = call "16bit Image Normalization.vi"("Transpose"=FALSE, "Imput image bits"=w1701, "Input image"=w1703) -> ("Direct scaled image"=w1689:u8[][])  [unwired: 4 in, 4 out]
                  n605 = local read "Inverse PNG"() -> (w1673:bool)
                  n606 = local read "PNG only"() -> (w1697:bool)
                  n607 = call <vilib>:"Flatten Pixmap.vi"("colors"=w1699, "8-bit pixmap"=w1689) -> ("image data"=w1698:T31)  [unwired: 4 in, 5 out]
                  n608 = Build Array (concatenate)(w1712, w1727) -> (w1718:u8[][])
                  n609 = shared-variable "My Computer\\Zeiss Library.lvlib\\DetB Max"(w1676) -> ()  [unwired: 1 in, 1 out]
                  n610 = shared-variable "My Computer\\Zeiss Library.lvlib\\DetB Mean"(w1675) -> ()  [unwired: 1 in, 1 out]
                  n611 = shared-variable "My Computer\\Zeiss Library.lvlib\\DetB Min"(w1674) -> ()  [unwired: 1 in, 1 out]
                  n612 = case shown="False" w1697 {
                    tunnel: w1698 -> [w1785 _]
                    frame False {
                      n613 = local read "Tile index"() -> (w1782:u8[])
                      n614 = Index Array(array=w1782) -> (element #1=w1783:u8, element #2=w1784:u8)  [unwired: 2 in]
                      n615 = Format Into String(w1783) -> (resulting string=w1781:string)  [unwired: 3 in, 1 out]
                      n616 = Format Into String(w1784) -> (resulting string=w1779:string)  [unwired: 3 in, 1 out]
                      n617 = Concatenate Strings("Low res_" ("string"), w1781, "-" ("string"), w1779, ".png" ("string")) -> (w1775:string)
                      n618 = Build Path(base path=path "D:/3D FIB-SEM Files" ("path to PNG file"), name or relative path=w1775) -> (appended path=w1774:path)
                      n619 = call <vilib>:"Write PNG File.vi"("image data"=w1785, "path to PNG file"=w1774) -> ()  [unwired: 1 in, 9 out]
                    }
                    frame True {
                    }
                  }
                  n620 = Select(t=u8 255 ("element"), s=w1673, f=u8 0 ("element")) -> (s? t:f=w1672:u8)
                  n621 = Transpose 2D Array(2D array=w1718) -> (transposed array=w1763:u8[][])
                  n622 = local read "FI Detector"() -> (w1682:u16)
                  n623 = local read "Eval A"() -> (w1716:i16[][])
                  n624 = local read "Eval B"() -> (w1717:i16[][])
                  n625 = shared-variable "My Computer\\Zeiss Library.lvlib\\DetA Max"(w1679) -> ()  [unwired: 1 in, 1 out]
                  n626 = local read "PNG only"() -> (w1667:bool)
                  n627 = shared-variable "My Computer\\Zeiss Library.lvlib\\DetA Mean"(w1678) -> ()  [unwired: 1 in, 1 out]
                  n628 = shared-variable "My Computer\\Zeiss Library.lvlib\\DetA Min"(w1677) -> ()  [unwired: 1 in, 1 out]
                  n629 = local read "SEM parameters"() -> (w1735:T5)
                  n630 = Unbundle By Name(w1735) -> ("Detector A"=w1739:string, "Brightness A"=w1722:sgl, "Contrast A"=w1721:sgl, "Detector B"=w1736:string, "Brightness B"=w1737:sgl, "Contrast B"=w1738:sgl)
                  n631 = local read "Image bits"() -> (w1713:u8)
                  n632 = case shown="1" w1682 {
                    tunnel: w1716 -> [w1810 _]
                    tunnel: w1717 -> [_ w1811]
                    tunnel: [w1810 w1811] -> w1685
                    frame 0, Default {
                    }
                    frame 1 {
                    }
                  }
                  n633 = Array Size(array=w1685) -> (size(s)=w1766:i32[])
                  n634 = Index Array(array=w1766, index=1) -> (element=w1669:i32)
                  n635 = Select(t=1024, s=w1667, f=w1669) -> (s? t:f=w1668:i32)
                  n636 = local read "Inverse PNG"() -> (w1693:bool)
                  n637 = Initialize Array(w1672, 60 ("dimension size"), w1668) -> (w1764:u8[][])
                  n638 = Format Into String(format string=w1740, w1739, w1722, w1721, w1679, w1678, w1677, w1719) -> (resulting string=w1742:string)  [unwired: 2 in, 1 out]
                  n639 = Format Into String(format string=w1740, w1736, w1737, w1738, w1676, w1675, w1674, w1720) -> (resulting string=w1741:string)  [unwired: 2 in, 1 out]
                  n640 = call "16bit Image Normalization.vi"("Transpose"=FALSE, "Imput image bits"=w1713, "Input image"=w1685) -> ("Normalized image"=w1686:u8[][], "Direct scaled image"=w1684:u8[][])  [unwired: 4 in, 3 out]
                  n641 = case shown="False" w1693 {
                    tunnel: [u32[] [16777222, 65793, 131586, 197379, 263172, 328965, 394758, 460551, 526344, 592137, 657930, 723723, 789516, 855309, 921102, 986895, 1052688, 1118481, 1184274, 1250067, 1315860, 1381653, 1447446, 1513239, 1579032, 1644825, 1710618, 1776411, 1842204, 1907997, 1973790, 2039583, 2105376, 2171169, 2236962, 2302755, 2368548, 2434341, 2500134, 2565927, 2631720, 2697513, 2763306, 2829099, 2894892, 2960685, 3026478, 3092271, 3158064, 3223857, 3289650, 3355443, 3421236, 3487029, 3552822, 3618615, 3684408, 3750201, 3815994, 3881787, 3947580, 4013373, 4079166, 4144959, 4210752, 4276545, 4342338, 4408131, 4473924, 4539717, 4605510, 4671303, 4737096, 4802889, 4868682, 4934475, 5000268, 5066061, 5131854, 5197647, 5263440, 5329233, 5395026, 5460819, 5526612, 5592405, 5658198, 5723991, 5789784, 5855577, 5921370, 5987163, 6052956, 6118749, 6184542, 6250335, 6316128, 6381921, 6447714, 6513507, 6579300, 6645093, 6710886, 6776679, 6842472, 6908265, 6974058, 7039851, 7105644, 7171437, 7237230, 7303023, 7368816, 7434609, 7500402, 7566195, 7631988, 7697781, 7763574, 7829367, 7895160, 7960953, 8026746, 8092539, 8158332, 8224125, 8289918, 8355711, 8421504, 8487297, 8553090, 8618883, 8684676, 8750469, 8816262, 8882055, 8947848, 9013641, 9079434, 9145227, 9211020, 9276813, 9342606, 9408399, 9474192, 9539985, 9605778, 9671571, 9737364, 9803157, 9868950, 9934743, 10000536, 10066329, 10132122, 10197915, 10263708, 10329501, 10395294, 10461087, 10526880, 10592673, 10658466, 10724259, 10790052, 10855845, 10921638, 10987431, 11053224, 11119017, 11184810, 11250603, 11316396, 11382189, 11447982, 11513775, 11579568, 11645361, 11711154, 11776947, 11842740, 11908533, 11974326, 12040119, 12105912, 12171705, 12237498, 12303291, 12369084, 12434877, 12500670, 12566463, 12632256, 12698049, 12763842, 12829635, 12895428, 12961221, 13027014, 13092807, 13158600, 13224393, 13290186, 13355979, 13421772, 13487565, 13553358, 13619151, 13684944, 13750737, 13816530, 13882323, 13948116, 14013909, 14079702, 14145495, 14211288, 14277081, 14342874, 14408667, 14474460, 14540253, 14606046, 14671839, 14737632, 14803425, 14869218, 14935011, 15000804, 15066597, 15132390, 15198183, 15263976, 15329769, 15395562, 15461355, 15527148, 15592941, 15658734, 15724527, 15790320, 15856113, 15921906, 15987699, 16053492, 16119285, 16185078, 16250871, 16316664, 16382457, 16448250, 16514043, 16579836, 16645629, 16711422, 16448250] ("256 gray scale") u32[] [16448250, 16711422, 16645629, 16579836, 16514043, 16448250, 16382457, 16316664, 16250871, 16185078, 16119285, 16053492, 15987699, 15921906, 15856113, 15790320, 15724527, 15658734, 15592941, 15527148, 15461355, 15395562, 15329769, 15263976, 15198183, 15132390, 15066597, 15000804, 14935011, 14869218, 14803425, 14737632, 14671839, 14606046, 14540253, 14474460, 14408667, 14342874, 14277081, 14211288, 14145495, 14079702, 14013909, 13948116, 13882323, 13816530, 13750737, 13684944, 13619151, 13553358, 13487565, 13421772, 13355979, 13290186, 13224393, 13158600, 13092807, 13027014, 12961221, 12895428, 12829635, 12763842, 12698049, 12632256, 12566463, 12500670, 12434877, 12369084, 12303291, 12237498, 12171705, 12105912, 12040119, 11974326, 11908533, 11842740, 11776947, 11711154, 11645361, 11579568, 11513775, 11447982, 11382189, 11316396, 11250603, 11184810, 11119017, 11053224, 10987431, 10921638, 10855845, 10790052, 10724259, 10658466, 10592673, 10526880, 10461087, 10395294, 10329501, 10263708, 10197915, 10132122, 10066329, 10000536, 9934743, 9868950, 9803157, 9737364, 9671571, 9605778, 9539985, 9474192, 9408399, 9342606, 9276813, 9211020, 9145227, 9079434, 9013641, 8947848, 8882055, 8816262, 8750469, 8684676, 8618883, 8553090, 8487297, 8421504, 8355711, 8289918, 8224125, 8158332, 8092539, 8026746, 7960953, 7895160, 7829367, 7763574, 7697781, 7631988, 7566195, 7500402, 7434609, 7368816, 7303023, 7237230, 7171437, 7105644, 7039851, 6974058, 6908265, 6842472, 6776679, 6710886, 6645093, 6579300, 6513507, 6447714, 6381921, 6316128, 6250335, 6184542, 6118749, 6052956, 5987163, 5921370, 5855577, 5789784, 5723991, 5658198, 5592405, 5526612, 5460819, 5395026, 5329233, 5263440, 5197647, 5131854, 5066061, 5000268, 4934475, 4868682, 4802889, 4737096, 4671303, 4605510, 4539717, 4473924, 4408131, 4342338, 4276545, 4210752, 4144959, 4079166, 4013373, 3947580, 3881787, 3815994, 3750201, 3684408, 3618615, 3552822, 3487029, 3421236, 3355443, 3289650, 3223857, 3158064, 3092271, 3026478, 2960685, 2894892, 2829099, 2763306, 2697513, 2631720, 2565927, 2500134, 2434341, 2368548, 2302755, 2236962, 2171169, 2105376, 2039583, 1973790, 1907997, 1842204, 1776411, 1710618, 1644825, 1579032, 1513239, 1447446, 1381653, 1315860, 1250067, 1184274, 1118481, 1052688, 986895, 921102, 855309, 789516, 723723, 657930, 592137, 526344, 460551, 394758, 328965, 263172, 197379, 131586, 65793, 16777222] ("256 gray scale inverse")] -> w1690
                    tunnel: [_ "Inverse"] -> w1688
                    tunnel: [u32 16448250 ("text color(black)") u32 0 ("text color(black)")] -> w1691
                    frame False {
                    }
                    frame True {
                    }
                  }
                  n642 = Unbundle By Name(w1735) -> ("Magnification"=w1726:sgl, "Pixel size"=w1725:sgl, "Working distance"=w1724:sgl, "EHT"=w1723:sgl)
                  n643 = case shown="False" w1667 {
                    tunnel: w1764 -> [w1806 w1809]
                    tunnel: w1763 -> [w1805 w1808]
                    tunnel: [w1804 w1807] -> w1762
                    tunnel: w1686 -> [w1803 _]
                    frame False {
                      n644 = Build Array (concatenate)(w1806, w1805, w1803) -> (w1804:u8[][])
                    }
                    frame True {
                      n645 = Build Array (concatenate)(w1809, w1808) -> (w1807:u8[][])
                    }
                  }
                  n646 = local read "File name"() -> (w1773:path)
                  n647 = case shown="3" w1743 {
                    tunnel: w1742 -> [w1812 _ w1815]
                    tunnel: w1741 -> [_ w1813 w1814]
                    tunnel: [w1812 w1813 w1815] -> w1729
                    tunnel: [_ _ w1814] -> w1728
                    frame 1, Default {
                    }
                    frame 2 {
                    }
                    frame 3 {
                    }
                  }
                  n648 = local read "Sample ID"() -> (w1687:string)
                  n649 = call <vilib>:"Flatten Pixmap.vi"("colors"=u32[] [16777222, 65793, 131586, 197379, 263172, 328965, 394758, 460551, 526344, 592137, 657930, 723723, 789516, 855309, 921102, 986895, 1052688, 1118481, 1184274, 1250067, 1315860, 1381653, 1447446, 1513239, 1579032, 1644825, 1710618, 1776411, 1842204, 1907997, 1973790, 2039583, 2105376, 2171169, 2236962, 2302755, 2368548, 2434341, 2500134, 2565927, 2631720, 2697513, 2763306, 2829099, 2894892, 2960685, 3026478, 3092271, 3158064, 3223857, 3289650, 3355443, 3421236, 3487029, 3552822, 3618615, 3684408, 3750201, 3815994, 3881787, 3947580, 4013373, 4079166, 4144959, 4210752, 4276545, 4342338, 4408131, 4473924, 4539717, 4605510, 4671303, 4737096, 4802889, 4868682, 4934475, 5000268, 5066061, 5131854, 5197647, 5263440, 5329233, 5395026, 5460819, 5526612, 5592405, 5658198, 5723991, 5789784, 5855577, 5921370, 5987163, 6052956, 6118749, 6184542, 6250335, 6316128, 6381921, 6447714, 6513507, 6579300, 6645093, 6710886, 6776679, 6842472, 6908265, 6974058, 7039851, 7105644, 7171437, 7237230, 7303023, 7368816, 7434609, 7500402, 7566195, 7631988, 7697781, 7763574, 7829367, 7895160, 7960953, 8026746, 8092539, 8158332, 8224125, 8289918, 8355711, 8421504, 8487297, 8553090, 8618883, 8684676, 8750469, 8816262, 8882055, 8947848, 9013641, 9079434, 9145227, 9211020, 9276813, 9342606, 9408399, 9474192, 9539985, 9605778, 9671571, 9737364, 9803157, 9868950, 9934743, 10000536, 10066329, 10132122, 10197915, 10263708, 10329501, 10395294, 10461087, 10526880, 10592673, 10658466, 10724259, 10790052, 10855845, 10921638, 10987431, 11053224, 11119017, 11184810, 11250603, 11316396, 11382189, 11447982, 11513775, 11579568, 11645361, 11711154, 11776947, 11842740, 11908533, 11974326, 12040119, 12105912, 12171705, 12237498, 12303291, 12369084, 12434877, 12500670, 12566463, 12632256, 12698049, 12763842, 12829635, 12895428, 12961221, 13027014, 13092807, 13158600, 13224393, 13290186, 13355979, 13421772, 13487565, 13553358, 13619151, 13684944, 13750737, 13816530, 13882323, 13948116, 14013909, 14079702, 14145495, 14211288, 14277081, 14342874, 14408667, 14474460, 14540253, 14606046, 14671839, 14737632, 14803425, 14869218, 14935011, 15000804, 15066597, 15132390, 15198183, 15263976, 15329769, 15395562, 15461355, 15527148, 15592941, 15658734, 15724527, 15790320, 15856113, 15921906, 15987699, 16053492, 16119285, 16185078, 16250871, 16316664, 16382457, 16448250, 16514043, 16579836, 16645629, 16711422, 16448250] ("256 gray scale"), "8-bit pixmap"=w1762) -> ("image data"=w1759:T31)  [unwired: 4 in, 5 out]
                  n650 = Strip Path(path=w1773) -> (stripped path=w1772:path, name=w1748:string)
                  n651 = call <vilib>:"Draw Flattened Pixmap.vi"("image data"=w1759) -> ("new picture"=w1761:picture)  [unwired: 1 in, 7 out]
                  n652 = Format Into String(format string="%s\n%s,  %s\nScan Rate = %.3pHz", w1748, w1687, w1688, w1683) -> (resulting string=w1747:string)  [unwired: 2 in, 1 out]
                  n653 = Search and Replace String(input string=w1748, search string=".dat", replace string=".png" ("replace string (\"\")")) -> (result string=w1769:string)  [unwired: 1 in, 7 out]
                  n654 = call <vilib>:"Draw Text at Point.vi"("text color(black)"=w1691, "text"=w1747, "origin"=cluster{"x":i16, "y":i16} {"x"=10, "y"=0}, "picture"=w1761) -> ("new picture"=w1750:picture)  [unwired: 5 in, 2 out]
                  n655 = local read "X resolution"() -> (w1751:u32)
                  n656 = local read "Y resolution"() -> (w1752:u32)
                  n657 = Build Path(base path=w1772, name or relative path=w1769) -> (appended path=w1768:path)
                  n658 = call <vilib>:"Flatten Pixmap.vi"("colors"=w1690, "8-bit pixmap"=w1684) -> ("image data"=w1715:T31)  [unwired: 4 in, 5 out]
                  n659 = case shown="False" w1667 {
                    tunnel: w1715 -> [w1791 _]
                    frame False {
                      n660 = local read "Tile index"() -> (w1800:u8[])
                      n661 = Index Array(array=w1800) -> (element #1=w1801:u8, element #2=w1802:u8)  [unwired: 2 in]
                      n662 = Format Into String(w1801) -> (resulting string=w1799:string)  [unwired: 3 in, 1 out]
                      n663 = Format Into String(w1802) -> (resulting string=w1797:string)  [unwired: 3 in, 1 out]
                      n664 = Concatenate Strings("Primary_grid_" ("string"), w1799, "-" ("string"), w1797, ".png" ("string")) -> (w1796:string)
                      n665 = Build Path(base path=path "D:/3D FIB-SEM Files" ("path to PNG file"), name or relative path=w1796) -> (appended path=w1792:path)
                      n666 = call <vilib>:"Write PNG File.vi"("image data"=w1791, "path to PNG file"=w1792) -> ()  [unwired: 1 in, 9 out]
                    }
                    frame True {
                    }
                  }
                  n667 = Format Into String(format string="Mag = %5.1f X\nPixel Size = %5.1f nm\n%#g x %#g pixels", w1726, w1725, w1751, w1752) -> (resulting string=w1746:string)  [unwired: 2 in, 1 out]
                  n668 = call <vilib>:"Draw Text at Point.vi"("text color(black)"=w1691, "text"=w1746, "origin"=cluster{"x":i16, "y":i16} {"x"=230, "y"=0}, "picture"=w1750) -> ("new picture"=w1758:picture)  [unwired: 5 in, 2 out]
                  n669 = local read "DetA-Scaling"() -> (w1681:sgl)
                  n670 = local read "DetB-Scaling"() -> (w1680:sgl)
                  n671 = Format Into String(format string="WD = %#g mm\nEHT = %#g kV\nDetA/B e- Scaling = %#g / %#g", w1724, w1723, w1681, w1680) -> (resulting string=w1754:string)  [unwired: 2 in, 1 out]
                  n672 = call <vilib>:"Draw Text at Point.vi"("text color(black)"=w1691, "text"=w1754, "origin"=cluster{"x":i16, "y":i16} {"x"=350, "y"=0}, "picture"=w1758) -> ("new picture"=w1731:picture)  [unwired: 5 in, 2 out]
                  n673 = call <vilib>:"Draw Text at Point.vi"("text color(black)"=w1691, "text"=w1729, "origin"=cluster{"x":i16, "y":i16} {"x"=10, "y"=45}, "picture"=w1731) -> ("new picture"=w1730:picture)  [unwired: 5 in, 2 out]
                  n674 = call <vilib>:"Draw Text at Point.vi"("text color(black)"=w1691, "text"=w1728, "origin"=cluster{"x":i16, "y":i16} {"x"=522, "y"=45}, "picture"=w1730) -> ("new picture"=w1665:picture)  [unwired: 5 in, 2 out]
                  n675 = call <vilib>:"Picture to Pixmap.vi"("picture"=w1665) -> ("image data"=w1695:T31)  [unwired: 3 in, 7 out]
                  n676 = call <vilib>:"Unflatten Pixmap.vi"("image data"=w1695) -> ("24-bit pixmap"=w1694:u32[][])  [unwired: 4 in, 6 out]
                  n677 = call <vilib>:"Flatten Pixmap.vi"("colors"=w1690, "8-bit pixmap"=w1694) -> ("image data"=w1696:T31)  [unwired: 4 in, 5 out]
                  n678 = call <vilib>:"Write PNG File.vi"("image data"=w1696, "path to PNG file"=w1768) -> ()  [unwired: 1 in, 9 out]
                }
              }
            }
            frame #4 {
              n679 = local read "Upload"() -> (w1837:bool)
              n680 = case shown="True" w1837 {
                frame False {
                }
                frame True {
                  n681 = stacked-sequence {
                    frame #0 {
                      n682 = shared-variable ".\\Zeiss Library.lvlib\\Upload flags path"() -> (w1838:string)  [unwired: 1 in, 1 out]
                      n683 = String To Path(string=w1838) -> (path=w1839:path)
                      "Upload flags path" <- w1839
                      n684 = File/Directory Info(path=w1839) -> (path out=w1842:path, error out=w1840:errorcluster)  [unwired: 1 in, 5 out]
                      n685 = Unbundle By Name(w1840) -> ("status"=w1841:bool)
                      n686 = case shown="True" w1841 {
                        tunnel: w1842 -> [_ w1843]
                        frame False {
                        }
                        frame True {
                          n687 = Create Folder(path (use dialog)=w1843) -> ()  [unwired: 1 in, 4 out]
                        }
                      }
                    }
                    frame #1 {
                      w1851 = T17 3 items=["no dialog", "OK message", "continue or stop message", "OK message + warnings", "continue/stop + warnings"] ("type of dialog (OK msg:1)")
                      w1863 = "^" ("replace string (\"\")")
                      n688 = local read "Upload flags path"() -> (w1854:path)
                      n689 = local read "File name"() -> (w1860:path)
                      n690 = local read "Delete after upload"() -> (w1847:bool)
                      n691 = Path To String(path=w1860) -> (string=w1859:string)
                      n692 = Select(t="^delete" ("replace string (\"\")"), s=w1847, f="^keep" ("replace string (\"\")")) -> (s? t:f=w1844:string)
                      n693 = Search and Replace String(replace all?=TRUE ("replace all? (F)"), input string=w1859, search string="\\", replace string=w1863) -> (result string=w1864:string)  [unwired: 4 in, 3 out]
                      n694 = local read "Sample ID"() -> (w1857:string)
                      n695 = Search and Replace String(input string=w1864, search string=":", replace string=w1863) -> (result string=w1856:string)  [unwired: 5 in, 3 out]
                      n696 = Concatenate Strings(w1857, "^" ("string"), w1856, w1844) -> (w1858:string)
                      n697 = Build Path(base path=w1854, name or relative path=w1858) -> (appended path=w1853:path)
                      n698 = Open/Create/Replace File(file path (use dialog)=w1853, operation (0:open)=T16."replace or create") -> (refnum out=w1850:refnum<file>, error out=w1848:errorcluster)  [unwired: 1 in, 4 out]
                      n699 = Close File(refnum=w1850, error in=w1848) -> (error out=w1849:errorcluster)  [unwired: 1 out]
                      n700 = call <vilib>:"General Error Handler.vi"("type of dialog (OK msg:1)"=w1851, "error in (no error)"=w1849) -> ()  [unwired: 1 in, 13 out]
                    }
                  }
                }
              }
            }
          }
        }
      }
      n701 = flat-sequence {
        tunnel: w791 -> [_]
        frame #0 {
          w944 = T17 3 items=["no dialog", "OK message", "continue or stop message", "OK message + warnings", "continue/stop + warnings"] ("type of dialog (OK msg:1)")
          w940 = 0 items=["one channel for each line", "one channel for all lines"] ("line grouping")
          n702 = shared-variable "My Computer\\Zeiss Library.lvlib\\Machine Type"() -> (w937:u8)  [unwired: 1 in, 1 out]
          n703 = case shown="2" w937 {
            frame 0, Default {
              n704 = local read "Eanable COM"() -> (w949:bool)
              n705 = case shown="True" w949 {
                frame False {
                }
                frame True {
                  w961 = TRUE ("Initialization")
                  n706 = local read "COM port"() -> (w958:refnum<visa-resource-name>)
                  n707 = call "Remcon32 command.vi"("Initialization"=w961, "SEM command"="bblk 1" ("write buffer"), "COM port in"=w958) -> ("error out"=w960:errorcluster, "COM port out"=w959:refnum<visa-resource-name>)  [unwired: 2 in, 5 out]
                  n708 = call "Remcon32 command.vi"("error in"=w960, "SEM command"="edx 0" ("write buffer"), "COM port in"=w959) -> ("error out"=w953:errorcluster, "COM port out"=w951:refnum<visa-resource-name>)  [unwired: 2 in, 5 out]
                  n709 = call "Remcon32 command.vi"("error in"=w953, "SEM command"="bblk 1" ("write buffer"), "COM port in"=w951) -> ("error out"=w954:errorcluster, "COM port out"=w952:refnum<visa-resource-name>)  [unwired: 2 in, 5 out]
                  n710 = local read "Freeze"() -> (w956:bool)
                  n711 = case shown="True" w956 {
                    tunnel: w952 -> [w964 w968]
                    tunnel: w961 -> [w962 w967]
                    tunnel: w954 -> [w963 w966]
                    frame False {
                      n712 = call "Remcon32 command.vi"("Close session"=w962, "error in"=w963, "COM port in"=w964) -> ()  [unwired: 2 in, 7 out]
                    }
                    frame True {
                      n713 = call "Remcon32 command.vi"("Close session"=w967, "error in"=w966, "SEM command"="frez" ("write buffer"), "COM port in"=w968) -> ()  [unwired: 1 in, 7 out]
                    }
                  }
                }
              }
            }
            frame 2 {
              n714 = local read "ActiveX Container"() -> (w978:refnum<k7>)
              n715 = local read "Freeze"() -> (w971:bool)
              n716 = invoke class="_EMApi" method="Set"(reference=w978, "lpszParam"="DP_BEAM_BLANKED", "vValue"=sgl 1.0) -> (reference out=w975:refnum<k7>, error out=w974:errorcluster)  [unwired: 2 in, 3 out]
              n717 = invoke class="_EMApi" method="Set"(reference=w975, error in=w974, "lpszParam"="DP_EXT_SCAN_CONTROL" ("lpszCommand"), "vValue"=sgl 0.0) -> (reference out=w970:refnum<k7>, error out=w969:errorcluster)  [unwired: 1 in, 3 out]
              n718 = case shown="True" w971 {
                tunnel: w970 -> [_ w980]
                tunnel: w969 -> [_ w979]
                frame False {
                }
                frame True {
                  n719 = invoke class="_EMApi" method="Execute"(reference=w980, error in=w979, "lpszCommand"="CMD_FREEZE_ALL") -> ()  [unwired: 1 in, 4 out]
                }
              }
            }
          }
          n720 = local read "Detector FIB-NI auto switch"() -> (w948:tag)
          n721 = call-poly <vilib>:"DAQmx Create Virtual Channel.vi"("lines"=w948, "line grouping"=w940) -> ("task out"=w938:refnum<k21>, "error out"=w939:errorcluster)  [unwired: 3 in, 9 out]
          n722 = call <vilib>:"DAQmx Start Task.vi"("task/channels in"=w938, "error in"=w939) -> ("task out"=w941:refnum<k21>, "error out"=w942:errorcluster)  [unwired: 12 out]
          n723 = call-poly <vilib>:"DAQmx Write.vi"("task/channels in"=w941, "data"=FALSE, "error in"=w942) -> ("task out"=w946:refnum<k21>, "error out"=w947:errorcluster)  [unwired: 1 in, 10 out]
          n724 = call <vilib>:"DAQmx Clear Task.vi"("task in"=w946, "error in"=w947) -> ("error out"=w945:errorcluster)  [unwired: 13 out]
          n725 = call <vilib>:"Simple Error Handler.vi"("type of dialog (OK msg:1)"=w944, "error in (no error)"=w945) -> ()  [unwired: 8 out]
        }
      }
      n726 = Get Queue Status(queue=w813, error in (no error)=w812) -> (queue out=w814:refnum<queue>, error out=w815:errorcluster, # elements in queue=w816:i32)  [unwired: 6 out]
      n727 = Merge Errors(w739, w791, w796) -> (w735:errorcluster)
      "error out" <- w735
      n728 = Equal To 0?(x=w816) -> (x = 0?=w817:bool)
      n729 = case shown="True" w802 {
        tunnel: w801 -> [_ w982]
        frame False {
        }
        frame True {
          n730 = Set Occurrence(w982) -> ()
        }
      }
      n731 = case shown="False" w826 {
        tunnel: w819 -> [w1867 _]
        tunnel: w818 -> [w1866 _]
        frame False {
          n732 = Release Queue(queue=w1867, error in (no error)=w1866) -> ()  [unwired: 4 out]
        }
        frame True {
        }
      }
      n733 = Compound Arithmetic op=OR(w817, w706) -> (w809:bool)
      n734 = call <vilib>:"Clear Errors.vi"("error in (no error)"=w735) -> ("error out"=w736:errorcluster)  [unwired: 5 in, 1 out]
      n735 = case shown="True" w809 {
        tunnel: w814 -> [_ w990]
        tunnel: w815 -> [w987 w989]
        tunnel: [w987 w988] -> _
        frame False {
        }
        frame True {
          n736 = Release Queue(queue=w990, error in (no error)=w989) -> (error out=w988:errorcluster)  [unwired: 3 out]
        }
      }
      n737 = call "FM Gen Pulse for FIB-SEM.vi"("WatchDog Mode"="WatchDog Mode", "error in"=w736, "State Value"=i16 5) -> ()  [unwired: 6 in, 3 out]
      n738 = case shown="False" w809 {
        tunnel: w811 -> [w986 _]
        tunnel: w810 -> [w985 _]
        frame False {
          n739 = Release Queue(queue=w986, error in (no error)=w985) -> ()  [unwired: 4 out]
        }
        frame True {
        }
      }
    }
    frame #3 {
      n740 = local read "Det A Img"() -> (w1907:i16[][])
      n741 = local read "Det B Img"() -> (w1901:i16[][])
      n742 = Array Size(array=w1907) -> (size(s)=w1905:i32[])
      n743 = Array Size(array=w1901) -> (size(s)=w1903:i32[])
      n744 = Multiply Array Elements(1:w1905) -> (0:w1906:i32)
      n745 = Multiply Array Elements(1:w1903) -> (0:w1902:i32)
      n746 = local read "Options"() -> (w1917:T9)
      n747 = Reshape Array(w1907, w1906) -> (w1908:i16[])
      n748 = Reshape Array(w1901, w1902) -> (w1900:i16[])
      n749 = Array Max & Min(array=w1908) -> (max value=w1904:i16)  [unwired: 3 out]
      n750 = Array Max & Min(array=w1900) -> (max value=w1899:i16)  [unwired: 3 out]
      n751 = Unbundle By Name(w1917) -> ("8-bit"=w1914:bool, "Detector A"=w1913:bool, "Detector B"=w1912:bool)
      n752 = Greater?(x=w1904, y=u8 255) -> (0:w1918:bool)
      n753 = Greater?(x=w1899, y=u8 255) -> (0:w1916:bool)
      n754 = Compound Arithmetic op=AND(w1914, w1913, w1918) -> (w1911:bool)
      n755 = Compound Arithmetic op=AND(w1914, w1912, w1916) -> (w1910:bool)
      n756 = Build Array(w1911, w1910) -> (→"8-bit over scale":bool[])
    }
    frame #4 {
      n757 = local read "Tile index"() -> (w1920:u8[])
      n758 = local write "stop"(TRUE ("stop")) -> ()
      n759 = local write "Force tclk init"(FALSE ("Force tclk init")) -> ()
      n760 = shared-variable ".\\Zeiss Library.lvlib\\Completed tile index"(w1920) -> ()  [unwired: 1 in, 1 out]
    }
  }
